vi "GetPropertiesArray.vi"(8 "error in (no error)":errorcluster, 11 "JSON Text":string="{\n    \"productNum\": 30929, \n    \"productName\": \"SLSC Module Prototype\",\n\n    \"vendorNum\": 4243, \n    \"vendorName\": \"National Instruments\",\n    \"vendorPrefix\": \"NI\",\n\n    \"capsVersion\": \"17.0.0f0\",\n    \"capsSpecVersion\": 2,\n    \"capsSpecOldestCompatibleVersion\": 1,\n\n    \"scales\": [\n       {\n           \"name\": \"PolynomialThermocouple\",\n           \"description-en\": \"Type J Thermocouple. https://www.omega.com/temperature/Z/pdf/z198-201.pdf\",\n           \"forwardCoeffs\": [\n              \n              \n              0.0,\n              1.978425e-2,\n              -2.001204e-7,\n              1.036969e-11,\n              -2.549687e-16,\n              3.585153e-21,\n              -5.344285e-26,\n              5.099890e-31\n           ],\n           \"reverseCoeffs\": [\n              \n              \n              0.0,\n              5.0381187815e1,\n              3.0475836930e-2,\n              -8.5681065720e-5,\n              1.3228195295e-7,\n              -1.7052958337e-10,\n              2.0948090697e-13,\n              -1.2538395336e-16,\n              1.5631725697e-20\n           ]\n       },\n       {\n           \"name\": \"PolynomialBoundaryConditions\",\n           \"description-en\": \"Simple 1st order polynomial scale for testing boundary conditions\",\n           \"forwardCoeffs\": [\n              3.0,\n              4.0\n           ],\n           \"reverseCoeffs\": [\n              -0.75,\n              0.25\n           ]\n       },\n       {\n           \"name\": \"TableRound\",\n           \"coercion\": \"RoundToNearest\",\n           \"table\": [\n               {\"scaled\": -6.0, \"unscaled\": -3.0},\n               {\"scaled\": 0.0, \"unscaled\": 0.0},\n               {\"scaled\": 6.0, \"unscaled\": 3.0}\n           ]\n       },\n       {\n           \"name\": \"TableInterpolate\",\n           \"coercion\": \"Interpolate\",\n           \"table\": [\n               {\"scaled\": -6.0, \"unscaled\": -3.0},\n               {\"scaled\": 0.0, \"unscaled\": 0.0},\n               {\"scaled\": 6.0, \"unscaled\": 3.0}\n           ]\n       },\n       {\n           \"name\": \"LinearDivideBy8\",\n           \"m\": 0.125,\n           \"b\": 0.0\n       },\n       {\n           \"name\": \"Times2Plus2\",\n           \"m\": 2.0,\n           \"b\": 2.0\n       },\n       {\n           \"name\": \"InvertBoolean\",\n           \"m\": -1.0,\n           \"b\": 1.0\n       },\n       {\n           \"name\": \"TableStrict\",\n           \"coercion\": \"Strict\",\n           \"table\": [\n               {\"scaled\": -88888.568101, \"unscaled\": 0.0},\n               {\"scaled\": -4.0, \"unscaled\": 1.0},\n               {\"scaled\": -1.0, \"unscaled\": 2.0},\n               {\"scaled\": 0.0, \"unscaled\": 3.0},\n               {\"scaled\": 6.59999999999, \"unscaled\": 4.0},\n               {\"scaled\": 6.6, \"unscaled\": 5.0},\n               {\"scaled\": 6.60000000001, \"unscaled\": 6.0},\n               {\"scaled\": 9999999999.59999, \"unscaled\": 7.0},\n               {\"scaled\": 9999999999.6, \"unscaled\": 8.0},\n               {\"scaled\": 9999999999.60001, \"unscaled\": 9.0}\n           ]\n       },\n       {\n          \"name\": \"TableStrict4Elements\",\n          \"coercion\": \"Strict\",\n           \"table\": [\n               {\"scaled\": -3.0, \"unscaled\": -6.0},\n               {\"scaled\": -2.0, \"unscaled\": -4.0},\n               {\"scaled\": 0.0, \"unscaled\": 0.0},\n               {\"scaled\": 1.0, \"unscaled\": 2.0}\n          ]\n       },\n       {\n          \"name\": \"TableStrict12Elements\",\n          \"coercion\": \"Strict\",\n          \"table\": [\n               {\"scaled\": -3.0, \"unscaled\": -6.0},\n               {\"scaled\": -2.0, \"unscaled\": -4.0},\n               {\"scaled\": 0.0, \"unscaled\": 0.0},\n               {\"scaled\": 1.0, \"unscaled\": 2.0},\n               {\"scaled\": 2.0, \"unscaled\": 4.0},\n               {\"scaled\": 3.0, \"unscaled\": 6.0},\n               {\"scaled\": 4.0, \"unscaled\": 8.0},\n               {\"scaled\": 5.0, \"unscaled\": 10.0},\n               {\"scaled\": 6.0, \"unscaled\": 12.0},\n               {\"scaled\": 7.0, \"unscaled\": 14.0},\n               {\"scaled\": 8.0, \"unscaled\": 16.0},\n               {\"scaled\": 9.0, \"unscaled\": 18.0}\n          ]\n       },\n       {\n          \n          \"name\": \"TableStrictTrueFalse\",\n          \"coercion\": \"Strict\",\n           \"table\": [\n               {\"scaled\": -4.0, \"unscaled\": -1.0},\n               {\"scaled\": -1.0, \"unscaled\": -3.0},\n               {\"scaled\": 0.0, \"unscaled\": 3.0},\n               {\"scaled\": 1.0, \"unscaled\": 0.0},\n               {\"scaled\": 2.0, \"unscaled\": -4.0},\n               {\"scaled\": 3.0, \"unscaled\": 12.0}\n          ]\n       },\n       {\n          \n          \"name\": \"TableStrictTrue\",\n          \"coercion\": \"Strict\",\n          \"table\": [\n               {\"scaled\": -4.0, \"unscaled\": -4.0},\n               {\"scaled\": -1.0, \"unscaled\": -1.0},\n               {\"scaled\": 1.0, \"unscaled\": 0.0},\n               {\"scaled\": 2.0, \"unscaled\": 2.0},\n               {\"scaled\": 3.0, \"unscaled\": 3.0}\n          ]\n       },\n       {\n          \n          \"name\": \"TableStrictFalse\",\n          \"coercion\": \"Strict\",\n          \"table\": [\n               {\"scaled\": -4.0, \"unscaled\": -4.0},\n               {\"scaled\": -1.0, \"unscaled\": -1.0},\n               {\"scaled\": 0.0, \"unscaled\": 0.0},\n               {\"scaled\": 2.0, \"unscaled\": 2.0},\n               {\"scaled\": 3.0, \"unscaled\": 3.0}\n          ]\n       },\n       {\n           \"name\": \"LinearMillisecondToSecond\",\n           \"m\": 0.001,\n           \"b\": 0.0\n       }\n    ],\n\n   \"enums\": [\n      {\n         \"name\": \"NI.LEDState\",\n         \"description-en\": \"This enum represents the state of LED\",\n         \"values\": [\n            {\n               \"name\": \"Off\",\n               \"value\": 0,\n               \"description-en\": \"The LED is off.\"\n            },\n            {\n               \"name\": \"On\",\n               \"value\": 1,\n               \"description-en\": \"The LED is on.\"\n            }\n         ]\n      },\n      {\n         \"name\": \"NI.EventDelay\",\n         \"description-en\": \"This enum determine how long to delay before setting the event interrupt.\",\n         \"values\": [\n            {\n               \"name\": \"TimeoutImmediately\",\n               \"value\": 0,\n               \"description-en\": \"Event to timeout immediately.\"\n            },\n            {\n               \"name\": \"TimeoutAfter50Millisecond\",\n               \"value\": 50,\n               \"description-en\": \"Event to timeout after 50 milliseconds.\"\n            },\n            {\n               \"name\": \"TimeoutAfter100Millisecond\",\n               \"value\": 100,\n               \"description-en\": \"Event to timeout after 100 milliseconds.\"\n            },\n            {\n               \"name\": \"TimeoutAfter150Millisecond\",\n               \"value\": 150,\n               \"description-en\": \"Event to timeout after 150 milliseconds.\"\n            },\n            {\n               \"name\": \"TimeoutAfter200Millisecond\",\n               \"value\": 200,\n               \"description-en\": \"Event to timeout after 200 milliseconds.\"\n            },\n            {\n               \"name\": \"TimeoutAfter250Millisecond\",\n               \"value\": 250,\n               \"description-en\": \"Event to timeout after 250 milliseconds.\"\n            }\n         ]\n      }\n   ],\n\n    \"registerMap\": {\n        \"registers\": [\n            {\n                \"name\": \"EventStartRegister\",\n                \"description-en\": \"Use to generate event.\",\n                \"access\": \"WriteOnly\",\n                \"address\": 512,\n                \"size\": 8,\n\n                \"bitfields\": [\n                    {\n                        \"name\": \"EventStart3\",\n                        \"description-en\": \"Starts event counter 3\",\n                        \"offset\": 3,\n                        \"size\": 1,\n                        \"strobe\": true\n                    },\n                    {\n                        \"name\": \"EventStart2\",\n                        \"description-en\": \"Starts event counter 2\",\n                        \"offset\": 2,\n                        \"size\": 1,\n                        \"strobe\": true\n                    },\n                    {\n                        \"name\": \"EventStart1\",\n                        \"description-en\": \"Starts event counter 1\",\n                        \"offset\": 1,\n                        \"size\": 1,\n                        \"strobe\": true\n                    },\n                    {\n                        \"name\": \"EventStart0\",\n                        \"description-en\": \"Starts event counter 0\",\n                        \"offset\": 0,\n                        \"size\": 1,\n                        \"strobe\": true\n                    }\n                ]\n            },\n            {\n                \"name\": \"EventCounter0\",\n                \"description-en\": \"Count down counter for generating an event.\",\n                \"access\": \"ReadWrite\",\n                \"address\": 528,\n                \"size\": 8,\n\n                \"initialValue\": 0,\n\n                \"bitfields\": [\n                    {\n                        \"name\": \"DelayInMilliseconds\",\n                        \"offset\": 0,\n                        \"size\": 8\n                    }\n                ]\n            },\n            {\n                \"name\": \"EventCounter1\",\n                \"description-en\": \"Count down counter for generating an event.\",\n                \"access\": \"ReadWrite\",\n                \"address\": 530,\n                \"size\": 8,\n\n                \"initialValue\": 0,\n\n                \"bitfields\": [\n                    {\n                        \"name\": \"DelayInMilliseconds\",\n                        \"offset\": 0,\n                        \"size\": 8\n                    }\n                ]\n            },\n            {\n                \"name\": \"EventCounter2\",\n                \"description-en\": \"Count down counter for generating an event.\",\n                \"access\": \"ReadWrite\",\n                \"address\": 532,\n                \"size\": 8,\n\n                \"initialValue\": 0,\n\n                \"bitfields\": [\n                    {\n                        \"name\": \"DelayInMilliseconds\",\n                        \"offset\": 0,\n                        \"size\": 8\n                    }\n                ]\n            },\n            {\n                \"name\": \"EventCounter3\",\n                \"description-en\": \"Count down counter for generating an event.\",\n                \"access\": \"ReadWrite\",\n                \"address\": 534,\n                \"size\": 8,\n\n                \"initialValue\": 0,\n\n                \"bitfields\": [\n                    {\n                        \"name\": \"DelayInMilliseconds\",\n                        \"offset\": 0,\n                        \"size\": 8\n                    }\n                ]\n            },\n            {\n                \"name\": \"InterruptStatus\",\n                \"description-en\": \"Shows the interrupt status\",\n                \"access\": \"ReadOnly\",\n                \"address\": 768,\n                \"size\": 8,\n\n                \"bitfields\": [\n                    {\n                        \"name\": \"ExternalIntStatus3\",\n                        \"description-en\": \"External interrupt status 3\",\n                        \"offset\": 7,\n                        \"size\": 1\n                    },\n                    {\n                        \"name\": \"ExternalIntStatus2\",\n                        \"description-en\": \"External interrupt status 2\",\n                        \"offset\": 6,\n                        \"size\": 1\n                    },\n                    {\n                        \"name\": \"ExternalIntStatus1\",\n                        \"description-en\": \"External interrupt status 1\",\n                        \"offset\": 5,\n                        \"size\": 1\n                    },\n                    {\n                        \"name\": \"ExternalIntStatus0\",\n                        \"description-en\": \"External interrupt status 0\",\n                        \"offset\": 4,\n                        \"size\": 1\n                    },\n                    {\n                        \"name\": \"EventIntStatus3\",\n                        \"description-en\": \"Event 3 interrupt status\",\n                        \"offset\": 3,\n                        \"size\": 1\n                    },\n                    {\n                        \"name\": \"EventIntStatus2\",\n                        \"description-en\": \"Event 2 interrupt status\",\n                        \"offset\": 2,\n                        \"size\": 1\n                    },\n                    {\n                        \"name\": \"EventIntStatus1\",\n                        \"description-en\": \"Event 1 interrupt status\",\n                        \"offset\": 1,\n                        \"size\": 1\n                    },\n                    {\n                        \"name\": \"EventIntStatus0\",\n                        \"description-en\": \"Event 0 interrupt status\",\n                        \"offset\": 0,\n                        \"size\": 1\n                    }\n                ]\n            },\n            {\n                \"name\": \"InterruptMask\",\n                \"description-en\": \"Shows the enabled interrupts\",\n                \"access\": \"ReadOnly\",\n                \"address\": 769,\n                \"size\": 8,\n\n                \"bitfields\": [\n                    {\n                        \"name\": \"ExternalIntMask3\",\n                        \"description-en\": \"External interrupt mask 3\",\n                        \"offset\": 7,\n                        \"size\": 1\n                    },\n                    {\n                        \"name\": \"ExternalIntMask2\",\n                        \"description-en\": \"External interrupt mask 2\",\n                        \"offset\": 6,\n                        \"size\": 1\n                    },\n                    {\n                        \"name\": \"ExternalIntMask1\",\n                        \"description-en\": \"External interrupt mask 1\",\n                        \"offset\": 5,\n                        \"size\": 1\n                    },\n                    {\n                        \"name\": \"ExternalIntMask0\",\n                        \"description-en\": \"External interrupt mask 0\",\n                        \"offset\": 4,\n                        \"size\": 1\n                    },\n                    {\n                        \"name\": \"EventIntMask3\",\n                        \"description-en\": \"Event 3 interrupt mask\",\n                        \"offset\": 3,\n                        \"size\": 1\n                    },\n                    {\n                        \"name\": \"EventIntMask2\",\n                        \"description-en\": \"Event 2 interrupt mask\",\n                        \"offset\": 2,\n                        \"size\": 1\n                    },\n                    {\n                        \"name\": \"EventIntMask1\",\n                        \"description-en\": \"Event 1 interrupt mask\",\n                        \"offset\": 1,\n                        \"size\": 1\n                    },\n                    {\n                        \"name\": \"EventIntMask0\",\n                        \"description-en\": \"Event 0 interrupt mask\",\n                        \"offset\": 0,\n                        \"size\": 1\n                    }\n                ]\n            },\n            {\n                \"name\": \"InterruptEnable\",\n                \"description-en\": \"Enable module interrupts support\",\n                \"access\": \"WriteOnly\",\n                \"address\": 770,\n                \"size\": 8,\n\n                \"bitfields\": [\n                    {\n                        \"name\": \"ExternalIntEnable3\",\n                        \"description-en\": \"Enable external interrupt 3\",\n                        \"offset\": 7,\n                        \"size\": 1,\n                        \"strobe\": true\n                    },\n                    {\n                        \"name\": \"ExternalIntEnable2\",\n                        \"description-en\": \"Enable external interrupt 2\",\n                        \"offset\": 6,\n                        \"size\": 1,\n                        \"strobe\": true\n                    },\n                    {\n                        \"name\": \"ExternalIntEnable1\",\n                        \"description-en\": \"Enable external interrupt 1\",\n                        \"offset\": 5,\n                        \"size\": 1,\n                        \"strobe\": true\n                    },\n                    {\n                        \"name\": \"ExternalIntEnable0\",\n                        \"description-en\": \"Enable external interrupt 0\",\n                        \"offset\": 4,\n                        \"size\": 1,\n                        \"strobe\": true\n                    },\n                    {\n                        \"name\": \"EventIntEnable3\",\n                        \"description-en\": \"Enable interrupt event 3\",\n                        \"offset\": 3,\n                        \"size\": 1,\n                        \"strobe\": true\n                    },\n                    {\n                        \"name\": \"EventIntEnable2\",\n                        \"description-en\": \"Enable interrupt event 2\",\n                        \"offset\": 2,\n                        \"size\": 1,\n                        \"strobe\": true\n                    },\n                    {\n                        \"name\": \"EventIntEnable1\",\n                        \"description-en\": \"Enable interrupt event 1\",\n                        \"offset\": 1,\n                        \"size\": 1,\n                        \"strobe\": true\n                    },\n                    {\n                        \"name\": \"EventIntEnable0\",\n                        \"description-en\": \"Enable interrupt event 0\",\n                        \"offset\": 0,\n                        \"size\": 1,\n                        \"strobe\": true\n                    }\n                ]\n            },\n            {\n                \"name\": \"InterruptDisable\",\n                \"description-en\": \"Disable module interrupts\",\n                \"access\": \"WriteOnly\",\n                \"address\": 771,\n                \"size\": 8,\n\n                \"bitfields\": [\n                    {\n                        \"name\": \"ExternalIntDisable3\",\n                        \"description-en\": \"Disable external interrupt 3\",\n                        \"offset\": 7,\n                        \"size\": 1,\n                        \"strobe\": true\n                    },\n                    {\n                        \"name\": \"ExternalIntDisable2\",\n                        \"description-en\": \"Disable external interrupt 2\",\n                        \"offset\": 6,\n                        \"size\": 1,\n                        \"strobe\": true\n                    },\n                    {\n                        \"name\": \"ExternalIntDisable1\",\n                        \"description-en\": \"Disable external interrupt 1\",\n                        \"offset\": 5,\n                        \"size\": 1,\n                        \"strobe\": true\n                    },\n                    {\n                        \"name\": \"ExternalIntDisable0\",\n                        \"description-en\": \"Disable external interrupt 0\",\n                        \"offset\": 4,\n                        \"size\": 1,\n                        \"strobe\": true\n                    },\n                    {\n                        \"name\": \"EventIntDisable3\",\n                        \"description-en\": \"Disable interrupt event 3\",\n                        \"offset\": 3,\n                        \"size\": 1,\n                        \"strobe\": true\n                    },\n                    {\n                        \"name\": \"EventIntDisable2\",\n                        \"description-en\": \"Disable interrupt event 2\",\n                        \"offset\": 2,\n                        \"size\": 1,\n                        \"strobe\": true\n                    },\n                    {\n                        \"name\": \"EventIntDisable1\",\n                        \"description-en\": \"Disable interrupt event 1\",\n                        \"offset\": 1,\n                        \"size\": 1,\n                        \"strobe\": true\n                    },\n                    {\n                        \"name\": \"EventIntDisable0\",\n                        \"description-en\": \"Disable interrupt event 0\",\n                        \"offset\": 0,\n                        \"size\": 1,\n                        \"strobe\": true\n                    }\n                ]\n            },\n            {\n                \"name\": \"InterruptAck\",\n                \"description-en\": \"Acknowledge module interrupts\",\n                \"access\": \"WriteOnly\",\n                \"address\": 772,\n                \"size\": 8,\n\n                \"bitfields\": [\n                    {\n                        \"name\": \"ExternalIntAck3\",\n                        \"description-en\": \"Acknowledge external interrupt 3\",\n                        \"offset\": 7,\n                        \"size\": 1,\n                        \"strobe\": true\n                    },\n                    {\n                        \"name\": \"ExternalIntAck2\",\n                        \"description-en\": \"Acknowledge external interrupt 2\",\n                        \"offset\": 6,\n                        \"size\": 1,\n                        \"strobe\": true\n                    },\n                    {\n                        \"name\": \"ExternalIntAck1\",\n                        \"description-en\": \"Acknowledge external interrupt 1\",\n                        \"offset\": 5,\n                        \"size\": 1,\n                        \"strobe\": true\n                    },\n                    {\n                        \"name\": \"ExternalIntAck0\",\n                        \"description-en\": \"Acknowledge external interrupt 0\",\n                        \"offset\": 4,\n                        \"size\": 1,\n                        \"strobe\": true\n                    },\n                    {\n                        \"name\": \"EventIntAck3\",\n                        \"description-en\": \"Acknowledge interrupt event 3\",\n                        \"offset\": 3,\n                        \"size\": 1,\n                        \"strobe\": true\n                    },\n                    {\n                        \"name\": \"EventIntAck2\",\n                        \"description-en\": \"Acknowledge interrupt event 2\",\n                        \"offset\": 2,\n                        \"size\": 1,\n                        \"strobe\": true\n                    },\n                    {\n                        \"name\": \"EventIntAck1\",\n                        \"description-en\": \"Acknowledge interrupt event 1\",\n                        \"offset\": 1,\n                        \"size\": 1,\n                        \"strobe\": true\n                    },\n                    {\n                        \"name\": \"EventIntAck0\",\n                        \"description-en\": \"Acknowledge interrupt event 0\",\n                        \"offset\": 0,\n                        \"size\": 1,\n                        \"strobe\": true\n                    }\n                ]\n            },\n            {\n                \"name\": \"Revision\",\n                \"description-en\": \"CPLD Date Code\",\n                \"access\": \"ReadOnly\",\n                \"address\": 2,\n                \"size\": 32,\n\n                \"bitfields\": [\n                    {\n                        \"name\": \"DateCode\",\n                        \"description-en\": \"CPLD bitfile date code\",\n                        \"offset\": 0,\n                        \"size\": 32\n                    }\n                ]\n            },\n            {\n                \"name\": \"FrontPanelLeds\",\n                \"description-en\": \"Controls front panel LEDs\",\n                \"access\": \"WriteOnly\",\n                \"address\": 1,\n                \"size\": 64,\n\n                \"initialValue\": 0,\n\n                \"bitfields\": [\n                    {\n                        \"name\": \"LedGreen2Enable\",\n                        \"description-en\": \"Turn on LED Green 2\",\n                        \"offset\": 6,\n                        \"size\": 1\n                    },\n                    {\n                        \"name\": \"LedGreen1Enable\",\n                        \"description-en\": \"Turn on LED Green 1\",\n                        \"offset\": 5,\n                        \"size\": 1\n                    },\n                    {\n                        \"name\": \"LedGreen0Enable\",\n                        \"description-en\": \"Turn on LED Green 0\",\n                        \"offset\": 4,\n                        \"size\": 1\n                    },\n                    {\n                        \"name\": \"LedRed2Enable\",\n                        \"description-en\": \"Turn on LED Red 2\",\n                        \"offset\": 2,\n                        \"size\": 1\n                    },\n                    {\n                        \"name\": \"LedRed1Enable\",\n                        \"description-en\": \"Turn on LED Red 1\",\n                        \"offset\": 1,\n                        \"size\": 1\n                    },\n                    {\n                        \"name\": \"LedRed0Enable\",\n                        \"description-en\": \"Turn on LED Red 0\",\n                        \"offset\": 0,\n                        \"size\": 1\n                    }\n                ]\n            },\n            {\n                \"name\": \"DebugScratch64\",\n                \"description-en\": \"64-bit Scratch register for debugging\",\n                \"access\": \"ReadWrite\",\n                \"address\": 256,\n                \"size\": 64,\n\n                \n                \"initialValue\": \"17940079176890708721\", \n\n                \"bitfields\": [\n                    {\n                        \"name\": \"Scratch64\",\n                        \"offset\": 0,\n                        \"size\": 64\n                    },\n                    {\n                        \"name\": \"ScratchI64\",\n                        \"offset\": 0,\n                        \"size\": 64,\n                        \"signed\": true\n                    },\n                    {\n                        \"name\": \"Scratch32\",\n                        \"offset\": 0,\n                        \"size\": 32\n                    },\n                    {\n                        \"name\": \"ScratchI32\",\n                        \"offset\": 0,\n                        \"size\": 32,\n                        \"signed\": true\n                    },\n                    {\n                        \"name\": \"Scratch16\",\n                        \"offset\": 0,\n                        \"size\": 16\n                    },\n                    {\n                        \"name\": \"ScratchI16\",\n                        \"offset\": 0,\n                        \"size\": 16,\n                        \"signed\": true\n                    },\n                    {\n                        \"name\": \"Scratch8\",\n                        \"offset\": 0,\n                        \"size\": 8\n                    },\n                    {\n                        \"name\": \"ScratchI8\",\n                        \"offset\": 0,\n                        \"size\": 8,\n                        \"signed\": true\n                    },\n                    {\n                        \"name\": \"ScratchBool\",\n                        \"offset\": 0,\n                        \"size\": 1\n                    }\n                ]\n            },\n            {\n                \"name\": \"DebugDipSwitch\",\n                \"description-en\": \"Reads the values of module SW1 DIP switches\",\n                \"access\": \"ReadOnly\",\n                \"address\": 257,\n                \"size\": 64,\n\n                \"bitfields\": [\n                    {\n                        \"name\": \"DipSwitch1\",\n                        \"description-en\": \"Reports the values of SW1 DIP switch 1\",\n                        \"offset\": 7,\n                        \"size\": 1\n                    },\n                    {\n                        \"name\": \"DipSwitch2\",\n                        \"description-en\": \"Reports the values of SW1 DIP switch 2\",\n                        \"offset\": 6,\n                        \"size\": 1\n                    },\n                    {\n                        \"name\": \"DipSwitch3\",\n                        \"description-en\": \"Reports the values of SW1 DIP switch 3\",\n                        \"offset\": 5,\n                        \"size\": 1\n                    },\n                    {\n                        \"name\": \"DipSwitch4\",\n                        \"description-en\": \"Reports the values of SW1 DIP switch 4\",\n                        \"offset\": 4,\n                        \"size\": 1\n                    },\n                    {\n                        \"name\": \"DipSwitch5\",\n                        \"description-en\": \"Reports the values of SW1 DIP switch 5\",\n                        \"offset\": 3,\n                        \"size\": 1\n                    },\n                    {\n                        \"name\": \"DipSwitch6\",\n                        \"description-en\": \"Reports the values of SW1 DIP switch 6\",\n                        \"offset\": 2,\n                        \"size\": 1\n                    },\n                    {\n                        \"name\": \"DipSwitch7\",\n                        \"description-en\": \"Reports the values of SW1 DIP switch 7\",\n                        \"offset\": 1,\n                        \"size\": 1\n                    },\n                    {\n                        \"name\": \"DipSwitch8\",\n                        \"description-en\": \"Reports the values of SW1 DIP switch 8\",\n                        \"offset\": 0,\n                        \"size\": 1\n                    }\n                ]\n            },\n            {\n                \"name\": \"DebugLeds\",\n                \"description-en\": \"Controls the blue LEDs adjacent to the CPLD\",\n                \"access\": \"ReadWrite\",\n                \"address\": 258,\n                \"size\": 64,\n\n                \"initialValue\" : 4, \n\n                \"bitfields\": [\n                    {\n                        \"name\": \"DebugLed0\",\n                        \"description-en\": \"Controls blue LED 0\",\n                        \"offset\": 0,\n                        \"size\": 1,\n                        \"strobe\": true \n                    },\n                    {\n                        \"name\": \"DebugLed1\",\n                        \"description-en\": \"Controls blue LED 1\",\n                        \"offset\": 1,\n                        \"size\": 1\n                    },\n                    {\n                        \"name\": \"DebugLed2\",\n                        \"description-en\": \"Controls blue LED 2\",\n                        \"offset\": 2,\n                        \"size\": 1\n                    },\n                    {\n                        \"name\": \"DebugLed3\",\n                        \"description-en\": \"Controls blue LED 3\",\n                        \"offset\": 3,\n                        \"size\": 1\n                    }\n                ]\n            },\n            {\n                \"name\": \"DebugScratch32\",\n                \"description-en\": \"32-bit Scratch register for debugging\",\n                \"access\": \"ReadWrite\",\n                \"address\": 280,\n                \"size\": 32,\n\n                \n                \"initialValue\": 4109628145, \n\n                \"bitfields\": [\n                    {\n                        \"name\": \"Scratch32\",\n                        \"offset\": 0,\n                        \"size\": 32\n                    },\n                    {\n                        \"name\": \"ScratchI32\",\n                        \"offset\": 0,\n                        \"size\": 32,\n                        \"signed\": true\n                    },\n                    {\n                        \"name\": \"Scratch16\",\n                        \"offset\": 0,\n                        \"size\": 16\n                    },\n                    {\n                        \"name\": \"ScratchI16\",\n                        \"offset\": 0,\n                        \"size\": 16,\n                        \"signed\": true\n                    },\n                    {\n                        \"name\": \"Scratch8\",\n                        \"offset\": 0,\n                        \"size\": 8\n                    },\n                    {\n                        \"name\": \"ScratchI8\",\n                        \"offset\": 0,\n                        \"size\": 8,\n                        \"signed\": true\n                    },\n                    {\n                        \"name\": \"ScratchBool\",\n                        \"offset\": 0,\n                        \"size\": 1\n                    }\n                ]\n            },\n            {\n                \"name\": \"DebugScratch16\",\n                \"description-en\": \"16-bit Scratch register for debugging\",\n                \"access\": \"ReadWrite\",\n                \"address\": 284,\n                \"size\": 16,\n\n                \n                \"initialValue\": 62193, \n\n                \"bitfields\": [\n                    {\n                        \"name\": \"Scratch16\",\n                        \"offset\": 0,\n                        \"size\": 16\n                    },\n                    {\n                        \"name\": \"ScratchI16\",\n                        \"offset\": 0,\n                        \"size\": 16,\n                        \"signed\": true\n                    },\n                    {\n                        \"name\": \"Scratch8\",\n                        \"offset\": 0,\n                        \"size\": 8\n                    },\n                    {\n                        \"name\": \"ScratchI8\",\n                        \"offset\": 0,\n                        \"size\": 8,\n                        \"signed\": true\n                    },\n                    {\n                        \"name\": \"ScratchBool\",\n                        \"offset\": 0,\n                        \"size\": 1\n                    }\n                ]\n            },\n            {\n                \"name\": \"DebugScratch8\",\n                \"description-en\": \"8-bit Scratch register for debugging\",\n                \"access\": \"ReadWrite\",\n                \"address\": 286,\n                \"size\": 8,\n\n                \n                \"initialValue\": 241, \n\n                \"bitfields\": [\n                    {\n                        \"name\": \"ScratchBool\",\n                        \"offset\": 0,\n                        \"size\": 1\n                    },\n                    {\n                        \"name\": \"Scratch8\",\n                        \"offset\": 0,\n                        \"size\": 8\n                    },\n                    {\n                        \"name\": \"ScratchI8\",\n                        \"offset\": 0,\n                        \"size\": 8,\n                        \"signed\": true\n                    }\n                ]\n            },\n            {\n                \"name\": \"ComplianceTestRegister\",\n                \"description-en\": \"MDK-required scratchpad register\",\n                \"access\": \"ReadWrite\",\n                \"address\": 32512,\n                \"size\": 8\n            },\n            {\n                \"name\": \"ComplianceTestPatternRegister\",\n                \"description-en\": \"MDK-required register which should always return 0xAA55F733CC08D24B\",\n                \"access\": \"ReadOnly\",\n                \"address\": 32520,\n                \"size\": 64\n            }\n         ],\n         \"interrupts\" : [\n            {\n               \"name\": \"EventInt0\",\n               \"description-en\": \"Event Interrupt 0\",\n               \"enableBitfield\": \"InterruptEnable/EventIntEnable0\",\n               \"disableBitfield\": \"InterruptDisable/EventIntDisable0\",\n               \"ackBitfield\": \"InterruptAck/EventIntAck0\",\n               \"statusBitfield\": \"InterruptStatus/EventIntStatus0\"\n            },\n            {\n               \"name\": \"EventInt1\",\n               \"description-en\": \"Event Interrupt 1\",\n               \"enableBitfield\": \"InterruptEnable/EventIntEnable1\",\n               \"disableBitfield\": \"InterruptDisable/EventIntDisable1\",\n               \"ackBitfield\": \"InterruptAck/EventIntAck1\",\n               \"statusBitfield\": \"InterruptStatus/EventIntStatus1\"\n            },\n            {\n               \"name\": \"EventInt2\",\n               \"description-en\": \"Event Interrupt 2\",\n               \"enableBitfield\": \"InterruptEnable/EventIntEnable2\",\n               \"disableBitfield\": \"InterruptDisable/EventIntDisable2\",\n               \"ackBitfield\": \"InterruptAck/EventIntAck2\",\n               \"statusBitfield\": \"InterruptStatus/EventIntStatus2\"\n            },\n            {\n               \"name\": \"EventInt3\",\n               \"description-en\": \"Event Interrupt 3\",\n               \"enableBitfield\": \"InterruptEnable/EventIntEnable3\",\n               \"disableBitfield\": \"InterruptDisable/EventIntDisable3\",\n               \"ackBitfield\": \"InterruptAck/EventIntAck3\",\n               \"statusBitfield\": \"InterruptStatus/EventIntStatus3\"\n            },\n            {\n               \"name\": \"ExternalInt0\",\n               \"description-en\": \"External Interrupt 0\",\n               \"enableBitfield\": \"InterruptEnable/ExternalIntEnable0\",\n               \"disableBitfield\": \"InterruptDisable/ExternalIntDisable0\",\n               \"ackBitfield\": \"InterruptAck/ExternalIntAck0\",\n               \"statusBitfield\": \"InterruptStatus/ExternalIntStatus0\"\n            },\n            {\n               \"name\": \"ExternalInt1\",\n               \"description-en\": \"External Interrupt 1\",\n               \"enableBitfield\": \"InterruptEnable/ExternalIntEnable1\",\n               \"disableBitfield\": \"InterruptDisable/ExternalIntDisable1\",\n               \"ackBitfield\": \"InterruptAck/ExternalIntAck1\",\n               \"statusBitfield\": \"InterruptStatus/ExternalIntStatus1\"\n            },\n            {\n               \"name\": \"ExternalInt2\",\n               \"description-en\": \"External Interrupt 2\",\n               \"enableBitfield\": \"InterruptEnable/ExternalIntEnable2\",\n               \"disableBitfield\": \"InterruptDisable/ExternalIntDisable2\",\n               \"ackBitfield\": \"InterruptAck/ExternalIntAck2\",\n               \"statusBitfield\": \"InterruptStatus/ExternalIntStatus2\"\n            },\n            {\n               \"name\": \"ExternalInt3\",\n               \"description-en\": \"External Interrupt 3\",\n               \"enableBitfield\": \"InterruptEnable/ExternalIntEnable3\",\n               \"disableBitfield\": \"InterruptDisable/ExternalIntDisable3\",\n               \"ackBitfield\": \"InterruptAck/ExternalIntAck3\",\n               \"statusBitfield\": \"InterruptStatus/ExternalIntStatus3\"\n            }\n         ]\n    },\n\n    \"commands\": [\n        {\n            \"name\": \"NI.EnableLed0Immediate\",\n            \"description-en\": \"Enable LED 0 and complete immediately\",\n            \"documentation-en\": \"Enable LED 0 and complete immediately (doc)\",\n            \"startBitfield\": \"DebugLeds/DebugLed0\"\n        },\n        {\n            \"name\": \"NI.EnableLed0Delay\",\n            \"description-en\": \"Enable LED 0 and delay 5 second\",\n            \"documentation-en\": \"Enable LED 0 and delay 5 second (doc)\",\n            \"startBitfield\": \"DebugLeds/DebugLed0\",\n            \"waitTimeInMs\": 5000\n        },\n        {\n            \"name\": \"NI.EnableLed0Poll\",\n            \"description-en\": \"Enable LED 0 and wait until DIP switch 1 enabled\",\n            \"documentation-en\": \"Enable LED 0 and wait until DIP switch 1 enabled (doc)\",\n            \"startBitfield\": \"DebugLeds/DebugLed0\",\n            \"doneBitfield\": \"DebugDipSwitch/DipSwitch1\",\n            \"doneTimeoutInMs\": 5000\n        },\n        {\n            \"name\": \"NI.Event0TimerExpirationInterrupt\",\n            \"description-en\": \"Start event 0 timer and wait until the expiration interrupt\",\n            \"documentation-en\": \"Start event 0 timer and wait until the expiration interrupt\",\n            \"startBitfield\": \"EventStartRegister/EventStart0\",\n            \"doneInterrupt\": \"EventInt0\",\n            \"doneTimeoutInMs\": 5000\n        },\n        {\n            \"name\": \"NI.Event1TimerExpirationInterrupt\",\n            \"description-en\": \"Start event 1 timer and wait until the expiration interrupt\",\n            \"documentation-en\": \"Start event 1 timer and wait until the expiration interrupt\",\n            \"startBitfield\": \"EventStartRegister/EventStart1\",\n            \"doneInterrupt\": \"EventInt1\",\n            \"doneTimeoutInMs\": 5000\n        },\n        {\n            \"name\": \"NI.Event2TimerExpirationInterrupt\",\n            \"description-en\": \"Start event 2 timer and wait until the expiration interrupt\",\n            \"documentation-en\": \"Start event 2 timer and wait until the expiration interrupt\",\n            \"startBitfield\": \"EventStartRegister/EventStart2\",\n            \"doneInterrupt\": \"EventInt2\",\n            \"doneTimeoutInMs\": 5000\n        },\n        {\n            \"name\": \"NI.Event3TimerExpirationInterrupt\",\n            \"description-en\": \"Start event 3 timer and wait until the expiration interrupt\",\n            \"documentation-en\": \"Start event 3 timer and wait until the expiration interrupt\",\n            \"startBitfield\": \"EventStartRegister/EventStart3\",\n            \"doneInterrupt\": \"EventInt3\",\n            \"doneTimeoutInMs\": 5000\n        }\n    ],\n\n    \"physicalChannels\": [\n        {\n            \"name\": \"LED0\",\n            \"properties\": [\n                {\n                   \"name\": \"NI.ChannelName\",\n                   \"dataType\": \"String\",\n                   \"value\": \"LED0\"\n                },\n                {\n                    \"name\": \"NI.RedBool\",\n                    \"dataType\": \"Bool\",\n                    \"access\": \"WriteOnly\",\n                    \"bitfield\": \"FrontPanelLeds/LedRed0Enable\"\n                },\n                {\n                    \"name\": \"NI.GreenBool\",\n                    \"dataType\": \"Bool\",\n                    \"access\": \"WriteOnly\",\n                    \"bitfield\": \"FrontPanelLeds/LedGreen0Enable\"\n                },\n                {\n                    \"name\": \"NI.RedEnum\",\n                    \"dataType\": \"NI.LEDState\",\n                    \"access\": \"WriteOnly\",\n                    \"bitfield\": \"FrontPanelLeds/LedRed0Enable\"\n                },\n                {\n                    \"name\": \"NI.GreenEnum\",\n                    \"dataType\": \"NI.LEDState\",\n                    \"access\": \"WriteOnly\",\n                    \"bitfield\": \"FrontPanelLeds/LedGreen0Enable\"\n                }\n            ]\n        },\n        {\n            \"name\": \"LED1\",\n            \"properties\": [\n                {\n                   \"name\": \"NI.ChannelName\",\n                   \"dataType\": \"String\",\n                   \"value\": \"LED1\"\n                },\n                {\n                    \"name\": \"NI.RedBool\",\n                    \"dataType\": \"Bool\",\n                    \"access\": \"WriteOnly\",\n                    \"bitfield\": \"FrontPanelLeds/LedRed1Enable\"\n                },\n                {\n                    \"name\": \"NI.GreenBool\",\n                    \"dataType\": \"Bool\",\n                    \"access\": \"WriteOnly\",\n                    \"bitfield\": \"FrontPanelLeds/LedGreen1Enable\"\n                },\n                {\n                    \"name\": \"NI.RedEnum\",\n                    \"dataType\": \"NI.LEDState\",\n                    \"access\": \"WriteOnly\",\n                    \"bitfield\": \"FrontPanelLeds/LedRed1Enable\"\n                },\n                {\n                    \"name\": \"NI.GreenEnum\",\n                    \"dataType\": \"NI.LEDState\",\n                    \"access\": \"WriteOnly\",\n                    \"bitfield\": \"FrontPanelLeds/LedGreen1Enable\"\n                }\n            ]\n        },\n        {\n            \"name\": \"LED2\",\n            \"properties\": [\n                {\n                   \"name\": \"NI.ChannelName\",\n                   \"dataType\": \"String\",\n                   \"value\": \"LED2\"\n                },\n                {\n                    \"name\": \"NI.RedBool\",\n                    \"dataType\": \"Bool\",\n                    \"access\": \"WriteOnly\",\n                    \"bitfield\": \"FrontPanelLeds/LedRed2Enable\"\n                },\n                {\n                    \"name\": \"NI.GreenBool\",\n                    \"dataType\": \"Bool\",\n                    \"access\": \"WriteOnly\",\n                    \"bitfield\": \"FrontPanelLeds/LedGreen2Enable\"\n                },\n                {\n                    \"name\": \"NI.RedEnum\",\n                    \"dataType\": \"NI.LEDState\",\n                    \"access\": \"WriteOnly\",\n                    \"bitfield\": \"FrontPanelLeds/LedRed2Enable\"\n                },\n                {\n                    \"name\": \"NI.GreenEnum\",\n                    \"dataType\": \"NI.LEDState\",\n                    \"access\": \"WriteOnly\",\n                    \"bitfield\": \"FrontPanelLeds/LedGreen2Enable\"\n                }\n            ]\n        },\n        {\n            \"name\": \"EventCounter0\",\n            \"properties\": [\n                {\n                   \"name\": \"NI.ChannelName\",\n                   \"dataType\": \"String\",\n                   \"value\": \"EventCounter0\"\n                },\n                {\n                    \"name\": \"NI.EventCounter.DelayInMs\",\n                    \"dataType\": \"UInt32\",\n                    \"access\": \"ReadWrite\",\n                    \"bitfield\": \"EventCounter0/DelayInMilliseconds\",\n                    \"max\": 255\n                },\n                {\n                    \"name\": \"NI.EventCounter.DelayInSec\",\n                     \"dataType\": \"Double\",\n                     \"access\": \"ReadWrite\",\n                     \"bitfield\": \"EventCounter0/DelayInMilliseconds\",\n                     \"scale\": \"LinearMillisecondToSecond\",\n                     \"min\": 0.0,\n                     \"max\": 0.255\n                },\n                {\n                    \"name\": \"NI.EventCounter.DelayEnum\",\n                     \"dataType\": \"NI.EventDelay\",\n                     \"access\": \"ReadWrite\",\n                     \"bitfield\": \"EventCounter0/DelayInMilliseconds\"\n                },\n                {\n                    \"name\": \"NI.EventCounter.Done\",\n                    \"dataType\": \"Bool\",\n                    \"access\": \"ReadOnly\",\n                    \"bitfield\": \"InterruptStatus/EventIntStatus0\"\n                },\n                {\n                    \"name\": \"NI.EventCounter.Armed\",\n                    \"dataType\": \"Bool\",\n                    \"access\": \"ReadOnly\",\n                    \"bitfield\": \"InterruptMask/EventIntMask0\"\n                },\n                {\n                    \"name\": \"NI.EventCounter.Ack\",\n                    \"dataType\": \"Bool\",\n                    \"access\": \"WriteOnly\",\n                    \"bitfield\": \"InterruptAck/EventIntAck0\"\n                },\n                {\n                    \"name\": \"NI.EventCounter.Start\",\n                    \"dataType\": \"Bool\",\n                    \"access\": \"WriteOnly\",\n                    \"bitfield\": \"EventStartRegister/EventStart0\"\n                }\n            ],\n            \"commands\" : [\n                 {\n                     \"name\": \"NI.EventCounter.Run\",\n                     \"description-en\": \"Start event timer and wait until the expiration interrupt\",\n                     \"documentation-en\": \"Start event timer and wait until the expiration interrupt\",\n                     \"startBitfield\": \"EventStartRegister/EventStart0\",\n                     \"doneInterrupt\": \"EventInt0\",\n                     \"doneTimeoutInMs\": 5000\n                 },\n                 {\n                     \"name\": \"NI.EventCounter.RunAsync\",\n                     \"description-en\": \"Start event timer without waiting the expiration interrupt\",\n                     \"documentation-en\": \"Start event timer without waiting the expiration interrupt\",\n                     \"startBitfield\": \"EventStartRegister/EventStart0\"\n                 },\n                 {\n                     \"name\": \"NI.EventCounter.RunAndPoll\",\n                     \"description-en\": \"Start event timer and poll the event IntStatus bit for completion\",\n                     \"documentation-en\": \"Start event timer and poll the event IntStatus bit for completion\",\n                     \"startBitfield\": \"EventStartRegister/EventStart0\",\n                     \"doneBitfield\": \"InterruptStatus/EventIntStatus0\",\n                     \"doneTimeoutInMs\": 5000\n                 }\n            ]\n        },\n        {\n            \"name\": \"EventCounter1\",\n            \"properties\": [\n                {\n                   \"name\": \"NI.ChannelName\",\n                   \"dataType\": \"String\",\n                   \"value\": \"EventCounter1\"\n                },\n                {\n                    \"name\": \"NI.EventCounter.DelayInMs\",\n                    \"dataType\": \"UInt32\",\n                    \"access\": \"ReadWrite\",\n                    \"bitfield\": \"EventCounter1/DelayInMilliseconds\",\n                    \"max\": 255\n                },\n                {\n                    \"name\": \"NI.EventCounter.DelayInSec\",\n                     \"dataType\": \"Double\",\n                     \"access\": \"ReadWrite\",\n                     \"bitfield\": \"EventCounter1/DelayInMilliseconds\",\n                     \"scale\": \"LinearMillisecondToSecond\",\n                     \"min\": 0.0,\n                     \"max\": 0.255\n                },\n                {\n                    \"name\": \"NI.EventCounter.DelayEnum\",\n                     \"dataType\": \"NI.EventDelay\",\n                     \"access\": \"ReadWrite\",\n                     \"bitfield\": \"EventCounter1/DelayInMilliseconds\"\n                },\n                {\n                    \"name\": \"NI.EventCounter.Done\",\n                    \"dataType\": \"Bool\",\n                    \"access\": \"ReadOnly\",\n                    \"bitfield\": \"InterruptStatus/EventIntStatus1\"\n                },\n                {\n                    \"name\": \"NI.EventCounter.Armed\",\n                    \"dataType\": \"Bool\",\n                    \"access\": \"ReadOnly\",\n                    \"bitfield\": \"InterruptMask/EventIntMask1\"\n                },\n                {\n                    \"name\": \"NI.EventCounter.Ack\",\n                    \"dataType\": \"Bool\",\n                    \"access\": \"WriteOnly\",\n                    \"bitfield\": \"InterruptAck/EventIntAck1\"\n                },\n                {\n                    \"name\": \"NI.EventCounter.Start\",\n                    \"dataType\": \"Bool\",\n                    \"access\": \"WriteOnly\",\n                    \"bitfield\": \"EventStartRegister/EventStart1\"\n                }\n            ],\n            \"commands\" : [\n                 {\n                     \"name\": \"NI.EventCounter.Run\",\n                     \"description-en\": \"Start event timer and wait until the expiration interrupt\",\n                     \"documentation-en\": \"Start event timer and wait until the expiration interrupt\",\n                     \"startBitfield\": \"EventStartRegister/EventStart1\",\n                     \"doneInterrupt\": \"EventInt1\",\n                     \"doneTimeoutInMs\": 5000\n                 },\n                 {\n                     \"name\": \"NI.EventCounter.RunAsync\",\n                     \"description-en\": \"Start event timer without waiting the expiration interrupt\",\n                     \"documentation-en\": \"Start event timer without waiting the expiration interrupt\",\n                     \"startBitfield\": \"EventStartRegister/EventStart1\"\n                 },\n                 {\n                     \"name\": \"NI.EventCounter.RunAndPoll\",\n                     \"description-en\": \"Start event timer and poll the event IntStatus bit for completion\",\n                     \"documentation-en\": \"Start event timer and poll the event IntStatus bit for completion\",\n                     \"startBitfield\": \"EventStartRegister/EventStart1\",\n                     \"doneBitfield\": \"InterruptStatus/EventIntStatus1\",\n                     \"doneTimeoutInMs\": 5000\n                 }\n            ]\n        },\n        {\n            \"name\": \"EventCounter2\",\n            \"properties\": [\n                {\n                   \"name\": \"NI.ChannelName\",\n                   \"dataType\": \"String\",\n                   \"value\": \"EventCounter2\"\n                },\n                {\n                    \"name\": \"NI.EventCounter.DelayInMs\",\n                    \"dataType\": \"UInt32\",\n                    \"access\": \"ReadWrite\",\n                    \"bitfield\": \"EventCounter2/DelayInMilliseconds\",\n                    \"max\": 255\n                },\n                {\n                    \"name\": \"NI.EventCounter.DelayInSec\",\n                     \"dataType\": \"Double\",\n                     \"access\": \"ReadWrite\",\n                     \"bitfield\": \"EventCounter2/DelayInMilliseconds\",\n                     \"scale\": \"LinearMillisecondToSecond\",\n                     \"min\": 0.0,\n                     \"max\": 0.255\n                },\n                {\n                    \"name\": \"NI.EventCounter.DelayEnum\",\n                     \"dataType\": \"NI.EventDelay\",\n                     \"access\": \"ReadWrite\",\n                     \"bitfield\": \"EventCounter2/DelayInMilliseconds\"\n                },\n                {\n                    \"name\": \"NI.EventCounter.Done\",\n                    \"dataType\": \"Bool\",\n                    \"access\": \"ReadOnly\",\n                    \"bitfield\": \"InterruptStatus/EventIntStatus2\"\n                },\n                {\n                    \"name\": \"NI.EventCounter.Armed\",\n                    \"dataType\": \"Bool\",\n                    \"access\": \"ReadOnly\",\n                    \"bitfield\": \"InterruptMask/EventIntMask2\"\n                },\n                {\n                    \"name\": \"NI.EventCounter.Ack\",\n                    \"dataType\": \"Bool\",\n                    \"access\": \"WriteOnly\",\n                    \"bitfield\": \"InterruptAck/EventIntAck2\"\n                },\n                {\n                    \"name\": \"NI.EventCounter.Start\",\n                    \"dataType\": \"Bool\",\n                    \"access\": \"WriteOnly\",\n                    \"bitfield\": \"EventStartRegister/EventStart2\"\n                }\n            ],\n            \"commands\" : [\n                 {\n                     \"name\": \"NI.EventCounter.Run\",\n                     \"description-en\": \"Start event timer and wait until the expiration interrupt\",\n                     \"documentation-en\": \"Start event timer and wait until the expiration interrupt\",\n                     \"startBitfield\": \"EventStartRegister/EventStart2\",\n                     \"doneInterrupt\": \"EventInt2\",\n                     \"doneTimeoutInMs\": 5000\n                 },\n                 {\n                     \"name\": \"NI.EventCounter.RunAsync\",\n                     \"description-en\": \"Start event timer without waiting the expiration interrupt\",\n                     \"documentation-en\": \"Start event timer without waiting the expiration interrupt\",\n                     \"startBitfield\": \"EventStartRegister/EventStart2\"\n                 },\n                 {\n                     \"name\": \"NI.EventCounter.RunAndPoll\",\n                     \"description-en\": \"Start event timer and poll the event IntStatus bit for completion\",\n                     \"documentation-en\": \"Start event timer and poll the event IntStatus bit for completion\",\n                     \"startBitfield\": \"EventStartRegister/EventStart2\",\n                     \"doneBitfield\": \"InterruptStatus/EventIntStatus2\",\n                     \"doneTimeoutInMs\": 5000\n                 }\n            ]\n        },\n        {\n            \"name\": \"EventCounter3\",\n            \"properties\": [\n                {\n                   \"name\": \"NI.ChannelName\",\n                   \"dataType\": \"String\",\n                   \"value\": \"EventCounter3\"\n                },\n                {\n                    \"name\": \"NI.EventCounter.DelayInMs\",\n                    \"dataType\": \"UInt32\",\n                    \"access\": \"ReadWrite\",\n                    \"bitfield\": \"EventCounter3/DelayInMilliseconds\",\n                    \"max\": 255\n                },\n                {\n                    \"name\": \"NI.EventCounter.DelayInSec\",\n                     \"dataType\": \"Double\",\n                     \"access\": \"ReadWrite\",\n                     \"bitfield\": \"EventCounter3/DelayInMilliseconds\",\n                     \"scale\": \"LinearMillisecondToSecond\",\n                     \"min\": 0.0,\n                     \"max\": 0.255\n                },\n                {\n                    \"name\": \"NI.EventCounter.DelayEnum\",\n                     \"dataType\": \"NI.EventDelay\",\n                     \"access\": \"ReadWrite\",\n                     \"bitfield\": \"EventCounter3/DelayInMilliseconds\"\n                },\n                {\n                    \"name\": \"NI.EventCounter.Done\",\n                    \"dataType\": \"Bool\",\n                    \"access\": \"ReadOnly\",\n                    \"bitfield\": \"InterruptStatus/EventIntStatus3\"\n                },\n                {\n                    \"name\": \"NI.EventCounter.Armed\",\n                    \"dataType\": \"Bool\",\n                    \"access\": \"ReadOnly\",\n                    \"bitfield\": \"InterruptMask/EventIntMask3\"\n                },\n                {\n                    \"name\": \"NI.EventCounter.Ack\",\n                    \"dataType\": \"Bool\",\n                    \"access\": \"WriteOnly\",\n                    \"bitfield\": \"InterruptAck/EventIntAck3\"\n                },\n                {\n                    \"name\": \"NI.EventCounter.Start\",\n                    \"dataType\": \"Bool\",\n                    \"access\": \"WriteOnly\",\n                    \"bitfield\": \"EventStartRegister/EventStart3\"\n                }\n            ],\n            \"commands\" : [\n                 {\n                     \"name\": \"NI.EventCounter.Run\",\n                     \"description-en\": \"Start event timer and wait until the expiration interrupt\",\n                     \"documentation-en\": \"Start event timer and wait until the expiration interrupt\",\n                     \"startBitfield\": \"EventStartRegister/EventStart3\",\n                     \"doneInterrupt\": \"EventInt3\",\n                     \"doneTimeoutInMs\": 5000\n                 },\n                 {\n                     \"name\": \"NI.EventCounter.RunAsync\",\n                     \"description-en\": \"Start event timer without waiting the expiration interrupt\",\n                     \"documentation-en\": \"Start event timer without waiting the expiration interrupt\",\n                     \"startBitfield\": \"EventStartRegister/EventStart3\"\n                 },\n                 {\n                     \"name\": \"NI.EventCounter.RunAndPoll\",\n                     \"description-en\": \"Start event timer and poll the event IntStatus bit for completion\",\n                     \"documentation-en\": \"Start event timer and poll the event IntStatus bit for completion\",\n                     \"startBitfield\": \"EventStartRegister/EventStart3\",\n                     \"doneBitfield\": \"InterruptStatus/EventIntStatus3\",\n                     \"doneTimeoutInMs\": 5000\n                 }\n            ]\n        },\n        {\n            \"name\": \"ExternalInterrupt0\",\n            \"properties\": [\n                {\n                   \"name\": \"NI.ChannelName\",\n                   \"dataType\": \"String\",\n                   \"value\": \"ExternalInterrupt0\"\n                },\n                {\n                    \"name\": \"NI.ExternalInterrupt.Done\",\n                    \"dataType\": \"Bool\",\n                    \"access\": \"ReadOnly\",\n                    \"bitfield\": \"InterruptStatus/ExternalIntStatus0\"\n                },\n                {\n                    \"name\": \"NI.ExternalInterrupt.Armed\",\n                    \"dataType\": \"Bool\",\n                    \"access\": \"ReadOnly\",\n                    \"bitfield\": \"InterruptMask/ExternalIntMask0\"\n                },\n                {\n                    \"name\": \"NI.ExternalInterrupt.Enable\",\n                    \"dataType\": \"Bool\",\n                    \"access\": \"WriteOnly\",\n                    \"bitfield\": \"InterruptEnable/ExternalIntEnable0\"\n                },\n                {\n                    \"name\": \"NI.ExternalInterrupt.Disable\",\n                    \"dataType\": \"Bool\",\n                    \"access\": \"WriteOnly\",\n                    \"bitfield\": \"InterruptDisable/ExternalIntDisable0\"\n                },\n                {\n                    \"name\": \"NI.ExternalInterrupt.Ack\",\n                    \"dataType\": \"Bool\",\n                    \"access\": \"WriteOnly\",\n                    \"bitfield\": \"InterruptAck/ExternalIntAck0\"\n                }\n            ],\n            \"commands\" : [\n                 {\n                     \"name\": \"NI.ExternalInterrupt.Wait\",\n                     \"description-en\": \"Wait for the external interrupt\",\n                     \"documentation-en\": \"Wait for the external interrupt\",\n                     \"startBitfield\": \"InterruptAck/ExternalIntAck0\", \n                     \"doneInterrupt\": \"ExternalInt0\",\n                     \"doneTimeoutInMs\": 60000\n                 },\n                 {\n                     \"name\": \"NI.ExternalInterrupt.Poll\",\n                     \"description-en\": \"Poll for the external interrupt line to be asserted\",\n                     \"documentation-en\": \"Poll for the external interrupt line to be asserted\",\n                     \"startBitfield\": \"InterruptAck/ExternalIntAck0\", \n                     \"doneBitfield\": \"InterruptStatus/ExternalIntStatus0\",\n                     \"doneTimeoutInMs\": 60000\n                 }\n            ]\n        },\n        {\n            \"name\": \"ExternalInterrupt1\",\n            \"properties\": [\n                {\n                   \"name\": \"NI.ChannelName\",\n                   \"dataType\": \"String\",\n                   \"value\": \"ExternalInterrupt1\"\n                },\n                {\n                    \"name\": \"NI.ExternalInterrupt.Done\",\n                    \"dataType\": \"Bool\",\n                    \"access\": \"ReadOnly\",\n                    \"bitfield\": \"InterruptStatus/ExternalIntStatus1\"\n                },\n                {\n                    \"name\": \"NI.ExternalInterrupt.Armed\",\n                    \"dataType\": \"Bool\",\n                    \"access\": \"ReadOnly\",\n                    \"bitfield\": \"InterruptMask/ExternalIntMask1\"\n                },\n                {\n                    \"name\": \"NI.ExternalInterrupt.Enable\",\n                    \"dataType\": \"Bool\",\n                    \"access\": \"WriteOnly\",\n                    \"bitfield\": \"InterruptEnable/ExternalIntEnable1\"\n                },\n                {\n                    \"name\": \"NI.ExternalInterrupt.Disable\",\n                    \"dataType\": \"Bool\",\n                    \"access\": \"WriteOnly\",\n                    \"bitfield\": \"InterruptDisable/ExternalIntDisable1\"\n                },\n                {\n                    \"name\": \"NI.ExternalInterrupt.Ack\",\n                    \"dataType\": \"Bool\",\n                    \"access\": \"WriteOnly\",\n                    \"bitfield\": \"InterruptAck/ExternalIntAck1\"\n                }\n            ],\n            \"commands\" : [\n                 {\n                     \"name\": \"NI.ExternalInterrupt.Wait\",\n                     \"description-en\": \"Wait for the external interrupt\",\n                     \"documentation-en\": \"Wait for the external interrupt\",\n                     \"startBitfield\": \"InterruptAck/ExternalIntAck1\", \n                     \"doneInterrupt\": \"ExternalInt1\",\n                     \"doneTimeoutInMs\": 60000\n                 },\n                 {\n                     \"name\": \"NI.ExternalInterrupt.Poll\",\n                     \"description-en\": \"Poll for the external interrupt line to be asserted\",\n                     \"documentation-en\": \"Poll for the external interrupt line to be asserted\",\n                     \"startBitfield\": \"InterruptAck/ExternalIntAck1\", \n                     \"doneBitfield\": \"InterruptStatus/ExternalIntStatus1\",\n                     \"doneTimeoutInMs\": 60000\n                 }\n            ]\n        },\n        {\n            \"name\": \"ExternalInterrupt2\",\n            \"properties\": [\n                {\n                   \"name\": \"NI.ChannelName\",\n                   \"dataType\": \"String\",\n                   \"value\": \"ExternalInterrupt2\"\n                },\n                {\n                    \"name\": \"NI.ExternalInterrupt.Done\",\n                    \"dataType\": \"Bool\",\n                    \"access\": \"ReadOnly\",\n                    \"bitfield\": \"InterruptStatus/ExternalIntStatus2\"\n                },\n                {\n                    \"name\": \"NI.ExternalInterrupt.Armed\",\n                    \"dataType\": \"Bool\",\n                    \"access\": \"ReadOnly\",\n                    \"bitfield\": \"InterruptMask/ExternalIntMask2\"\n                },\n                {\n                    \"name\": \"NI.ExternalInterrupt.Enable\",\n                    \"dataType\": \"Bool\",\n                    \"access\": \"WriteOnly\",\n                    \"bitfield\": \"InterruptEnable/ExternalIntEnable2\"\n                },\n                {\n                    \"name\": \"NI.ExternalInterrupt.Disable\",\n                    \"dataType\": \"Bool\",\n                    \"access\": \"WriteOnly\",\n                    \"bitfield\": \"InterruptDisable/ExternalIntDisable2\"\n                },\n                {\n                    \"name\": \"NI.ExternalInterrupt.Ack\",\n                    \"dataType\": \"Bool\",\n                    \"access\": \"WriteOnly\",\n                    \"bitfield\": \"InterruptAck/ExternalIntAck2\"\n                }\n            ],\n            \"commands\" : [\n                 {\n                     \"name\": \"NI.ExternalInterrupt.Wait\",\n                     \"description-en\": \"Wait for the external interrupt\",\n                     \"documentation-en\": \"Wait for the external interrupt\",\n                     \"startBitfield\": \"InterruptAck/ExternalIntAck2\", \n                     \"doneInterrupt\": \"ExternalInt2\",\n                     \"doneTimeoutInMs\": 60000\n                 },\n                 {\n                     \"name\": \"NI.ExternalInterrupt.Poll\",\n                     \"description-en\": \"Poll for the external interrupt line to be asserted\",\n                     \"documentation-en\": \"Poll for the external interrupt line to be asserted\",\n                     \"startBitfield\": \"InterruptAck/ExternalIntAck2\", \n                     \"doneBitfield\": \"InterruptStatus/ExternalIntStatus2\",\n                     \"doneTimeoutInMs\": 60000\n                 }\n            ]\n        },\n        {\n            \"name\": \"ExternalInterrupt3\",\n            \"properties\": [\n                {\n                   \"name\": \"NI.ChannelName\",\n                   \"dataType\": \"String\",\n                   \"value\": \"ExternalInterrupt3\"\n                },\n                {\n                    \"name\": \"NI.ExternalInterrupt.Done\",\n                    \"dataType\": \"Bool\",\n                    \"access\": \"ReadOnly\",\n                    \"bitfield\": \"InterruptStatus/ExternalIntStatus3\"\n                },\n                {\n                    \"name\": \"NI.ExternalInterrupt.Armed\",\n                    \"dataType\": \"Bool\",\n                    \"access\": \"ReadOnly\",\n                    \"bitfield\": \"InterruptMask/ExternalIntMask3\"\n                },\n                {\n                    \"name\": \"NI.ExternalInterrupt.Enable\",\n                    \"dataType\": \"Bool\",\n                    \"access\": \"WriteOnly\",\n                    \"bitfield\": \"InterruptEnable/ExternalIntEnable3\"\n                },\n                {\n                    \"name\": \"NI.ExternalInterrupt.Disable\",\n                    \"dataType\": \"Bool\",\n                    \"access\": \"WriteOnly\",\n                    \"bitfield\": \"InterruptDisable/ExternalIntDisable3\"\n                },\n                {\n                    \"name\": \"NI.ExternalInterrupt.Ack\",\n                    \"dataType\": \"Bool\",\n                    \"access\": \"WriteOnly\",\n                    \"bitfield\": \"InterruptAck/ExternalIntAck3\"\n                }\n            ],\n            \"commands\" : [\n                 {\n                     \"name\": \"NI.ExternalInterrupt.Wait\",\n                     \"description-en\": \"Wait for the external interrupt\",\n                     \"documentation-en\": \"Wait for the external interrupt\",\n                     \"startBitfield\": \"InterruptAck/ExternalIntAck3\", \n                     \"doneInterrupt\": \"ExternalInt3\",\n                     \"doneTimeoutInMs\": 60000\n                 },\n                 {\n                     \"name\": \"NI.ExternalInterrupt.Poll\",\n                     \"description-en\": \"Poll for the external interrupt line to be asserted\",\n                     \"documentation-en\": \"Poll for the external interrupt line to be asserted\",\n                     \"startBitfield\": \"InterruptAck/ExternalIntAck3\", \n                     \"doneBitfield\": \"InterruptStatus/ExternalIntStatus3\",\n                     \"doneTimeoutInMs\": 60000\n                 }\n            ]\n        },\n        {\n            \"name\": \"Scratchpad/Size_64\",\n            \"description-en\": \"Channel for testing a single slash in channel names\",\n            \"properties\": [\n                {\n                   \"name\": \"NI.ChannelName\",\n                   \"dataType\": \"String\",\n                   \"value\": \"Scratchpad/64\"\n                },\n                {\n                    \"name\": \"NI.Scratchpad.AsUInt64\",\n                    \"description-en\": \"use 64-bit Scratchpad as UInt64\",\n                    \"documentation-en\": \"Read write 64-bit scratchpad with UInt64 type\",\n                    \"dataType\": \"UInt64\",\n                    \"access\": \"ReadWrite\",\n                    \"bitfield\": \"DebugScratch64/Scratch64\"\n                }\n            ]\n        },\n        {\n            \"name\": \"Scratchpad/Copy2/Size_64\",\n            \"description-en\": \"Channel for testing multiple slashes in channel names\",\n            \"properties\": [\n                {\n                   \"name\": \"NI.ChannelName\",\n                   \"dataType\": \"String\",\n                   \"value\": \"Scratchpad/Copy2/64\"\n                },\n                {\n                    \"name\": \"NI.Scratchpad.AsUInt64\",\n                    \"description-en\": \"use 64-bit Scratchpad as UInt64\",\n                    \"documentation-en\": \"Read write 64-bit scratchpad with UInt64 type\",\n                    \"dataType\": \"UInt64\",\n                    \"access\": \"ReadWrite\",\n                    \"bitfield\": \"DebugScratch64/Scratch64\"\n                }\n            ]\n        },\n        {\n            \"name\": \"Scratchpad64\",\n            \"properties\": [\n                {\n                   \"name\": \"NI.ChannelName\",\n                   \"dataType\": \"String\",\n                   \"value\": \"Scratchpad64\"\n                },\n                {\n                    \"name\": \"NI.Scratchpad.RegisterSize\",\n                    \"description-en\": \"Indicates the width of the register backing this physical channel\",\n                    \"dataType\": \"Int32\",\n                    \"value\": 64\n                },\n                {\n                    \"name\": \"NI.Scratchpad.AsBool\",\n                    \"description-en\": \"use 64-bit Scratchpad as Bool\",\n                    \"documentation-en\": \"Read write 64-bit scratchpad with Bool value\",\n                    \"dataType\": \"Bool\",\n                    \"access\": \"ReadWrite\",\n                    \"bitfield\": \"DebugScratch64/ScratchBool\"\n                },\n                {\n                    \"name\": \"NI.Scratchpad.AsBool.U64\",\n                    \"description-en\": \"registerSize=64, bitfieldSize=64, dataType=Bool\",\n                    \"documentation-en\": \"Read write 64-bit scratchpad with U64 range as Bool\",\n                    \"dataType\": \"Bool\",\n                    \"access\": \"ReadWrite\",\n                    \"bitfield\": \"DebugScratch64/Scratch64\"\n                },\n                {\n                    \"name\": \"NI.Scratchpad.AsBool.I64\",\n                    \"description-en\": \"registerSize=64, bitfieldSize=64, dataType=Bool\",\n                    \"documentation-en\": \"Read write 64-bit scratchpad with I64 range as Bool\",\n                    \"dataType\": \"Bool\",\n                    \"access\": \"ReadWrite\",\n                    \"bitfield\": \"DebugScratch64/ScratchI64\"\n                },\n                {\n                    \"name\": \"NI.Scratchpad.AsBool.U32\",\n                    \"description-en\": \"registerSize=64, bitfieldSize=32, dataType=Bool\",\n                    \"documentation-en\": \"Read write 64-bit scratchpad with U32 range as Bool\",\n                    \"dataType\": \"Bool\",\n                    \"access\": \"ReadWrite\",\n                    \"bitfield\": \"DebugScratch64/Scratch32\"\n                },\n                {\n                    \"name\": \"NI.Scratchpad.AsBool.I32\",\n                    \"description-en\": \"registerSize=64, bitfieldSize=32, dataType=Bool\",\n                    \"documentation-en\": \"Read write 64-bit scratchpad with I32 range as Bool\",\n                    \"dataType\": \"Bool\",\n                    \"access\": \"ReadWrite\",\n                    \"bitfield\": \"DebugScratch64/ScratchI32\"\n                },\n                {\n                    \"name\": \"NI.Scratchpad.AsBool.U16\",\n                    \"description-en\": \"registerSize=64, bitfieldSize=16, dataType=Bool\",\n                    \"documentation-en\": \"Read write 64-bit scratchpad with U16 range as Bool\",\n                    \"dataType\": \"Bool\",\n                    \"access\": \"ReadWrite\",\n                    \"bitfield\": \"DebugScratch64/Scratch16\"\n                },\n                {\n                    \"name\": \"NI.Scratchpad.AsBool.I16\",\n                    \"description-en\": \"registerSize=64, bitfieldSize=16, dataType=Bool\",\n                    \"documentation-en\": \"Read write 64-bit scratchpad with I16 range as Bool\",\n                    \"dataType\": \"Bool\",\n                    \"access\": \"ReadWrite\",\n                    \"bitfield\": \"DebugScratch64/ScratchI16\"\n                },\n                {\n                    \"name\": \"NI.Scratchpad.AsBool.U8\",\n                    \"description-en\": \"registerSize=64, bitfieldSize=8, dataType=Bool\",\n                    \"documentation-en\": \"Read write 64-bit scratchpad with U8 range as Bool\",\n                    \"dataType\": \"Bool\",\n                    \"access\": \"ReadWrite\",\n                    \"bitfield\": \"DebugScratch64/Scratch8\"\n                },\n                {\n                    \"name\": \"NI.Scratchpad.AsBool.I8\",\n                    \"description-en\": \"registerSize=64, bitfieldSize=8, dataType=Bool\",\n                    \"documentation-en\": \"Read write 64-bit scratchpad with I8 range as Bool\",\n                    \"dataType\": \"Bool\",\n                    \"access\": \"ReadWrite\",\n                    \"bitfield\": \"DebugScratch64/ScratchI8\"\n                },\n        \n                {\n                    \"name\": \"NI.Scratchpad.AsBool.InvertBoolean\",\n                    \"dataType\": \"Bool\",\n                    \"access\": \"ReadWrite\",\n                    \"bitfield\": \"DebugScratch64/ScratchBool\",\n                    \"scale\": \"InvertBoolean\"\n                },\n                {\n                    \"name\": \"NI.Scratchpad.AsBool.TableStrictTrueFalse\",\n                    \"dataType\": \"Bool\",\n                    \"access\": \"ReadWrite\",\n                    \"bitfield\": \"DebugScratch64/ScratchI64\",\n                    \"scale\": \"TableStrictTrueFalse\"\n                },\n                {\n                    \"name\": \"NI.Scratchpad.AsBool.TableStrictFalse\",\n                    \"dataType\": \"Bool\",\n                    \"access\": \"ReadWrite\",\n                    \"bitfield\": \"DebugScratch64/ScratchI64\",\n                    \"scale\": \"TableStrictFalse\"\n                },\n                {\n                    \"name\": \"NI.Scratchpad.AsBool.TableStrictTrue\",\n                    \"dataType\": \"Bool\",\n                    \"access\": \"ReadWrite\",\n                    \"bitfield\": \"DebugScratch64/ScratchI64\",\n                    \"scale\": \"TableStrictTrue\"\n                },\n                {\n                    \"name\": \"NI.Scratchpad.AsBool.Bool\",\n                    \"description-en\": \"registerSize=64, bitfieldSize=1, dataType=Bool\",\n                    \"documentation-en\": \"Read write 64-bit scratchpad with 1 bit range as Bool\",\n                    \"dataType\": \"Bool\",\n                    \"access\": \"ReadWrite\",\n                    \"bitfield\": \"DebugScratch64/ScratchBool\"\n                },\n                {\n                    \"name\": \"NI.Scratchpad.AsDouble\",\n                    \"description-en\": \"use 64-bit Scratchpad as Double\",\n                    \"documentation-en\": \"Read write 64-bit scratchpad with Double value\",\n                    \"dataType\": \"Double\",\n                    \"access\": \"ReadWrite\",\n                    \"bitfield\": \"DebugScratch64/ScratchI64\"\n                },\n                {\n                    \"name\": \"NI.Scratchpad.AsDouble.U64\",\n                    \"description-en\": \"registerSize=64, bitfieldSize=64, dataType=Double\",\n                    \"documentation-en\": \"Read write 64-bit scratchpad with U64 range as Double\",\n                    \"dataType\": \"Double\",\n                    \"access\": \"ReadWrite\",\n                    \"bitfield\": \"DebugScratch64/Scratch64\"\n                },\n                {\n                    \"name\": \"NI.Scratchpad.AsDouble.I64\",\n                    \"description-en\": \"registerSize=64, bitfieldSize=64, dataType=Double\",\n                    \"documentation-en\": \"Read write 64-bit scratchpad with I64 range as Double\",\n                    \"dataType\": \"Double\",\n                    \"access\": \"ReadWrite\",\n                    \"bitfield\": \"DebugScratch64/ScratchI64\"\n                },\n                {\n                    \"name\": \"NI.Scratchpad.AsDouble.U32\",\n                    \"description-en\": \"registerSize=64, bitfieldSize=32, dataType=Double\",\n                    \"documentation-en\": \"Read write 64-bit scratchpad with U32 range as Double\",\n                    \"dataType\": \"Double\",\n                    \"access\": \"ReadWrite\",\n                    \"bitfield\": \"DebugScratch64/Scratch32\"\n                },\n                {\n                    \"name\": \"NI.Scratchpad.AsDouble.I32\",\n                    \"description-en\": \"registerSize=64, bitfieldSize=32, dataType=Double\",\n                    \"documentation-en\": \"Read write 64-bit scratchpad with I32 range as Double\",\n                    \"dataType\": \"Double\",\n                    \"access\": \"ReadWrite\",\n                    \"bitfield\": \"DebugScratch64/ScratchI32\"\n                },\n                {\n                    \"name\": \"NI.Scratchpad.AsDouble.U16\",\n                    \"description-en\": \"registerSize=64, bitfieldSize=16, dataType=Double\",\n                    \"documentation-en\": \"Read write 64-bit scratchpad with U16 range as Double\",\n                    \"dataType\": \"Double\",\n                    \"access\": \"ReadWrite\",\n                    \"bitfield\": \"DebugScratch64/Scratch16\"\n                },\n                {\n                    \"name\": \"NI.Scratchpad.AsDouble.I16\",\n                    \"description-en\": \"registerSize=64, bitfieldSize=16, dataType=Double\",\n                    \"documentation-en\": \"Read write 64-bit scratchpad with I16 range as Double\",\n                    \"dataType\": \"Double\",\n                    \"access\": \"ReadWrite\",\n                    \"bitfield\": \"DebugScratch64/ScratchI16\"\n                },\n                {\n                    \"name\": \"NI.Scratchpad.AsDouble.U8\",\n                    \"description-en\": \"registerSize=64, bitfieldSize=8, dataType=Double\",\n                    \"documentation-en\": \"Read write 64-bit scratchpad with U8 range as Double\",\n                    \"dataType\": \"Double\",\n                    \"access\": \"ReadWrite\",\n                    \"bitfield\": \"DebugScratch64/Scratch8\"\n                },\n                {\n                    \"name\": \"NI.Scratchpad.AsDouble.I8\",\n                    \"description-en\": \"registerSize=64, bitfieldSize=8, dataType=Double\",\n                    \"documentation-en\": \"Read write 64-bit scratchpad with I8 range as Double\",\n                    \"dataType\": \"Double\",\n                    \"access\": \"ReadWrite\",\n                    \"bitfield\": \"DebugScratch64/ScratchI8\"\n                },\n        \n                {\n                    \"name\": \"NI.Scratchpad.AsDouble.TableStrict\",\n                    \"dataType\": \"Double\",\n                    \"access\": \"ReadWrite\",\n                    \"bitfield\": \"DebugScratch64/ScratchI64\",\n                    \"scale\": \"TableStrict\"\n                },\n                {\n                    \"name\": \"NI.Scratchpad.AsDouble.TableStrict12Elements\",\n                    \"dataType\": \"Double\",\n                    \"access\": \"ReadWrite\",\n                    \"bitfield\": \"DebugScratch64/ScratchI64\",\n                    \"scale\": \"TableStrict12Elements\"\n                },\n                {\n                    \"name\": \"NI.Scratchpad.AsDouble.TableRound\",\n                    \"dataType\": \"Double\",\n                    \"access\": \"ReadWrite\",\n                    \"bitfield\": \"DebugScratch64/ScratchI64\",\n                    \"scale\": \"TableRound\"\n                },\n                {\n                    \"name\": \"NI.Scratchpad.AsDouble.TableInterpolate\",\n                    \"dataType\": \"Double\",\n                    \"access\": \"ReadWrite\",\n                    \"bitfield\": \"DebugScratch64/ScratchI64\",\n                    \"scale\": \"TableInterpolate\"\n                },\n                {\n                    \"name\": \"NI.Scratchpad.AsDouble.LinearDivideBy8\",\n                    \"dataType\": \"Double\",\n                    \"access\": \"ReadWrite\",\n                    \"bitfield\": \"DebugScratch64/ScratchI64\",\n                    \"scale\": \"LinearDivideBy8\"\n                },\n                {\n                    \"name\": \"NI.Scratchpad.AsDouble.Times2Plus2\",\n                    \"dataType\": \"Double\",\n                    \"access\": \"ReadWrite\",\n                    \"bitfield\": \"DebugScratch64/ScratchI64\",\n                    \"scale\": \"Times2Plus2\"\n                },\n                {\n                    \"name\": \"NI.Scratchpad.AsDouble.PolynomialThermocouple\",\n                    \"dataType\": \"Double\",\n                    \"access\": \"ReadWrite\",\n                    \"bitfield\": \"DebugScratch64/ScratchI64\",\n                    \"scale\": \"PolynomialThermocouple\",\n                    \"min\": 0,\n                    \"max\": 760\n                },\n                {\n                    \"name\": \"NI.Scratchpad.AsDouble.PolynomialBoundaryConditions\",\n                    \"dataType\": \"Double\",\n                    \"access\": \"ReadWrite\",\n                    \"bitfield\": \"DebugScratch64/ScratchI64\",\n                    \"scale\": \"PolynomialBoundaryConditions\"\n                },\n                {\n                    \"name\": \"NI.Scratchpad.AsDouble.Bool\",\n                    \"description-en\": \"registerSize=64, bitfieldSize=1, dataType=Double\",\n                    \"documentation-en\": \"Read write 64-bit scratchpad with 1 bit range as Double\",\n                    \"dataType\": \"Double\",\n                    \"access\": \"ReadWrite\",\n                    \"bitfield\": \"DebugScratch64/ScratchBool\"\n                },\n                {\n                    \"name\": \"NI.Scratchpad.AsInt32\",\n                    \"description-en\": \"use 64-bit Scratchpad as Int32\",\n                    \"documentation-en\": \"Read write 64-bit scratchpad with Int32 value\",\n                    \"dataType\": \"Int32\",\n                    \"access\": \"ReadWrite\",\n                    \"bitfield\": \"DebugScratch64/ScratchI32\"\n                },\n                {\n                    \"name\": \"NI.Scratchpad.AsInt32.U64\",\n                    \"description-en\": \"registerSize=64, bitfieldSize=64, dataType=Int32\",\n                    \"documentation-en\": \"Read write 64-bit scratchpad with U64 range as Int32\",\n                    \"dataType\": \"Int32\",\n                    \"access\": \"ReadWrite\",\n                    \"bitfield\": \"DebugScratch64/Scratch64\"\n                },\n                {\n                    \"name\": \"NI.Scratchpad.AsInt32.I64\",\n                    \"description-en\": \"registerSize=64, bitfieldSize=64, dataType=Int32\",\n                    \"documentation-en\": \"Read write 64-bit scratchpad with I64 range as Int32\",\n                    \"dataType\": \"Int32\",\n                    \"access\": \"ReadWrite\",\n                    \"bitfield\": \"DebugScratch64/ScratchI64\"\n                },\n                {\n                    \"name\": \"NI.Scratchpad.AsInt32.U32\",\n                    \"description-en\": \"registerSize=64, bitfieldSize=32, dataType=Int32\",\n                    \"documentation-en\": \"Read write 64-bit scratchpad with U32 range as Int32\",\n                    \"dataType\": \"Int32\",\n                    \"access\": \"ReadWrite\",\n                    \"bitfield\": \"DebugScratch64/Scratch32\"\n                },\n                {\n                    \"name\": \"NI.Scratchpad.AsInt32.I32\",\n                    \"description-en\": \"registerSize=64, bitfieldSize=32, dataType=Int32\",\n                    \"documentation-en\": \"Read write 64-bit scratchpad with I32 range as Int32\",\n                    \"dataType\": \"Int32\",\n                    \"access\": \"ReadWrite\",\n                    \"bitfield\": \"DebugScratch64/ScratchI32\"\n                },\n                {\n                    \"name\": \"NI.Scratchpad.AsInt32.U16\",\n                    \"description-en\": \"registerSize=64, bitfieldSize=16, dataType=Int32\",\n                    \"documentation-en\": \"Read write 64-bit scratchpad with U16 range as Int32\",\n                    \"dataType\": \"Int32\",\n                    \"access\": \"ReadWrite\",\n                    \"bitfield\": \"DebugScratch64/Scratch16\"\n                },\n                {\n                    \"name\": \"NI.Scratchpad.AsInt32.I16\",\n                    \"description-en\": \"registerSize=64, bitfieldSize=16, dataType=Int32\",\n                    \"documentation-en\": \"Read write 64-bit scratchpad with I16 range as Int32\",\n                    \"dataType\": \"Int32\",\n                    \"access\": \"ReadWrite\",\n                    \"bitfield\": \"DebugScratch64/ScratchI16\"\n                },\n                {\n                    \"name\": \"NI.Scratchpad.AsInt32.U8\",\n                    \"description-en\": \"registerSize=64, bitfieldSize=8, dataType=Int32\",\n                    \"documentation-en\": \"Read write 64-bit scratchpad with U8 range as Int32\",\n                    \"dataType\": \"Int32\",\n                    \"access\": \"ReadWrite\",\n                    \"bitfield\": \"DebugScratch64/Scratch8\"\n                },\n                {\n                    \"name\": \"NI.Scratchpad.AsInt32.I8\",\n                    \"description-en\": \"registerSize=64, bitfieldSize=8, dataType=Int32\",\n                    \"documentation-en\": \"Read write 64-bit scratchpad with I8 range as Int32\",\n                    \"dataType\": \"Int32\",\n                    \"access\": \"ReadWrite\",\n                    \"bitfield\": \"DebugScratch64/ScratchI8\"\n                },\n        \n                {\n                    \"name\": \"NI.Scratchpad.AsInt32.TableStrict12Elements\",\n                    \"dataType\": \"Int32\",\n                    \"access\": \"ReadWrite\",\n                    \"bitfield\": \"DebugScratch64/ScratchI32\",\n                    \"scale\": \"TableStrict12Elements\"\n                },\n                {\n                    \"name\": \"NI.Scratchpad.AsInt32.TableRound\",\n                    \"dataType\": \"Int32\",\n                    \"access\": \"ReadWrite\",\n                    \"bitfield\": \"DebugScratch64/ScratchI32\",\n                    \"scale\": \"TableRound\"\n                },\n                {\n                    \"name\": \"NI.Scratchpad.AsInt32.TableInterpolate\",\n                    \"dataType\": \"Int32\",\n                    \"access\": \"ReadWrite\",\n                    \"bitfield\": \"DebugScratch64/ScratchI32\",\n                    \"scale\": \"TableInterpolate\"\n                },\n                {\n                    \"name\": \"NI.Scratchpad.AsInt32.LinearDivideBy8\",\n                    \"dataType\": \"Int32\",\n                    \"access\": \"ReadWrite\",\n                    \"bitfield\": \"DebugScratch64/ScratchI32\",\n                    \"scale\": \"LinearDivideBy8\"\n                },\n                {\n                    \"name\": \"NI.Scratchpad.AsInt32.Times2Plus2\",\n                    \"dataType\": \"Int32\",\n                    \"access\": \"ReadWrite\",\n                    \"bitfield\": \"DebugScratch64/ScratchI32\",\n                    \"scale\": \"Times2Plus2\"\n                },\n                {\n                    \"name\": \"NI.Scratchpad.AsInt32.PolynomialThermocouple\",\n                    \"dataType\": \"Int32\",\n                    \"access\": \"ReadWrite\",\n                    \"bitfield\": \"DebugScratch64/ScratchI32\",\n                    \"scale\": \"PolynomialThermocouple\",\n                    \"min\": 0,\n                    \"max\": 760\n                },\n                {\n                    \"name\": \"NI.Scratchpad.AsInt32.PolynomialBoundaryConditions\",\n                    \"dataType\": \"Int32\",\n                    \"access\": \"ReadWrite\",\n                    \"bitfield\": \"DebugScratch64/ScratchI32\",\n                    \"scale\": \"PolynomialBoundaryConditions\"\n                },\n                {\n                    \"name\": \"NI.Scratchpad.AsInt32.Bool\",\n                    \"description-en\": \"registerSize=64, bitfieldSize=1, dataType=Int32\",\n                    \"documentation-en\": \"Read write 64-bit scratchpad with 1 bit range as Int32\",\n                    \"dataType\": \"Int32\",\n                    \"access\": \"ReadWrite\",\n                    \"bitfield\": \"DebugScratch64/ScratchBool\"\n                },\n                {\n                    \"name\": \"NI.Scratchpad.AsInt64\",\n                    \"description-en\": \"use 64-bit Scratchpad as Int64\",\n                    \"documentation-en\": \"Read write 64-bit scratchpad with Int64 value\",\n                    \"dataType\": \"Int64\",\n                    \"access\": \"ReadWrite\",\n                    \"bitfield\": \"DebugScratch64/ScratchI64\"\n                },\n                {\n                    \"name\": \"NI.Scratchpad.AsInt64.U64\",\n                    \"description-en\": \"registerSize=64, bitfieldSize=64, dataType=Int64\",\n                    \"documentation-en\": \"Read write 64-bit scratchpad with U64 range as Int64\",\n                    \"dataType\": \"Int64\",\n                    \"access\": \"ReadWrite\",\n                    \"bitfield\": \"DebugScratch64/Scratch64\"\n                },\n                {\n                    \"name\": \"NI.Scratchpad.AsInt64.I64\",\n                    \"description-en\": \"registerSize=64, bitfieldSize=64, dataType=Int64\",\n                    \"documentation-en\": \"Read write 64-bit scratchpad with I64 range as Int64\",\n                    \"dataType\": \"Int64\",\n                    \"access\": \"ReadWrite\",\n                    \"bitfield\": \"DebugScratch64/ScratchI64\"\n                },\n                {\n                    \"name\": \"NI.Scratchpad.AsInt64.U32\",\n                    \"description-en\": \"registerSize=64, bitfieldSize=32, dataType=Int64\",\n                    \"documentation-en\": \"Read write 64-bit scratchpad with U32 range as Int64\",\n                    \"dataType\": \"Int64\",\n                    \"access\": \"ReadWrite\",\n                    \"bitfield\": \"DebugScratch64/Scratch32\"\n                },\n                {\n                    \"name\": \"NI.Scratchpad.AsInt64.I32\",\n                    \"description-en\": \"registerSize=64, bitfieldSize=32, dataType=Int64\",\n                    \"documentation-en\": \"Read write 64-bit scratchpad with I32 range as Int64\",\n                    \"dataType\": \"Int64\",\n                    \"access\": \"ReadWrite\",\n                    \"bitfield\": \"DebugScratch64/ScratchI32\"\n                },\n                {\n                    \"name\": \"NI.Scratchpad.AsInt64.U16\",\n                    \"description-en\": \"registerSize=64, bitfieldSize=16, dataType=Int64\",\n                    \"documentation-en\": \"Read write 64-bit scratchpad with U16 range as Int64\",\n                    \"dataType\": \"Int64\",\n                    \"access\": \"ReadWrite\",\n                    \"bitfield\": \"DebugScratch64/Scratch16\"\n                },\n                {\n                    \"name\": \"NI.Scratchpad.AsInt64.I16\",\n                    \"description-en\": \"registerSize=64, bitfieldSize=16, dataType=Int64\",\n                    \"documentation-en\": \"Read write 64-bit scratchpad with I16 range as Int64\",\n                    \"dataType\": \"Int64\",\n                    \"access\": \"ReadWrite\",\n                    \"bitfield\": \"DebugScratch64/ScratchI16\"\n                },\n                {\n                    \"name\": \"NI.Scratchpad.AsInt64.U8\",\n                    \"description-en\": \"registerSize=64, bitfieldSize=8, dataType=Int64\",\n                    \"documentation-en\": \"Read write 64-bit scratchpad with U8 range as Int64\",\n                    \"dataType\": \"Int64\",\n                    \"access\": \"ReadWrite\",\n                    \"bitfield\": \"DebugScratch64/Scratch8\"\n                },\n                {\n                    \"name\": \"NI.Scratchpad.AsInt64.I8\",\n                    \"description-en\": \"registerSize=64, bitfieldSize=8, dataType=Int64\",\n                    \"documentation-en\": \"Read write 64-bit scratchpad with I8 range as Int64\",\n                    \"dataType\": \"Int64\",\n                    \"access\": \"ReadWrite\",\n                    \"bitfield\": \"DebugScratch64/ScratchI8\"\n                },\n        \n                {\n                    \"name\": \"NI.Scratchpad.AsInt64.TableStrict12Elements\",\n                    \"dataType\": \"Int64\",\n                    \"access\": \"ReadWrite\",\n                    \"bitfield\": \"DebugScratch64/ScratchI64\",\n                    \"scale\": \"TableStrict12Elements\"\n                },\n                {\n                    \"name\": \"NI.Scratchpad.AsInt64.TableRound\",\n                    \"dataType\": \"Int64\",\n                    \"access\": \"ReadWrite\",\n                    \"bitfield\": \"DebugScratch64/ScratchI64\",\n                    \"scale\": \"TableRound\"\n                },\n                {\n                    \"name\": \"NI.Scratchpad.AsInt64.TableInterpolate\",\n                    \"dataType\": \"Int64\",\n                    \"access\": \"ReadWrite\",\n                    \"bitfield\": \"DebugScratch64/ScratchI64\",\n                    \"scale\": \"TableInterpolate\"\n                },\n                {\n                    \"name\": \"NI.Scratchpad.AsInt64.LinearDivideBy8\",\n                    \"dataType\": \"Int64\",\n                    \"access\": \"ReadWrite\",\n                    \"bitfield\": \"DebugScratch64/ScratchI64\",\n                    \"scale\": \"LinearDivideBy8\"\n                },\n                {\n                    \"name\": \"NI.Scratchpad.AsInt64.Times2Plus2\",\n                    \"dataType\": \"Int64\",\n                    \"access\": \"ReadWrite\",\n                    \"bitfield\": \"DebugScratch64/ScratchI64\",\n                    \"scale\": \"Times2Plus2\"\n                },\n                {\n                    \"name\": \"NI.Scratchpad.AsInt64.PolynomialThermocouple\",\n                    \"dataType\": \"Int64\",\n                    \"access\": \"ReadWrite\",\n                    \"bitfield\": \"DebugScratch64/ScratchI64\",\n                    \"scale\": \"PolynomialThermocouple\",\n                    \"min\": 0,\n                    \"max\": 760\n                },\n                {\n                    \"name\": \"NI.Scratchpad.AsInt64.PolynomialBoundaryConditions\",\n                    \"dataType\": \"Int64\",\n                    \"access\": \"ReadWrite\",\n                    \"bitfield\": \"DebugScratch64/ScratchI64\",\n                    \"scale\": \"PolynomialBoundaryConditions\"\n                },\n                {\n                    \"name\": \"NI.Scratchpad.AsInt64.Bool\",\n                    \"description-en\": \"registerSize=64, bitfieldSize=1, dataType=Int64\",\n                    \"documentation-en\": \"Read write 64-bit scratchpad with 1 bit range as Int64\",\n                    \"dataType\": \"Int64\",\n                    \"access\": \"ReadWrite\",\n                    \"bitfield\": \"DebugScratch64/ScratchBool\"\n                },\n                {\n                    \"name\": \"NI.Scratchpad.AsUInt32\",\n                    \"description-en\": \"use 64-bit Scratchpad as UInt32\",\n                    \"documentation-en\": \"Read write 64-bit scratchpad with UInt32 value\",\n                    \"dataType\": \"UInt32\",\n                    \"access\": \"ReadWrite\",\n                    \"bitfield\": \"DebugScratch64/Scratch32\"\n                },\n                {\n                    \"name\": \"NI.Scratchpad.AsUInt32.U64\",\n                    \"description-en\": \"registerSize=64, bitfieldSize=64, dataType=UInt32\",\n                    \"documentation-en\": \"Read write 64-bit scratchpad with U64 range as UInt32\",\n                    \"dataType\": \"UInt32\",\n                    \"access\": \"ReadWrite\",\n                    \"bitfield\": \"DebugScratch64/Scratch64\"\n                },\n                {\n                    \"name\": \"NI.Scratchpad.AsUInt32.I64\",\n                    \"description-en\": \"registerSize=64, bitfieldSize=64, dataType=UInt32\",\n                    \"documentation-en\": \"Read write 64-bit scratchpad with I64 range as UInt32\",\n                    \"dataType\": \"UInt32\",\n                    \"access\": \"ReadWrite\",\n                    \"bitfield\": \"DebugScratch64/ScratchI64\"\n                },\n                {\n                    \"name\": \"NI.Scratchpad.AsUInt32.U32\",\n                    \"description-en\": \"registerSize=64, bitfieldSize=32, dataType=UInt32\",\n                    \"documentation-en\": \"Read write 64-bit scratchpad with U32 range as UInt32\",\n                    \"dataType\": \"UInt32\",\n                    \"access\": \"ReadWrite\",\n                    \"bitfield\": \"DebugScratch64/Scratch32\"\n                },\n                {\n                    \"name\": \"NI.Scratchpad.AsUInt32.I32\",\n                    \"description-en\": \"registerSize=64, bitfieldSize=32, dataType=UInt32\",\n                    \"documentation-en\": \"Read write 64-bit scratchpad with I32 range as UInt32\",\n                    \"dataType\": \"UInt32\",\n                    \"access\": \"ReadWrite\",\n                    \"bitfield\": \"DebugScratch64/ScratchI32\"\n                },\n                {\n                    \"name\": \"NI.Scratchpad.AsUInt32.U16\",\n                    \"description-en\": \"registerSize=64, bitfieldSize=16, dataType=UInt32\",\n                    \"documentation-en\": \"Read write 64-bit scratchpad with U16 range as UInt32\",\n                    \"dataType\": \"UInt32\",\n                    \"access\": \"ReadWrite\",\n                    \"bitfield\": \"DebugScratch64/Scratch16\"\n                },\n                {\n                    \"name\": \"NI.Scratchpad.AsUInt32.I16\",\n                    \"description-en\": \"registerSize=64, bitfieldSize=16, dataType=UInt32\",\n                    \"documentation-en\": \"Read write 64-bit scratchpad with I16 range as UInt32\",\n                    \"dataType\": \"UInt32\",\n                    \"access\": \"ReadWrite\",\n                    \"bitfield\": \"DebugScratch64/ScratchI16\"\n                },\n                {\n                    \"name\": \"NI.Scratchpad.AsUInt32.U8\",\n                    \"description-en\": \"registerSize=64, bitfieldSize=8, dataType=UInt32\",\n                    \"documentation-en\": \"Read write 64-bit scratchpad with U8 range as UInt32\",\n                    \"dataType\": \"UInt32\",\n                    \"access\": \"ReadWrite\",\n                    \"bitfield\": \"DebugScratch64/Scratch8\"\n                },\n                {\n                    \"name\": \"NI.Scratchpad.AsUInt32.I8\",\n                    \"description-en\": \"registerSize=64, bitfieldSize=8, dataType=UInt32\",\n                    \"documentation-en\": \"Read write 64-bit scratchpad with I8 range as UInt32\",\n                    \"dataType\": \"UInt32\",\n                    \"access\": \"ReadWrite\",\n                    \"bitfield\": \"DebugScratch64/ScratchI8\"\n                },\n        \n                {\n                    \"name\": \"NI.Scratchpad.AsUInt32.TableStrict12Elements\",\n                    \"dataType\": \"UInt32\",\n                    \"access\": \"ReadWrite\",\n                    \"bitfield\": \"DebugScratch64/Scratch32\",\n                    \"scale\": \"TableStrict12Elements\"\n                },\n                {\n                    \"name\": \"NI.Scratchpad.AsUInt32.TableRound\",\n                    \"dataType\": \"UInt32\",\n                    \"access\": \"ReadWrite\",\n                    \"bitfield\": \"DebugScratch64/Scratch32\",\n                    \"scale\": \"TableRound\"\n                },\n                {\n                    \"name\": \"NI.Scratchpad.AsUInt32.TableInterpolate\",\n                    \"dataType\": \"UInt32\",\n                    \"access\": \"ReadWrite\",\n                    \"bitfield\": \"DebugScratch64/Scratch32\",\n                    \"scale\": \"TableInterpolate\"\n                },\n                {\n                    \"name\": \"NI.Scratchpad.AsUInt32.LinearDivideBy8\",\n                    \"dataType\": \"UInt32\",\n                    \"access\": \"ReadWrite\",\n                    \"bitfield\": \"DebugScratch64/Scratch32\",\n                    \"scale\": \"LinearDivideBy8\"\n                },\n                {\n                    \"name\": \"NI.Scratchpad.AsUInt32.Times2Plus2\",\n                    \"dataType\": \"UInt32\",\n                    \"access\": \"ReadWrite\",\n                    \"bitfield\": \"DebugScratch64/Scratch32\",\n                    \"scale\": \"Times2Plus2\"\n                },\n                {\n                    \"name\": \"NI.Scratchpad.AsUInt32.PolynomialThermocouple\",\n                    \"dataType\": \"UInt32\",\n                    \"access\": \"ReadWrite\",\n                    \"bitfield\": \"DebugScratch64/Scratch32\",\n                    \"scale\": \"PolynomialThermocouple\",\n                    \"min\": 0,\n                    \"max\": 760\n                },\n                {\n                    \"name\": \"NI.Scratchpad.AsUInt32.PolynomialBoundaryConditions\",\n                    \"dataType\": \"UInt32\",\n                    \"access\": \"ReadWrite\",\n                    \"bitfield\": \"DebugScratch64/Scratch32\",\n                    \"scale\": \"PolynomialBoundaryConditions\"\n                },\n                {\n                    \"name\": \"NI.Scratchpad.AsUInt32.Bool\",\n                    \"description-en\": \"registerSize=64, bitfieldSize=1, dataType=UInt32\",\n                    \"documentation-en\": \"Read write 64-bit scratchpad with 1 bit range as UInt32\",\n                    \"dataType\": \"UInt32\",\n                    \"access\": \"ReadWrite\",\n                    \"bitfield\": \"DebugScratch64/ScratchBool\"\n                },\n                {\n                    \"name\": \"NI.Scratchpad.AsUInt64\",\n                    \"description-en\": \"use 64-bit Scratchpad as UInt64\",\n                    \"documentation-en\": \"Read write 64-bit scratchpad with UInt64 value\",\n                    \"dataType\": \"UInt64\",\n                    \"access\": \"ReadWrite\",\n                    \"bitfield\": \"DebugScratch64/Scratch64\"\n                },\n                {\n                    \"name\": \"NI.Scratchpad.AsUInt64.U64\",\n                    \"description-en\": \"registerSize=64, bitfieldSize=64, dataType=UInt64\",\n                    \"documentation-en\": \"Read write 64-bit scratchpad with U64 range as UInt64\",\n                    \"dataType\": \"UInt64\",\n                    \"access\": \"ReadWrite\",\n                    \"bitfield\": \"DebugScratch64/Scratch64\"\n                },\n                {\n                    \"name\": \"NI.Scratchpad.AsUInt64.I64\",\n                    \"description-en\": \"registerSize=64, bitfieldSize=64, dataType=UInt64\",\n                    \"documentation-en\": \"Read write 64-bit scratchpad with I64 range as UInt64\",\n                    \"dataType\": \"UInt64\",\n                    \"access\": \"ReadWrite\",\n                    \"bitfield\": \"DebugScratch64/ScratchI64\"\n                },\n                {\n                    \"name\": \"NI.Scratchpad.AsUInt64.U32\",\n                    \"description-en\": \"registerSize=64, bitfieldSize=32, dataType=UInt64\",\n                    \"documentation-en\": \"Read write 64-bit scratchpad with U32 range as UInt64\",\n                    \"dataType\": \"UInt64\",\n                    \"access\": \"ReadWrite\",\n                    \"bitfield\": \"DebugScratch64/Scratch32\"\n                },\n                {\n                    \"name\": \"NI.Scratchpad.AsUInt64.I32\",\n                    \"description-en\": \"registerSize=64, bitfieldSize=32, dataType=UInt64\",\n                    \"documentation-en\": \"Read write 64-bit scratchpad with I32 range as UInt64\",\n                    \"dataType\": \"UInt64\",\n                    \"access\": \"ReadWrite\",\n                    \"bitfield\": \"DebugScratch64/ScratchI32\"\n                },\n                {\n                    \"name\": \"NI.Scratchpad.AsUInt64.U16\",\n                    \"description-en\": \"registerSize=64, bitfieldSize=16, dataType=UInt64\",\n                    \"documentation-en\": \"Read write 64-bit scratchpad with U16 range as UInt64\",\n                    \"dataType\": \"UInt64\",\n                    \"access\": \"ReadWrite\",\n                    \"bitfield\": \"DebugScratch64/Scratch16\"\n                },\n                {\n                    \"name\": \"NI.Scratchpad.AsUInt64.I16\",\n                    \"description-en\": \"registerSize=64, bitfieldSize=16, dataType=UInt64\",\n                    \"documentation-en\": \"Read write 64-bit scratchpad with I16 range as UInt64\",\n                    \"dataType\": \"UInt64\",\n                    \"access\": \"ReadWrite\",\n                    \"bitfield\": \"DebugScratch64/ScratchI16\"\n                },\n                {\n                    \"name\": \"NI.Scratchpad.AsUInt64.U8\",\n                    \"description-en\": \"registerSize=64, bitfieldSize=8, dataType=UInt64\",\n                    \"documentation-en\": \"Read write 64-bit scratchpad with U8 range as UInt64\",\n                    \"dataType\": \"UInt64\",\n                    \"access\": \"ReadWrite\",\n                    \"bitfield\": \"DebugScratch64/Scratch8\"\n                },\n                {\n                    \"name\": \"NI.Scratchpad.AsUInt64.I8\",\n                    \"description-en\": \"registerSize=64, bitfieldSize=8, dataType=UInt64\",\n                    \"documentation-en\": \"Read write 64-bit scratchpad with I8 range as UInt64\",\n                    \"dataType\": \"UInt64\",\n                    \"access\": \"ReadWrite\",\n                    \"bitfield\": \"DebugScratch64/ScratchI8\"\n                },\n        \n                {\n                    \"name\": \"NI.Scratchpad.AsUInt64.TableStrict12Elements\",\n                    \"dataType\": \"UInt64\",\n                    \"access\": \"ReadWrite\",\n                    \"bitfield\": \"DebugScratch64/Scratch64\",\n                    \"scale\": \"TableStrict12Elements\"\n                },\n                {\n                    \"name\": \"NI.Scratchpad.AsUInt64.TableRound\",\n                    \"dataType\": \"UInt64\",\n                    \"access\": \"ReadWrite\",\n                    \"bitfield\": \"DebugScratch64/Scratch64\",\n                    \"scale\": \"TableRound\"\n                },\n                {\n                    \"name\": \"NI.Scratchpad.AsUInt64.TableInterpolate\",\n                    \"dataType\": \"UInt64\",\n                    \"access\": \"ReadWrite\",\n                    \"bitfield\": \"DebugScratch64/Scratch64\",\n                    \"scale\": \"TableInterpolate\"\n                },\n                {\n                    \"name\": \"NI.Scratchpad.AsUInt64.LinearDivideBy8\",\n                    \"dataType\": \"UInt64\",\n                    \"access\": \"ReadWrite\",\n                    \"bitfield\": \"DebugScratch64/Scratch64\",\n                    \"scale\": \"LinearDivideBy8\"\n                },\n                {\n                    \"name\": \"NI.Scratchpad.AsUInt64.Times2Plus2\",\n                    \"dataType\": \"UInt64\",\n                    \"access\": \"ReadWrite\",\n                    \"bitfield\": \"DebugScratch64/Scratch64\",\n                    \"scale\": \"Times2Plus2\"\n                },\n                {\n                    \"name\": \"NI.Scratchpad.AsUInt64.PolynomialThermocouple\",\n                    \"dataType\": \"UInt64\",\n                    \"access\": \"ReadWrite\",\n                    \"bitfield\": \"DebugScratch64/Scratch64\",\n                    \"scale\": \"PolynomialThermocouple\",\n                    \"min\": 0,\n                    \"max\": 760\n                },\n                {\n                    \"name\": \"NI.Scratchpad.AsUInt64.PolynomialBoundaryConditions\",\n                    \"dataType\": \"UInt64\",\n                    \"access\": \"ReadWrite\",\n                    \"bitfield\": \"DebugScratch64/Scratch64\",\n                    \"scale\": \"PolynomialBoundaryConditions\"\n                },\n                {\n                    \"name\": \"NI.Scratchpad.AsUInt64.Bool\",\n                    \"description-en\": \"registerSize=64, bitfieldSize=1, dataType=UInt64\",\n                    \"documentation-en\": \"Read write 64-bit scratchpad with 1 bit range as UInt64\",\n                    \"dataType\": \"UInt64\",\n                    \"access\": \"ReadWrite\",\n                    \"bitfield\": \"DebugScratch64/ScratchBool\"\n                }\n            ]\n        },\n        {\n            \"name\": \"Scratchpad32\",\n            \"properties\": [\n                {\n                   \"name\": \"NI.ChannelName\",\n                   \"dataType\": \"String\",\n                   \"value\": \"Scratchpad32\"\n                },\n                {\n                    \"name\": \"NI.Scratchpad.RegisterSize\",\n                    \"description-en\": \"Indicates the width of the register backing this physical channel\",\n                    \"dataType\": \"Int32\",\n                    \"value\": 32\n                },\n                {\n                    \"name\": \"NI.Scratchpad.AsBool\",\n                    \"description-en\": \"use 32-bit Scratchpad as Bool\",\n                    \"documentation-en\": \"Read write 32-bit scratchpad with Bool value\",\n                    \"dataType\": \"Bool\",\n                    \"access\": \"ReadWrite\",\n                    \"bitfield\": \"DebugScratch32/ScratchBool\"\n                },\n                {\n                    \"name\": \"NI.Scratchpad.AsBool.U32\",\n                    \"description-en\": \"registerSize=32, bitfieldSize=32, dataType=Bool\",\n                    \"documentation-en\": \"Read write 32-bit scratchpad with U32 range as Bool\",\n                    \"dataType\": \"Bool\",\n                    \"access\": \"ReadWrite\",\n                    \"bitfield\": \"DebugScratch32/Scratch32\"\n                },\n                {\n                    \"name\": \"NI.Scratchpad.AsBool.I32\",\n                    \"description-en\": \"registerSize=32, bitfieldSize=32, dataType=Bool\",\n                    \"documentation-en\": \"Read write 32-bit scratchpad with I32 range as Bool\",\n                    \"dataType\": \"Bool\",\n                    \"access\": \"ReadWrite\",\n                    \"bitfield\": \"DebugScratch32/ScratchI32\"\n                },\n                {\n                    \"name\": \"NI.Scratchpad.AsBool.U16\",\n                    \"description-en\": \"registerSize=32, bitfieldSize=16, dataType=Bool\",\n                    \"documentation-en\": \"Read write 32-bit scratchpad with U16 range as Bool\",\n                    \"dataType\": \"Bool\",\n                    \"access\": \"ReadWrite\",\n                    \"bitfield\": \"DebugScratch32/Scratch16\"\n                },\n                {\n                    \"name\": \"NI.Scratchpad.AsBool.I16\",\n                    \"description-en\": \"registerSize=32, bitfieldSize=16, dataType=Bool\",\n                    \"documentation-en\": \"Read write 32-bit scratchpad with I16 range as Bool\",\n                    \"dataType\": \"Bool\",\n                    \"access\": \"ReadWrite\",\n                    \"bitfield\": \"DebugScratch32/ScratchI16\"\n                },\n                {\n                    \"name\": \"NI.Scratchpad.AsBool.U8\",\n                    \"description-en\": \"registerSize=32, bitfieldSize=8, dataType=Bool\",\n                    \"documentation-en\": \"Read write 32-bit scratchpad with U8 range as Bool\",\n                    \"dataType\": \"Bool\",\n                    \"access\": \"ReadWrite\",\n                    \"bitfield\": \"DebugScratch32/Scratch8\"\n                },\n                {\n                    \"name\": \"NI.Scratchpad.AsBool.I8\",\n                    \"description-en\": \"registerSize=32, bitfieldSize=8, dataType=Bool\",\n                    \"documentation-en\": \"Read write 32-bit scratchpad with I8 range as Bool\",\n                    \"dataType\": \"Bool\",\n                    \"access\": \"ReadWrite\",\n                    \"bitfield\": \"DebugScratch32/ScratchI8\"\n                },\n        \n                {\n                    \"name\": \"NI.Scratchpad.AsBool.InvertBoolean\",\n                    \"dataType\": \"Bool\",\n                    \"access\": \"ReadWrite\",\n                    \"bitfield\": \"DebugScratch32/ScratchBool\",\n                    \"scale\": \"InvertBoolean\"\n                },\n                {\n                    \"name\": \"NI.Scratchpad.AsBool.TableStrictTrueFalse\",\n                    \"dataType\": \"Bool\",\n                    \"access\": \"ReadWrite\",\n                    \"bitfield\": \"DebugScratch32/ScratchI32\",\n                    \"scale\": \"TableStrictTrueFalse\"\n                },\n                {\n                    \"name\": \"NI.Scratchpad.AsBool.TableStrictFalse\",\n                    \"dataType\": \"Bool\",\n                    \"access\": \"ReadWrite\",\n                    \"bitfield\": \"DebugScratch32/ScratchI32\",\n                    \"scale\": \"TableStrictFalse\"\n                },\n                {\n                    \"name\": \"NI.Scratchpad.AsBool.TableStrictTrue\",\n                    \"dataType\": \"Bool\",\n                    \"access\": \"ReadWrite\",\n                    \"bitfield\": \"DebugScratch32/ScratchI32\",\n                    \"scale\": \"TableStrictTrue\"\n                },\n                {\n                    \"name\": \"NI.Scratchpad.AsBool.Bool\",\n                    \"description-en\": \"registerSize=32, bitfieldSize=1, dataType=Bool\",\n                    \"documentation-en\": \"Read write 32-bit scratchpad with 1 bit range as Bool\",\n                    \"dataType\": \"Bool\",\n                    \"access\": \"ReadWrite\",\n                    \"bitfield\": \"DebugScratch32/ScratchBool\"\n                },\n                {\n                    \"name\": \"NI.Scratchpad.AsDouble\",\n                    \"description-en\": \"use 32-bit Scratchpad as Double\",\n                    \"documentation-en\": \"Read write 32-bit scratchpad with Double value\",\n                    \"dataType\": \"Double\",\n                    \"access\": \"ReadWrite\",\n                    \"bitfield\": \"DebugScratch32/ScratchI32\"\n                },\n                {\n                    \"name\": \"NI.Scratchpad.AsDouble.U32\",\n                    \"description-en\": \"registerSize=32, bitfieldSize=32, dataType=Double\",\n                    \"documentation-en\": \"Read write 32-bit scratchpad with U32 range as Double\",\n                    \"dataType\": \"Double\",\n                    \"access\": \"ReadWrite\",\n                    \"bitfield\": \"DebugScratch32/Scratch32\"\n                },\n                {\n                    \"name\": \"NI.Scratchpad.AsDouble.I32\",\n                    \"description-en\": \"registerSize=32, bitfieldSize=32, dataType=Double\",\n                    \"documentation-en\": \"Read write 32-bit scratchpad with I32 range as Double\",\n                    \"dataType\": \"Double\",\n                    \"access\": \"ReadWrite\",\n                    \"bitfield\": \"DebugScratch32/ScratchI32\"\n                },\n                {\n                    \"name\": \"NI.Scratchpad.AsDouble.U16\",\n                    \"description-en\": \"registerSize=32, bitfieldSize=16, dataType=Double\",\n                    \"documentation-en\": \"Read write 32-bit scratchpad with U16 range as Double\",\n                    \"dataType\": \"Double\",\n                    \"access\": \"ReadWrite\",\n                    \"bitfield\": \"DebugScratch32/Scratch16\"\n                },\n                {\n                    \"name\": \"NI.Scratchpad.AsDouble.I16\",\n                    \"description-en\": \"registerSize=32, bitfieldSize=16, dataType=Double\",\n                    \"documentation-en\": \"Read write 32-bit scratchpad with I16 range as Double\",\n                    \"dataType\": \"Double\",\n                    \"access\": \"ReadWrite\",\n                    \"bitfield\": \"DebugScratch32/ScratchI16\"\n                },\n                {\n                    \"name\": \"NI.Scratchpad.AsDouble.U8\",\n                    \"description-en\": \"registerSize=32, bitfieldSize=8, dataType=Double\",\n                    \"documentation-en\": \"Read write 32-bit scratchpad with U8 range as Double\",\n                    \"dataType\": \"Double\",\n                    \"access\": \"ReadWrite\",\n                    \"bitfield\": \"DebugScratch32/Scratch8\"\n                },\n                {\n                    \"name\": \"NI.Scratchpad.AsDouble.I8\",\n                    \"description-en\": \"registerSize=32, bitfieldSize=8, dataType=Double\",\n                    \"documentation-en\": \"Read write 32-bit scratchpad with I8 range as Double\",\n                    \"dataType\": \"Double\",\n                    \"access\": \"ReadWrite\",\n                    \"bitfield\": \"DebugScratch32/ScratchI8\"\n                },\n        \n                {\n                    \"name\": \"NI.Scratchpad.AsDouble.TableStrict\",\n                    \"dataType\": \"Double\",\n                    \"access\": \"ReadWrite\",\n                    \"bitfield\": \"DebugScratch32/ScratchI32\",\n                    \"scale\": \"TableStrict\"\n                },\n                {\n                    \"name\": \"NI.Scratchpad.AsDouble.TableStrict12Elements\",\n                    \"dataType\": \"Double\",\n                    \"access\": \"ReadWrite\",\n                    \"bitfield\": \"DebugScratch32/ScratchI32\",\n                    \"scale\": \"TableStrict12Elements\"\n                },\n                {\n                    \"name\": \"NI.Scratchpad.AsDouble.TableRound\",\n                    \"dataType\": \"Double\",\n                    \"access\": \"ReadWrite\",\n                    \"bitfield\": \"DebugScratch32/ScratchI32\",\n                    \"scale\": \"TableRound\"\n                },\n                {\n                    \"name\": \"NI.Scratchpad.AsDouble.TableInterpolate\",\n                    \"dataType\": \"Double\",\n                    \"access\": \"ReadWrite\",\n                    \"bitfield\": \"DebugScratch32/ScratchI32\",\n                    \"scale\": \"TableInterpolate\"\n                },\n                {\n                    \"name\": \"NI.Scratchpad.AsDouble.LinearDivideBy8\",\n                    \"dataType\": \"Double\",\n                    \"access\": \"ReadWrite\",\n                    \"bitfield\": \"DebugScratch32/ScratchI32\",\n                    \"scale\": \"LinearDivideBy8\"\n                },\n                {\n                    \"name\": \"NI.Scratchpad.AsDouble.Times2Plus2\",\n                    \"dataType\": \"Double\",\n                    \"access\": \"ReadWrite\",\n                    \"bitfield\": \"DebugScratch32/ScratchI32\",\n                    \"scale\": \"Times2Plus2\"\n                },\n                {\n                    \"name\": \"NI.Scratchpad.AsDouble.PolynomialThermocouple\",\n                    \"dataType\": \"Double\",\n                    \"access\": \"ReadWrite\",\n                    \"bitfield\": \"DebugScratch32/ScratchI32\",\n                    \"scale\": \"PolynomialThermocouple\",\n                    \"min\": 0,\n                    \"max\": 760\n                },\n                {\n                    \"name\": \"NI.Scratchpad.AsDouble.PolynomialBoundaryConditions\",\n                    \"dataType\": \"Double\",\n                    \"access\": \"ReadWrite\",\n                    \"bitfield\": \"DebugScratch32/ScratchI32\",\n                    \"scale\": \"PolynomialBoundaryConditions\"\n                },\n                {\n                    \"name\": \"NI.Scratchpad.AsDouble.Bool\",\n                    \"description-en\": \"registerSize=32, bitfieldSize=1, dataType=Double\",\n                    \"documentation-en\": \"Read write 32-bit scratchpad with 1 bit range as Double\",\n                    \"dataType\": \"Double\",\n                    \"access\": \"ReadWrite\",\n                    \"bitfield\": \"DebugScratch32/ScratchBool\"\n                },\n                {\n                    \"name\": \"NI.Scratchpad.AsInt32\",\n                    \"description-en\": \"use 32-bit Scratchpad as Int32\",\n                    \"documentation-en\": \"Read write 32-bit scratchpad with Int32 value\",\n                    \"dataType\": \"Int32\",\n                    \"access\": \"ReadWrite\",\n                    \"bitfield\": \"DebugScratch32/ScratchI32\"\n                },\n                {\n                    \"name\": \"NI.Scratchpad.AsInt32.U32\",\n                    \"description-en\": \"registerSize=32, bitfieldSize=32, dataType=Int32\",\n                    \"documentation-en\": \"Read write 32-bit scratchpad with U32 range as Int32\",\n                    \"dataType\": \"Int32\",\n                    \"access\": \"ReadWrite\",\n                    \"bitfield\": \"DebugScratch32/Scratch32\"\n                },\n                {\n                    \"name\": \"NI.Scratchpad.AsInt32.I32\",\n                    \"description-en\": \"registerSize=32, bitfieldSize=32, dataType=Int32\",\n                    \"documentation-en\": \"Read write 32-bit scratchpad with I32 range as Int32\",\n                    \"dataType\": \"Int32\",\n                    \"access\": \"ReadWrite\",\n                    \"bitfield\": \"DebugScratch32/ScratchI32\"\n                },\n                {\n                    \"name\": \"NI.Scratchpad.AsInt32.U16\",\n                    \"description-en\": \"registerSize=32, bitfieldSize=16, dataType=Int32\",\n                    \"documentation-en\": \"Read write 32-bit scratchpad with U16 range as Int32\",\n                    \"dataType\": \"Int32\",\n                    \"access\": \"ReadWrite\",\n                    \"bitfield\": \"DebugScratch32/Scratch16\"\n                },\n                {\n                    \"name\": \"NI.Scratchpad.AsInt32.I16\",\n                    \"description-en\": \"registerSize=32, bitfieldSize=16, dataType=Int32\",\n                    \"documentation-en\": \"Read write 32-bit scratchpad with I16 range as Int32\",\n                    \"dataType\": \"Int32\",\n                    \"access\": \"ReadWrite\",\n                    \"bitfield\": \"DebugScratch32/ScratchI16\"\n                },\n                {\n                    \"name\": \"NI.Scratchpad.AsInt32.U8\",\n                    \"description-en\": \"registerSize=32, bitfieldSize=8, dataType=Int32\",\n                    \"documentation-en\": \"Read write 32-bit scratchpad with U8 range as Int32\",\n                    \"dataType\": \"Int32\",\n                    \"access\": \"ReadWrite\",\n                    \"bitfield\": \"DebugScratch32/Scratch8\"\n                },\n                {\n                    \"name\": \"NI.Scratchpad.AsInt32.I8\",\n                    \"description-en\": \"registerSize=32, bitfieldSize=8, dataType=Int32\",\n                    \"documentation-en\": \"Read write 32-bit scratchpad with I8 range as Int32\",\n                    \"dataType\": \"Int32\",\n                    \"access\": \"ReadWrite\",\n                    \"bitfield\": \"DebugScratch32/ScratchI8\"\n                },\n        \n                {\n                    \"name\": \"NI.Scratchpad.AsInt32.TableStrict12Elements\",\n                    \"dataType\": \"Int32\",\n                    \"access\": \"ReadWrite\",\n                    \"bitfield\": \"DebugScratch32/ScratchI32\",\n                    \"scale\": \"TableStrict12Elements\"\n                },\n                {\n                    \"name\": \"NI.Scratchpad.AsInt32.TableRound\",\n                    \"dataType\": \"Int32\",\n                    \"access\": \"ReadWrite\",\n                    \"bitfield\": \"DebugScratch32/ScratchI32\",\n                    \"scale\": \"TableRound\"\n                },\n                {\n                    \"name\": \"NI.Scratchpad.AsInt32.TableInterpolate\",\n                    \"dataType\": \"Int32\",\n                    \"access\": \"ReadWrite\",\n                    \"bitfield\": \"DebugScratch32/ScratchI32\",\n                    \"scale\": \"TableInterpolate\"\n                },\n                {\n                    \"name\": \"NI.Scratchpad.AsInt32.LinearDivideBy8\",\n                    \"dataType\": \"Int32\",\n                    \"access\": \"ReadWrite\",\n                    \"bitfield\": \"DebugScratch32/ScratchI32\",\n                    \"scale\": \"LinearDivideBy8\"\n                },\n                {\n                    \"name\": \"NI.Scratchpad.AsInt32.Times2Plus2\",\n                    \"dataType\": \"Int32\",\n                    \"access\": \"ReadWrite\",\n                    \"bitfield\": \"DebugScratch32/ScratchI32\",\n                    \"scale\": \"Times2Plus2\"\n                },\n                {\n                    \"name\": \"NI.Scratchpad.AsInt32.PolynomialThermocouple\",\n                    \"dataType\": \"Int32\",\n                    \"access\": \"ReadWrite\",\n                    \"bitfield\": \"DebugScratch32/ScratchI32\",\n                    \"scale\": \"PolynomialThermocouple\",\n                    \"min\": 0,\n                    \"max\": 760\n                },\n                {\n                    \"name\": \"NI.Scratchpad.AsInt32.PolynomialBoundaryConditions\",\n                    \"dataType\": \"Int32\",\n                    \"access\": \"ReadWrite\",\n                    \"bitfield\": \"DebugScratch32/ScratchI32\",\n                    \"scale\": \"PolynomialBoundaryConditions\"\n                },\n                {\n                    \"name\": \"NI.Scratchpad.AsInt32.Bool\",\n                    \"description-en\": \"registerSize=32, bitfieldSize=1, dataType=Int32\",\n                    \"documentation-en\": \"Read write 32-bit scratchpad with 1 bit range as Int32\",\n                    \"dataType\": \"Int32\",\n                    \"access\": \"ReadWrite\",\n                    \"bitfield\": \"DebugScratch32/ScratchBool\"\n                },\n                {\n                    \"name\": \"NI.Scratchpad.AsInt64\",\n                    \"description-en\": \"use 32-bit Scratchpad as Int64\",\n                    \"documentation-en\": \"Read write 32-bit scratchpad with Int64 value\",\n                    \"dataType\": \"Int64\",\n                    \"access\": \"ReadWrite\",\n                    \"bitfield\": \"DebugScratch32/ScratchI32\"\n                },\n                {\n                    \"name\": \"NI.Scratchpad.AsInt64.U32\",\n                    \"description-en\": \"registerSize=32, bitfieldSize=32, dataType=Int64\",\n                    \"documentation-en\": \"Read write 32-bit scratchpad with U32 range as Int64\",\n                    \"dataType\": \"Int64\",\n                    \"access\": \"ReadWrite\",\n                    \"bitfield\": \"DebugScratch32/Scratch32\"\n                },\n                {\n                    \"name\": \"NI.Scratchpad.AsInt64.I32\",\n                    \"description-en\": \"registerSize=32, bitfieldSize=32, dataType=Int64\",\n                    \"documentation-en\": \"Read write 32-bit scratchpad with I32 range as Int64\",\n                    \"dataType\": \"Int64\",\n                    \"access\": \"ReadWrite\",\n                    \"bitfield\": \"DebugScratch32/ScratchI32\"\n                },\n                {\n                    \"name\": \"NI.Scratchpad.AsInt64.U16\",\n                    \"description-en\": \"registerSize=32, bitfieldSize=16, dataType=Int64\",\n                    \"documentation-en\": \"Read write 32-bit scratchpad with U16 range as Int64\",\n                    \"dataType\": \"Int64\",\n                    \"access\": \"ReadWrite\",\n                    \"bitfield\": \"DebugScratch32/Scratch16\"\n                },\n                {\n                    \"name\": \"NI.Scratchpad.AsInt64.I16\",\n                    \"description-en\": \"registerSize=32, bitfieldSize=16, dataType=Int64\",\n                    \"documentation-en\": \"Read write 32-bit scratchpad with I16 range as Int64\",\n                    \"dataType\": \"Int64\",\n                    \"access\": \"ReadWrite\",\n                    \"bitfield\": \"DebugScratch32/ScratchI16\"\n                },\n                {\n                    \"name\": \"NI.Scratchpad.AsInt64.U8\",\n                    \"description-en\": \"registerSize=32, bitfieldSize=8, dataType=Int64\",\n                    \"documentation-en\": \"Read write 32-bit scratchpad with U8 range as Int64\",\n                    \"dataType\": \"Int64\",\n                    \"access\": \"ReadWrite\",\n                    \"bitfield\": \"DebugScratch32/Scratch8\"\n                },\n                {\n                    \"name\": \"NI.Scratchpad.AsInt64.I8\",\n                    \"description-en\": \"registerSize=32, bitfieldSize=8, dataType=Int64\",\n                    \"documentation-en\": \"Read write 32-bit scratchpad with I8 range as Int64\",\n                    \"dataType\": \"Int64\",\n                    \"access\": \"ReadWrite\",\n                    \"bitfield\": \"DebugScratch32/ScratchI8\"\n                },\n        \n                {\n                    \"name\": \"NI.Scratchpad.AsInt64.TableStrict12Elements\",\n                    \"dataType\": \"Int64\",\n                    \"access\": \"ReadWrite\",\n                    \"bitfield\": \"DebugScratch32/ScratchI32\",\n                    \"scale\": \"TableStrict12Elements\"\n                },\n                {\n                    \"name\": \"NI.Scratchpad.AsInt64.TableRound\",\n                    \"dataType\": \"Int64\",\n                    \"access\": \"ReadWrite\",\n                    \"bitfield\": \"DebugScratch32/ScratchI32\",\n                    \"scale\": \"TableRound\"\n                },\n                {\n                    \"name\": \"NI.Scratchpad.AsInt64.TableInterpolate\",\n                    \"dataType\": \"Int64\",\n                    \"access\": \"ReadWrite\",\n                    \"bitfield\": \"DebugScratch32/ScratchI32\",\n                    \"scale\": \"TableInterpolate\"\n                },\n                {\n                    \"name\": \"NI.Scratchpad.AsInt64.LinearDivideBy8\",\n                    \"dataType\": \"Int64\",\n                    \"access\": \"ReadWrite\",\n                    \"bitfield\": \"DebugScratch32/ScratchI32\",\n                    \"scale\": \"LinearDivideBy8\"\n                },\n                {\n                    \"name\": \"NI.Scratchpad.AsInt64.Times2Plus2\",\n                    \"dataType\": \"Int64\",\n                    \"access\": \"ReadWrite\",\n                    \"bitfield\": \"DebugScratch32/ScratchI32\",\n                    \"scale\": \"Times2Plus2\"\n                },\n                {\n                    \"name\": \"NI.Scratchpad.AsInt64.PolynomialThermocouple\",\n                    \"dataType\": \"Int64\",\n                    \"access\": \"ReadWrite\",\n                    \"bitfield\": \"DebugScratch32/ScratchI32\",\n                    \"scale\": \"PolynomialThermocouple\",\n                    \"min\": 0,\n                    \"max\": 760\n                },\n                {\n                    \"name\": \"NI.Scratchpad.AsInt64.PolynomialBoundaryConditions\",\n                    \"dataType\": \"Int64\",\n                    \"access\": \"ReadWrite\",\n                    \"bitfield\": \"DebugScratch32/ScratchI32\",\n                    \"scale\": \"PolynomialBoundaryConditions\"\n                },\n                {\n                    \"name\": \"NI.Scratchpad.AsInt64.Bool\",\n                    \"description-en\": \"registerSize=32, bitfieldSize=1, dataType=Int64\",\n                    \"documentation-en\": \"Read write 32-bit scratchpad with 1 bit range as Int64\",\n                    \"dataType\": \"Int64\",\n                    \"access\": \"ReadWrite\",\n                    \"bitfield\": \"DebugScratch32/ScratchBool\"\n                },\n                {\n                    \"name\": \"NI.Scratchpad.AsUInt32\",\n                    \"description-en\": \"use 32-bit Scratchpad as UInt32\",\n                    \"documentation-en\": \"Read write 32-bit scratchpad with UInt32 value\",\n                    \"dataType\": \"UInt32\",\n                    \"access\": \"ReadWrite\",\n                    \"bitfield\": \"DebugScratch32/Scratch32\"\n                },\n                {\n                    \"name\": \"NI.Scratchpad.AsUInt32.U32\",\n                    \"description-en\": \"registerSize=32, bitfieldSize=32, dataType=UInt32\",\n                    \"documentation-en\": \"Read write 32-bit scratchpad with U32 range as UInt32\",\n                    \"dataType\": \"UInt32\",\n                    \"access\": \"ReadWrite\",\n                    \"bitfield\": \"DebugScratch32/Scratch32\"\n                },\n                {\n                    \"name\": \"NI.Scratchpad.AsUInt32.I32\",\n                    \"description-en\": \"registerSize=32, bitfieldSize=32, dataType=UInt32\",\n                    \"documentation-en\": \"Read write 32-bit scratchpad with I32 range as UInt32\",\n                    \"dataType\": \"UInt32\",\n                    \"access\": \"ReadWrite\",\n                    \"bitfield\": \"DebugScratch32/ScratchI32\"\n                },\n                {\n                    \"name\": \"NI.Scratchpad.AsUInt32.U16\",\n                    \"description-en\": \"registerSize=32, bitfieldSize=16, dataType=UInt32\",\n                    \"documentation-en\": \"Read write 32-bit scratchpad with U16 range as UInt32\",\n                    \"dataType\": \"UInt32\",\n                    \"access\": \"ReadWrite\",\n                    \"bitfield\": \"DebugScratch32/Scratch16\"\n                },\n                {\n                    \"name\": \"NI.Scratchpad.AsUInt32.I16\",\n                    \"description-en\": \"registerSize=32, bitfieldSize=16, dataType=UInt32\",\n                    \"documentation-en\": \"Read write 32-bit scratchpad with I16 range as UInt32\",\n                    \"dataType\": \"UInt32\",\n                    \"access\": \"ReadWrite\",\n                    \"bitfield\": \"DebugScratch32/ScratchI16\"\n                },\n                {\n                    \"name\": \"NI.Scratchpad.AsUInt32.U8\",\n                    \"description-en\": \"registerSize=32, bitfieldSize=8, dataType=UInt32\",\n                    \"documentation-en\": \"Read write 32-bit scratchpad with U8 range as UInt32\",\n                    \"dataType\": \"UInt32\",\n                    \"access\": \"ReadWrite\",\n                    \"bitfield\": \"DebugScratch32/Scratch8\"\n                },\n                {\n                    \"name\": \"NI.Scratchpad.AsUInt32.I8\",\n                    \"description-en\": \"registerSize=32, bitfieldSize=8, dataType=UInt32\",\n                    \"documentation-en\": \"Read write 32-bit scratchpad with I8 range as UInt32\",\n                    \"dataType\": \"UInt32\",\n                    \"access\": \"ReadWrite\",\n                    \"bitfield\": \"DebugScratch32/ScratchI8\"\n                },\n        \n                {\n                    \"name\": \"NI.Scratchpad.AsUInt32.TableStrict12Elements\",\n                    \"dataType\": \"UInt32\",\n                    \"access\": \"ReadWrite\",\n                    \"bitfield\": \"DebugScratch32/Scratch32\",\n                    \"scale\": \"TableStrict12Elements\"\n                },\n                {\n                    \"name\": \"NI.Scratchpad.AsUInt32.TableRound\",\n                    \"dataType\": \"UInt32\",\n                    \"access\": \"ReadWrite\",\n                    \"bitfield\": \"DebugScratch32/Scratch32\",\n                    \"scale\": \"TableRound\"\n                },\n                {\n                    \"name\": \"NI.Scratchpad.AsUInt32.TableInterpolate\",\n                    \"dataType\": \"UInt32\",\n                    \"access\": \"ReadWrite\",\n                    \"bitfield\": \"DebugScratch32/Scratch32\",\n                    \"scale\": \"TableInterpolate\"\n                },\n                {\n                    \"name\": \"NI.Scratchpad.AsUInt32.LinearDivideBy8\",\n                    \"dataType\": \"UInt32\",\n                    \"access\": \"ReadWrite\",\n                    \"bitfield\": \"DebugScratch32/Scratch32\",\n                    \"scale\": \"LinearDivideBy8\"\n                },\n                {\n                    \"name\": \"NI.Scratchpad.AsUInt32.Times2Plus2\",\n                    \"dataType\": \"UInt32\",\n                    \"access\": \"ReadWrite\",\n                    \"bitfield\": \"DebugScratch32/Scratch32\",\n                    \"scale\": \"Times2Plus2\"\n                },\n                {\n                    \"name\": \"NI.Scratchpad.AsUInt32.PolynomialThermocouple\",\n                    \"dataType\": \"UInt32\",\n                    \"access\": \"ReadWrite\",\n                    \"bitfield\": \"DebugScratch32/Scratch32\",\n                    \"scale\": \"PolynomialThermocouple\",\n                    \"min\": 0,\n                    \"max\": 760\n                },\n                {\n                    \"name\": \"NI.Scratchpad.AsUInt32.PolynomialBoundaryConditions\",\n                    \"dataType\": \"UInt32\",\n                    \"access\": \"ReadWrite\",\n                    \"bitfield\": \"DebugScratch32/Scratch32\",\n                    \"scale\": \"PolynomialBoundaryConditions\"\n                },\n                {\n                    \"name\": \"NI.Scratchpad.AsUInt32.Bool\",\n                    \"description-en\": \"registerSize=32, bitfieldSize=1, dataType=UInt32\",\n                    \"documentation-en\": \"Read write 32-bit scratchpad with 1 bit range as UInt32\",\n                    \"dataType\": \"UInt32\",\n                    \"access\": \"ReadWrite\",\n                    \"bitfield\": \"DebugScratch32/ScratchBool\"\n                },\n                {\n                    \"name\": \"NI.Scratchpad.AsUInt64\",\n                    \"description-en\": \"use 32-bit Scratchpad as UInt64\",\n                    \"documentation-en\": \"Read write 32-bit scratchpad with UInt64 value\",\n                    \"dataType\": \"UInt64\",\n                    \"access\": \"ReadWrite\",\n                    \"bitfield\": \"DebugScratch32/Scratch32\"\n                },\n                {\n                    \"name\": \"NI.Scratchpad.AsUInt64.U32\",\n                    \"description-en\": \"registerSize=32, bitfieldSize=32, dataType=UInt64\",\n                    \"documentation-en\": \"Read write 32-bit scratchpad with U32 range as UInt64\",\n                    \"dataType\": \"UInt64\",\n                    \"access\": \"ReadWrite\",\n                    \"bitfield\": \"DebugScratch32/Scratch32\"\n                },\n                {\n                    \"name\": \"NI.Scratchpad.AsUInt64.I32\",\n                    \"description-en\": \"registerSize=32, bitfieldSize=32, dataType=UInt64\",\n                    \"documentation-en\": \"Read write 32-bit scratchpad with I32 range as UInt64\",\n                    \"dataType\": \"UInt64\",\n                    \"access\": \"ReadWrite\",\n                    \"bitfield\": \"DebugScratch32/ScratchI32\"\n                },\n                {\n                    \"name\": \"NI.Scratchpad.AsUInt64.U16\",\n                    \"description-en\": \"registerSize=32, bitfieldSize=16, dataType=UInt64\",\n                    \"documentation-en\": \"Read write 32-bit scratchpad with U16 range as UInt64\",\n                    \"dataType\": \"UInt64\",\n                    \"access\": \"ReadWrite\",\n                    \"bitfield\": \"DebugScratch32/Scratch16\"\n                },\n                {\n                    \"name\": \"NI.Scratchpad.AsUInt64.I16\",\n                    \"description-en\": \"registerSize=32, bitfieldSize=16, dataType=UInt64\",\n                    \"documentation-en\": \"Read write 32-bit scratchpad with I16 range as UInt64\",\n                    \"dataType\": \"UInt64\",\n                    \"access\": \"ReadWrite\",\n                    \"bitfield\": \"DebugScratch32/ScratchI16\"\n                },\n                {\n                    \"name\": \"NI.Scratchpad.AsUInt64.U8\",\n                    \"description-en\": \"registerSize=32, bitfieldSize=8, dataType=UInt64\",\n                    \"documentation-en\": \"Read write 32-bit scratchpad with U8 range as UInt64\",\n                    \"dataType\": \"UInt64\",\n                    \"access\": \"ReadWrite\",\n                    \"bitfield\": \"DebugScratch32/Scratch8\"\n                },\n                {\n                    \"name\": \"NI.Scratchpad.AsUInt64.I8\",\n                    \"description-en\": \"registerSize=32, bitfieldSize=8, dataType=UInt64\",\n                    \"documentation-en\": \"Read write 32-bit scratchpad with I8 range as UInt64\",\n                    \"dataType\": \"UInt64\",\n                    \"access\": \"ReadWrite\",\n                    \"bitfield\": \"DebugScratch32/ScratchI8\"\n                },\n        \n                {\n                    \"name\": \"NI.Scratchpad.AsUInt64.TableStrict12Elements\",\n                    \"dataType\": \"UInt64\",\n                    \"access\": \"ReadWrite\",\n                    \"bitfield\": \"DebugScratch32/Scratch32\",\n                    \"scale\": \"TableStrict12Elements\"\n                },\n                {\n                    \"name\": \"NI.Scratchpad.AsUInt64.TableRound\",\n                    \"dataType\": \"UInt64\",\n                    \"access\": \"ReadWrite\",\n                    \"bitfield\": \"DebugScratch32/Scratch32\",\n                    \"scale\": \"TableRound\"\n                },\n                {\n                    \"name\": \"NI.Scratchpad.AsUInt64.TableInterpolate\",\n                    \"dataType\": \"UInt64\",\n                    \"access\": \"ReadWrite\",\n                    \"bitfield\": \"DebugScratch32/Scratch32\",\n                    \"scale\": \"TableInterpolate\"\n                },\n                {\n                    \"name\": \"NI.Scratchpad.AsUInt64.LinearDivideBy8\",\n                    \"dataType\": \"UInt64\",\n                    \"access\": \"ReadWrite\",\n                    \"bitfield\": \"DebugScratch32/Scratch32\",\n                    \"scale\": \"LinearDivideBy8\"\n                },\n                {\n                    \"name\": \"NI.Scratchpad.AsUInt64.Times2Plus2\",\n                    \"dataType\": \"UInt64\",\n                    \"access\": \"ReadWrite\",\n                    \"bitfield\": \"DebugScratch32/Scratch32\",\n                    \"scale\": \"Times2Plus2\"\n                },\n                {\n                    \"name\": \"NI.Scratchpad.AsUInt64.PolynomialThermocouple\",\n                    \"dataType\": \"UInt64\",\n                    \"access\": \"ReadWrite\",\n                    \"bitfield\": \"DebugScratch32/Scratch32\",\n                    \"scale\": \"PolynomialThermocouple\",\n                    \"min\": 0,\n                    \"max\": 760\n                },\n                {\n                    \"name\": \"NI.Scratchpad.AsUInt64.PolynomialBoundaryConditions\",\n                    \"dataType\": \"UInt64\",\n                    \"access\": \"ReadWrite\",\n                    \"bitfield\": \"DebugScratch32/Scratch32\",\n                    \"scale\": \"PolynomialBoundaryConditions\"\n                },\n                {\n                    \"name\": \"NI.Scratchpad.AsUInt64.Bool\",\n                    \"description-en\": \"registerSize=32, bitfieldSize=1, dataType=UInt64\",\n                    \"documentation-en\": \"Read write 32-bit scratchpad with 1 bit range as UInt64\",\n                    \"dataType\": \"UInt64\",\n                    \"access\": \"ReadWrite\",\n                    \"bitfield\": \"DebugScratch32/ScratchBool\"\n                }\n            ]\n        },\n        {\n            \"name\": \"Scratchpad16\",\n            \"properties\": [\n                {\n                   \"name\": \"NI.ChannelName\",\n                   \"dataType\": \"String\",\n                   \"value\": \"Scratchpad16\"\n                },\n                {\n                    \"name\": \"NI.Scratchpad.RegisterSize\",\n                    \"description-en\": \"Indicates the width of the register backing this physical channel\",\n                    \"dataType\": \"Int32\",\n                    \"value\": 16\n                },\n                {\n                    \"name\": \"NI.Scratchpad.AsBool\",\n                    \"description-en\": \"use 16-bit Scratchpad as Bool\",\n                    \"documentation-en\": \"Read write 16-bit scratchpad with Bool value\",\n                    \"dataType\": \"Bool\",\n                    \"access\": \"ReadWrite\",\n                    \"bitfield\": \"DebugScratch16/ScratchBool\"\n                },\n                {\n                    \"name\": \"NI.Scratchpad.AsBool.U16\",\n                    \"description-en\": \"registerSize=16, bitfieldSize=16, dataType=Bool\",\n                    \"documentation-en\": \"Read write 16-bit scratchpad with U16 range as Bool\",\n                    \"dataType\": \"Bool\",\n                    \"access\": \"ReadWrite\",\n                    \"bitfield\": \"DebugScratch16/Scratch16\"\n                },\n                {\n                    \"name\": \"NI.Scratchpad.AsBool.I16\",\n                    \"description-en\": \"registerSize=16, bitfieldSize=16, dataType=Bool\",\n                    \"documentation-en\": \"Read write 16-bit scratchpad with I16 range as Bool\",\n                    \"dataType\": \"Bool\",\n                    \"access\": \"ReadWrite\",\n                    \"bitfield\": \"DebugScratch16/ScratchI16\"\n                },\n                {\n                    \"name\": \"NI.Scratchpad.AsBool.U8\",\n                    \"description-en\": \"registerSize=16, bitfieldSize=8, dataType=Bool\",\n                    \"documentation-en\": \"Read write 16-bit scratchpad with U8 range as Bool\",\n                    \"dataType\": \"Bool\",\n                    \"access\": \"ReadWrite\",\n                    \"bitfield\": \"DebugScratch16/Scratch8\"\n                },\n                {\n                    \"name\": \"NI.Scratchpad.AsBool.I8\",\n                    \"description-en\": \"registerSize=16, bitfieldSize=8, dataType=Bool\",\n                    \"documentation-en\": \"Read write 16-bit scratchpad with I8 range as Bool\",\n                    \"dataType\": \"Bool\",\n                    \"access\": \"ReadWrite\",\n                    \"bitfield\": \"DebugScratch16/ScratchI8\"\n                },\n        \n                {\n                    \"name\": \"NI.Scratchpad.AsBool.InvertBoolean\",\n                    \"dataType\": \"Bool\",\n                    \"access\": \"ReadWrite\",\n                    \"bitfield\": \"DebugScratch16/ScratchBool\",\n                    \"scale\": \"InvertBoolean\"\n                },\n                {\n                    \"name\": \"NI.Scratchpad.AsBool.TableStrictTrueFalse\",\n                    \"dataType\": \"Bool\",\n                    \"access\": \"ReadWrite\",\n                    \"bitfield\": \"DebugScratch16/ScratchI16\",\n                    \"scale\": \"TableStrictTrueFalse\"\n                },\n                {\n                    \"name\": \"NI.Scratchpad.AsBool.TableStrictFalse\",\n                    \"dataType\": \"Bool\",\n                    \"access\": \"ReadWrite\",\n                    \"bitfield\": \"DebugScratch16/ScratchI16\",\n                    \"scale\": \"TableStrictFalse\"\n                },\n                {\n                    \"name\": \"NI.Scratchpad.AsBool.TableStrictTrue\",\n                    \"dataType\": \"Bool\",\n                    \"access\": \"ReadWrite\",\n                    \"bitfield\": \"DebugScratch16/ScratchI16\",\n                    \"scale\": \"TableStrictTrue\"\n                },\n                {\n                    \"name\": \"NI.Scratchpad.AsBool.Bool\",\n                    \"description-en\": \"registerSize=16, bitfieldSize=1, dataType=Bool\",\n                    \"documentation-en\": \"Read write 16-bit scratchpad with 1 bit range as Bool\",\n                    \"dataType\": \"Bool\",\n                    \"access\": \"ReadWrite\",\n                    \"bitfield\": \"DebugScratch16/ScratchBool\"\n                },\n                {\n                    \"name\": \"NI.Scratchpad.AsDouble\",\n                    \"description-en\": \"use 16-bit Scratchpad as Double\",\n                    \"documentation-en\": \"Read write 16-bit scratchpad with Double value\",\n                    \"dataType\": \"Double\",\n                    \"access\": \"ReadWrite\",\n                    \"bitfield\": \"DebugScratch16/ScratchI16\"\n                },\n                {\n                    \"name\": \"NI.Scratchpad.AsDouble.U16\",\n                    \"description-en\": \"registerSize=16, bitfieldSize=16, dataType=Double\",\n                    \"documentation-en\": \"Read write 16-bit scratchpad with U16 range as Double\",\n                    \"dataType\": \"Double\",\n                    \"access\": \"ReadWrite\",\n                    \"bitfield\": \"DebugScratch16/Scratch16\"\n                },\n                {\n                    \"name\": \"NI.Scratchpad.AsDouble.I16\",\n                    \"description-en\": \"registerSize=16, bitfieldSize=16, dataType=Double\",\n                    \"documentation-en\": \"Read write 16-bit scratchpad with I16 range as Double\",\n                    \"dataType\": \"Double\",\n                    \"access\": \"ReadWrite\",\n                    \"bitfield\": \"DebugScratch16/ScratchI16\"\n                },\n                {\n                    \"name\": \"NI.Scratchpad.AsDouble.U8\",\n                    \"description-en\": \"registerSize=16, bitfieldSize=8, dataType=Double\",\n                    \"documentation-en\": \"Read write 16-bit scratchpad with U8 range as Double\",\n                    \"dataType\": \"Double\",\n                    \"access\": \"ReadWrite\",\n                    \"bitfield\": \"DebugScratch16/Scratch8\"\n                },\n                {\n                    \"name\": \"NI.Scratchpad.AsDouble.I8\",\n                    \"description-en\": \"registerSize=16, bitfieldSize=8, dataType=Double\",\n                    \"documentation-en\": \"Read write 16-bit scratchpad with I8 range as Double\",\n                    \"dataType\": \"Double\",\n                    \"access\": \"ReadWrite\",\n                    \"bitfield\": \"DebugScratch16/ScratchI8\"\n                },\n        \n                {\n                    \"name\": \"NI.Scratchpad.AsDouble.TableStrict\",\n                    \"dataType\": \"Double\",\n                    \"access\": \"ReadWrite\",\n                    \"bitfield\": \"DebugScratch16/ScratchI16\",\n                    \"scale\": \"TableStrict\"\n                },\n                {\n                    \"name\": \"NI.Scratchpad.AsDouble.TableStrict12Elements\",\n                    \"dataType\": \"Double\",\n                    \"access\": \"ReadWrite\",\n                    \"bitfield\": \"DebugScratch16/ScratchI16\",\n                    \"scale\": \"TableStrict12Elements\"\n                },\n                {\n                    \"name\": \"NI.Scratchpad.AsDouble.TableRound\",\n                    \"dataType\": \"Double\",\n                    \"access\": \"ReadWrite\",\n                    \"bitfield\": \"DebugScratch16/ScratchI16\",\n                    \"scale\": \"TableRound\"\n                },\n                {\n                    \"name\": \"NI.Scratchpad.AsDouble.TableInterpolate\",\n                    \"dataType\": \"Double\",\n                    \"access\": \"ReadWrite\",\n                    \"bitfield\": \"DebugScratch16/ScratchI16\",\n                    \"scale\": \"TableInterpolate\"\n                },\n                {\n                    \"name\": \"NI.Scratchpad.AsDouble.LinearDivideBy8\",\n                    \"dataType\": \"Double\",\n                    \"access\": \"ReadWrite\",\n                    \"bitfield\": \"DebugScratch16/ScratchI16\",\n                    \"scale\": \"LinearDivideBy8\"\n                },\n                {\n                    \"name\": \"NI.Scratchpad.AsDouble.Times2Plus2\",\n                    \"dataType\": \"Double\",\n                    \"access\": \"ReadWrite\",\n                    \"bitfield\": \"DebugScratch16/ScratchI16\",\n                    \"scale\": \"Times2Plus2\"\n                },\n                {\n                    \"name\": \"NI.Scratchpad.AsDouble.PolynomialThermocouple\",\n                    \"dataType\": \"Double\",\n                    \"access\": \"ReadWrite\",\n                    \"bitfield\": \"DebugScratch16/ScratchI16\",\n                    \"scale\": \"PolynomialThermocouple\",\n                    \"min\": 0,\n                    \"max\": 760\n                },\n                {\n                    \"name\": \"NI.Scratchpad.AsDouble.PolynomialBoundaryConditions\",\n                    \"dataType\": \"Double\",\n                    \"access\": \"ReadWrite\",\n                    \"bitfield\": \"DebugScratch16/ScratchI16\",\n                    \"scale\": \"PolynomialBoundaryConditions\"\n                },\n                {\n                    \"name\": \"NI.Scratchpad.AsDouble.Bool\",\n                    \"description-en\": \"registerSize=16, bitfieldSize=1, dataType=Double\",\n                    \"documentation-en\": \"Read write 16-bit scratchpad with 1 bit range as Double\",\n                    \"dataType\": \"Double\",\n                    \"access\": \"ReadWrite\",\n                    \"bitfield\": \"DebugScratch16/ScratchBool\"\n                },\n                {\n                    \"name\": \"NI.Scratchpad.AsInt32\",\n                    \"description-en\": \"use 16-bit Scratchpad as Int32\",\n                    \"documentation-en\": \"Read write 16-bit scratchpad with Int32 value\",\n                    \"dataType\": \"Int32\",\n                    \"access\": \"ReadWrite\",\n                    \"bitfield\": \"DebugScratch16/ScratchI16\"\n                },\n                {\n                    \"name\": \"NI.Scratchpad.AsInt32.U16\",\n                    \"description-en\": \"registerSize=16, bitfieldSize=16, dataType=Int32\",\n                    \"documentation-en\": \"Read write 16-bit scratchpad with U16 range as Int32\",\n                    \"dataType\": \"Int32\",\n                    \"access\": \"ReadWrite\",\n                    \"bitfield\": \"DebugScratch16/Scratch16\"\n                },\n                {\n                    \"name\": \"NI.Scratchpad.AsInt32.I16\",\n                    \"description-en\": \"registerSize=16, bitfieldSize=16, dataType=Int32\",\n                    \"documentation-en\": \"Read write 16-bit scratchpad with I16 range as Int32\",\n                    \"dataType\": \"Int32\",\n                    \"access\": \"ReadWrite\",\n                    \"bitfield\": \"DebugScratch16/ScratchI16\"\n                },\n                {\n                    \"name\": \"NI.Scratchpad.AsInt32.U8\",\n                    \"description-en\": \"registerSize=16, bitfieldSize=8, dataType=Int32\",\n                    \"documentation-en\": \"Read write 16-bit scratchpad with U8 range as Int32\",\n                    \"dataType\": \"Int32\",\n                    \"access\": \"ReadWrite\",\n                    \"bitfield\": \"DebugScratch16/Scratch8\"\n                },\n                {\n                    \"name\": \"NI.Scratchpad.AsInt32.I8\",\n                    \"description-en\": \"registerSize=16, bitfieldSize=8, dataType=Int32\",\n                    \"documentation-en\": \"Read write 16-bit scratchpad with I8 range as Int32\",\n                    \"dataType\": \"Int32\",\n                    \"access\": \"ReadWrite\",\n                    \"bitfield\": \"DebugScratch16/ScratchI8\"\n                },\n        \n                {\n                    \"name\": \"NI.Scratchpad.AsInt32.TableStrict12Elements\",\n                    \"dataType\": \"Int32\",\n                    \"access\": \"ReadWrite\",\n                    \"bitfield\": \"DebugScratch16/ScratchI16\",\n                    \"scale\": \"TableStrict12Elements\"\n                },\n                {\n                    \"name\": \"NI.Scratchpad.AsInt32.TableRound\",\n                    \"dataType\": \"Int32\",\n                    \"access\": \"ReadWrite\",\n                    \"bitfield\": \"DebugScratch16/ScratchI16\",\n                    \"scale\": \"TableRound\"\n                },\n                {\n                    \"name\": \"NI.Scratchpad.AsInt32.TableInterpolate\",\n                    \"dataType\": \"Int32\",\n                    \"access\": \"ReadWrite\",\n                    \"bitfield\": \"DebugScratch16/ScratchI16\",\n                    \"scale\": \"TableInterpolate\"\n                },\n                {\n                    \"name\": \"NI.Scratchpad.AsInt32.LinearDivideBy8\",\n                    \"dataType\": \"Int32\",\n                    \"access\": \"ReadWrite\",\n                    \"bitfield\": \"DebugScratch16/ScratchI16\",\n                    \"scale\": \"LinearDivideBy8\"\n                },\n                {\n                    \"name\": \"NI.Scratchpad.AsInt32.Times2Plus2\",\n                    \"dataType\": \"Int32\",\n                    \"access\": \"ReadWrite\",\n                    \"bitfield\": \"DebugScratch16/ScratchI16\",\n                    \"scale\": \"Times2Plus2\"\n                },\n                {\n                    \"name\": \"NI.Scratchpad.AsInt32.PolynomialThermocouple\",\n                    \"dataType\": \"Int32\",\n                    \"access\": \"ReadWrite\",\n                    \"bitfield\": \"DebugScratch16/ScratchI16\",\n                    \"scale\": \"PolynomialThermocouple\",\n                    \"min\": 0,\n                    \"max\": 760\n                },\n                {\n                    \"name\": \"NI.Scratchpad.AsInt32.PolynomialBoundaryConditions\",\n                    \"dataType\": \"Int32\",\n                    \"access\": \"ReadWrite\",\n                    \"bitfield\": \"DebugScratch16/ScratchI16\",\n                    \"scale\": \"PolynomialBoundaryConditions\"\n                },\n                {\n                    \"name\": \"NI.Scratchpad.AsInt32.Bool\",\n                    \"description-en\": \"registerSize=16, bitfieldSize=1, dataType=Int32\",\n                    \"documentation-en\": \"Read write 16-bit scratchpad with 1 bit range as Int32\",\n                    \"dataType\": \"Int32\",\n                    \"access\": \"ReadWrite\",\n                    \"bitfield\": \"DebugScratch16/ScratchBool\"\n                },\n                {\n                    \"name\": \"NI.Scratchpad.AsInt64\",\n                    \"description-en\": \"use 16-bit Scratchpad as Int64\",\n                    \"documentation-en\": \"Read write 16-bit scratchpad with Int64 value\",\n                    \"dataType\": \"Int64\",\n                    \"access\": \"ReadWrite\",\n                    \"bitfield\": \"DebugScratch16/ScratchI16\"\n                },\n                {\n                    \"name\": \"NI.Scratchpad.AsInt64.U16\",\n                    \"description-en\": \"registerSize=16, bitfieldSize=16, dataType=Int64\",\n                    \"documentation-en\": \"Read write 16-bit scratchpad with U16 range as Int64\",\n                    \"dataType\": \"Int64\",\n                    \"access\": \"ReadWrite\",\n                    \"bitfield\": \"DebugScratch16/Scratch16\"\n                },\n                {\n                    \"name\": \"NI.Scratchpad.AsInt64.I16\",\n                    \"description-en\": \"registerSize=16, bitfieldSize=16, dataType=Int64\",\n                    \"documentation-en\": \"Read write 16-bit scratchpad with I16 range as Int64\",\n                    \"dataType\": \"Int64\",\n                    \"access\": \"ReadWrite\",\n                    \"bitfield\": \"DebugScratch16/ScratchI16\"\n                },\n                {\n                    \"name\": \"NI.Scratchpad.AsInt64.U8\",\n                    \"description-en\": \"registerSize=16, bitfieldSize=8, dataType=Int64\",\n                    \"documentation-en\": \"Read write 16-bit scratchpad with U8 range as Int64\",\n                    \"dataType\": \"Int64\",\n                    \"access\": \"ReadWrite\",\n                    \"bitfield\": \"DebugScratch16/Scratch8\"\n                },\n                {\n                    \"name\": \"NI.Scratchpad.AsInt64.I8\",\n                    \"description-en\": \"registerSize=16, bitfieldSize=8, dataType=Int64\",\n                    \"documentation-en\": \"Read write 16-bit scratchpad with I8 range as Int64\",\n                    \"dataType\": \"Int64\",\n                    \"access\": \"ReadWrite\",\n                    \"bitfield\": \"DebugScratch16/ScratchI8\"\n                },\n        \n                {\n                    \"name\": \"NI.Scratchpad.AsInt64.TableStrict12Elements\",\n                    \"dataType\": \"Int64\",\n                    \"access\": \"ReadWrite\",\n                    \"bitfield\": \"DebugScratch16/ScratchI16\",\n                    \"scale\": \"TableStrict12Elements\"\n                },\n                {\n                    \"name\": \"NI.Scratchpad.AsInt64.TableRound\",\n                    \"dataType\": \"Int64\",\n                    \"access\": \"ReadWrite\",\n                    \"bitfield\": \"DebugScratch16/ScratchI16\",\n                    \"scale\": \"TableRound\"\n                },\n                {\n                    \"name\": \"NI.Scratchpad.AsInt64.TableInterpolate\",\n                    \"dataType\": \"Int64\",\n                    \"access\": \"ReadWrite\",\n                    \"bitfield\": \"DebugScratch16/ScratchI16\",\n                    \"scale\": \"TableInterpolate\"\n                },\n                {\n                    \"name\": \"NI.Scratchpad.AsInt64.LinearDivideBy8\",\n                    \"dataType\": \"Int64\",\n                    \"access\": \"ReadWrite\",\n                    \"bitfield\": \"DebugScratch16/ScratchI16\",\n                    \"scale\": \"LinearDivideBy8\"\n                },\n                {\n                    \"name\": \"NI.Scratchpad.AsInt64.Times2Plus2\",\n                    \"dataType\": \"Int64\",\n                    \"access\": \"ReadWrite\",\n                    \"bitfield\": \"DebugScratch16/ScratchI16\",\n                    \"scale\": \"Times2Plus2\"\n                },\n                {\n                    \"name\": \"NI.Scratchpad.AsInt64.PolynomialThermocouple\",\n                    \"dataType\": \"Int64\",\n                    \"access\": \"ReadWrite\",\n                    \"bitfield\": \"DebugScratch16/ScratchI16\",\n                    \"scale\": \"PolynomialThermocouple\",\n                    \"min\": 0,\n                    \"max\": 760\n                },\n                {\n                    \"name\": \"NI.Scratchpad.AsInt64.PolynomialBoundaryConditions\",\n                    \"dataType\": \"Int64\",\n                    \"access\": \"ReadWrite\",\n                    \"bitfield\": \"DebugScratch16/ScratchI16\",\n                    \"scale\": \"PolynomialBoundaryConditions\"\n                },\n                {\n                    \"name\": \"NI.Scratchpad.AsInt64.Bool\",\n                    \"description-en\": \"registerSize=16, bitfieldSize=1, dataType=Int64\",\n                    \"documentation-en\": \"Read write 16-bit scratchpad with 1 bit range as Int64\",\n                    \"dataType\": \"Int64\",\n                    \"access\": \"ReadWrite\",\n                    \"bitfield\": \"DebugScratch16/ScratchBool\"\n                },\n                {\n                    \"name\": \"NI.Scratchpad.AsUInt32\",\n                    \"description-en\": \"use 16-bit Scratchpad as UInt32\",\n                    \"documentation-en\": \"Read write 16-bit scratchpad with UInt32 value\",\n                    \"dataType\": \"UInt32\",\n                    \"access\": \"ReadWrite\",\n                    \"bitfield\": \"DebugScratch16/Scratch16\"\n                },\n                {\n                    \"name\": \"NI.Scratchpad.AsUInt32.U16\",\n                    \"description-en\": \"registerSize=16, bitfieldSize=16, dataType=UInt32\",\n                    \"documentation-en\": \"Read write 16-bit scratchpad with U16 range as UInt32\",\n                    \"dataType\": \"UInt32\",\n                    \"access\": \"ReadWrite\",\n                    \"bitfield\": \"DebugScratch16/Scratch16\"\n                },\n                {\n                    \"name\": \"NI.Scratchpad.AsUInt32.I16\",\n                    \"description-en\": \"registerSize=16, bitfieldSize=16, dataType=UInt32\",\n                    \"documentation-en\": \"Read write 16-bit scratchpad with I16 range as UInt32\",\n                    \"dataType\": \"UInt32\",\n                    \"access\": \"ReadWrite\",\n                    \"bitfield\": \"DebugScratch16/ScratchI16\"\n                },\n                {\n                    \"name\": \"NI.Scratchpad.AsUInt32.U8\",\n                    \"description-en\": \"registerSize=16, bitfieldSize=8, dataType=UInt32\",\n                    \"documentation-en\": \"Read write 16-bit scratchpad with U8 range as UInt32\",\n                    \"dataType\": \"UInt32\",\n                    \"access\": \"ReadWrite\",\n                    \"bitfield\": \"DebugScratch16/Scratch8\"\n                },\n                {\n                    \"name\": \"NI.Scratchpad.AsUInt32.I8\",\n                    \"description-en\": \"registerSize=16, bitfieldSize=8, dataType=UInt32\",\n                    \"documentation-en\": \"Read write 16-bit scratchpad with I8 range as UInt32\",\n                    \"dataType\": \"UInt32\",\n                    \"access\": \"ReadWrite\",\n                    \"bitfield\": \"DebugScratch16/ScratchI8\"\n                },\n        \n                {\n                    \"name\": \"NI.Scratchpad.AsUInt32.TableStrict12Elements\",\n                    \"dataType\": \"UInt32\",\n                    \"access\": \"ReadWrite\",\n                    \"bitfield\": \"DebugScratch16/Scratch16\",\n                    \"scale\": \"TableStrict12Elements\"\n                },\n                {\n                    \"name\": \"NI.Scratchpad.AsUInt32.TableRound\",\n                    \"dataType\": \"UInt32\",\n                    \"access\": \"ReadWrite\",\n                    \"bitfield\": \"DebugScratch16/Scratch16\",\n                    \"scale\": \"TableRound\"\n                },\n                {\n                    \"name\": \"NI.Scratchpad.AsUInt32.TableInterpolate\",\n                    \"dataType\": \"UInt32\",\n                    \"access\": \"ReadWrite\",\n                    \"bitfield\": \"DebugScratch16/Scratch16\",\n                    \"scale\": \"TableInterpolate\"\n                },\n                {\n                    \"name\": \"NI.Scratchpad.AsUInt32.LinearDivideBy8\",\n                    \"dataType\": \"UInt32\",\n                    \"access\": \"ReadWrite\",\n                    \"bitfield\": \"DebugScratch16/Scratch16\",\n                    \"scale\": \"LinearDivideBy8\"\n                },\n                {\n                    \"name\": \"NI.Scratchpad.AsUInt32.Times2Plus2\",\n                    \"dataType\": \"UInt32\",\n                    \"access\": \"ReadWrite\",\n                    \"bitfield\": \"DebugScratch16/Scratch16\",\n                    \"scale\": \"Times2Plus2\"\n                },\n                {\n                    \"name\": \"NI.Scratchpad.AsUInt32.PolynomialThermocouple\",\n                    \"dataType\": \"UInt32\",\n                    \"access\": \"ReadWrite\",\n                    \"bitfield\": \"DebugScratch16/Scratch16\",\n                    \"scale\": \"PolynomialThermocouple\",\n                    \"min\": 0,\n                    \"max\": 760\n                },\n                {\n                    \"name\": \"NI.Scratchpad.AsUInt32.PolynomialBoundaryConditions\",\n                    \"dataType\": \"UInt32\",\n                    \"access\": \"ReadWrite\",\n                    \"bitfield\": \"DebugScratch16/Scratch16\",\n                    \"scale\": \"PolynomialBoundaryConditions\"\n                },\n                {\n                    \"name\": \"NI.Scratchpad.AsUInt32.Bool\",\n                    \"description-en\": \"registerSize=16, bitfieldSize=1, dataType=UInt32\",\n                    \"documentation-en\": \"Read write 16-bit scratchpad with 1 bit range as UInt32\",\n                    \"dataType\": \"UInt32\",\n                    \"access\": \"ReadWrite\",\n                    \"bitfield\": \"DebugScratch16/ScratchBool\"\n                },\n                {\n                    \"name\": \"NI.Scratchpad.AsUInt64\",\n                    \"description-en\": \"use 16-bit Scratchpad as UInt64\",\n                    \"documentation-en\": \"Read write 16-bit scratchpad with UInt64 value\",\n                    \"dataType\": \"UInt64\",\n                    \"access\": \"ReadWrite\",\n                    \"bitfield\": \"DebugScratch16/Scratch16\"\n                },\n                {\n                    \"name\": \"NI.Scratchpad.AsUInt64.U16\",\n                    \"description-en\": \"registerSize=16, bitfieldSize=16, dataType=UInt64\",\n                    \"documentation-en\": \"Read write 16-bit scratchpad with U16 range as UInt64\",\n                    \"dataType\": \"UInt64\",\n                    \"access\": \"ReadWrite\",\n                    \"bitfield\": \"DebugScratch16/Scratch16\"\n                },\n                {\n                    \"name\": \"NI.Scratchpad.AsUInt64.I16\",\n                    \"description-en\": \"registerSize=16, bitfieldSize=16, dataType=UInt64\",\n                    \"documentation-en\": \"Read write 16-bit scratchpad with I16 range as UInt64\",\n                    \"dataType\": \"UInt64\",\n                    \"access\": \"ReadWrite\",\n                    \"bitfield\": \"DebugScratch16/ScratchI16\"\n                },\n                {\n                    \"name\": \"NI.Scratchpad.AsUInt64.U8\",\n                    \"description-en\": \"registerSize=16, bitfieldSize=8, dataType=UInt64\",\n                    \"documentation-en\": \"Read write 16-bit scratchpad with U8 range as UInt64\",\n                    \"dataType\": \"UInt64\",\n                    \"access\": \"ReadWrite\",\n                    \"bitfield\": \"DebugScratch16/Scratch8\"\n                },\n                {\n                    \"name\": \"NI.Scratchpad.AsUInt64.I8\",\n                    \"description-en\": \"registerSize=16, bitfieldSize=8, dataType=UInt64\",\n                    \"documentation-en\": \"Read write 16-bit scratchpad with I8 range as UInt64\",\n                    \"dataType\": \"UInt64\",\n                    \"access\": \"ReadWrite\",\n                    \"bitfield\": \"DebugScratch16/ScratchI8\"\n                },\n        \n                {\n                    \"name\": \"NI.Scratchpad.AsUInt64.TableStrict12Elements\",\n                    \"dataType\": \"UInt64\",\n                    \"access\": \"ReadWrite\",\n                    \"bitfield\": \"DebugScratch16/Scratch16\",\n                    \"scale\": \"TableStrict12Elements\"\n                },\n                {\n                    \"name\": \"NI.Scratchpad.AsUInt64.TableRound\",\n                    \"dataType\": \"UInt64\",\n                    \"access\": \"ReadWrite\",\n                    \"bitfield\": \"DebugScratch16/Scratch16\",\n                    \"scale\": \"TableRound\"\n                },\n                {\n                    \"name\": \"NI.Scratchpad.AsUInt64.TableInterpolate\",\n                    \"dataType\": \"UInt64\",\n                    \"access\": \"ReadWrite\",\n                    \"bitfield\": \"DebugScratch16/Scratch16\",\n                    \"scale\": \"TableInterpolate\"\n                },\n                {\n                    \"name\": \"NI.Scratchpad.AsUInt64.LinearDivideBy8\",\n                    \"dataType\": \"UInt64\",\n                    \"access\": \"ReadWrite\",\n                    \"bitfield\": \"DebugScratch16/Scratch16\",\n                    \"scale\": \"LinearDivideBy8\"\n                },\n                {\n                    \"name\": \"NI.Scratchpad.AsUInt64.Times2Plus2\",\n                    \"dataType\": \"UInt64\",\n                    \"access\": \"ReadWrite\",\n                    \"bitfield\": \"DebugScratch16/Scratch16\",\n                    \"scale\": \"Times2Plus2\"\n                },\n                {\n                    \"name\": \"NI.Scratchpad.AsUInt64.PolynomialThermocouple\",\n                    \"dataType\": \"UInt64\",\n                    \"access\": \"ReadWrite\",\n                    \"bitfield\": \"DebugScratch16/Scratch16\",\n                    \"scale\": \"PolynomialThermocouple\",\n                    \"min\": 0,\n                    \"max\": 760\n                },\n                {\n                    \"name\": \"NI.Scratchpad.AsUInt64.PolynomialBoundaryConditions\",\n                    \"dataType\": \"UInt64\",\n                    \"access\": \"ReadWrite\",\n                    \"bitfield\": \"DebugScratch16/Scratch16\",\n                    \"scale\": \"PolynomialBoundaryConditions\"\n                },\n                {\n                    \"name\": \"NI.Scratchpad.AsUInt64.Bool\",\n                    \"description-en\": \"registerSize=16, bitfieldSize=1, dataType=UInt64\",\n                    \"documentation-en\": \"Read write 16-bit scratchpad with 1 bit range as UInt64\",\n                    \"dataType\": \"UInt64\",\n                    \"access\": \"ReadWrite\",\n                    \"bitfield\": \"DebugScratch16/ScratchBool\"\n                }\n            ]\n        },\n        {\n            \"name\": \"Scratchpad8\",\n            \"properties\": [\n                {\n                   \"name\": \"NI.ChannelName\",\n                   \"dataType\": \"String\",\n                   \"value\": \"Scratchpad8\"\n                },\n                {\n                    \"name\": \"NI.Scratchpad.RegisterSize\",\n                    \"description-en\": \"Indicates the width of the register backing this physical channel\",\n                    \"dataType\": \"Int32\",\n                    \"value\": 8\n                },\n                {\n                    \"name\": \"NI.Scratchpad.AsBool\",\n                    \"description-en\": \"use 8-bit Scratchpad as Bool\",\n                    \"documentation-en\": \"Read write 8-bit scratchpad with Bool value\",\n                    \"dataType\": \"Bool\",\n                    \"access\": \"ReadWrite\",\n                    \"bitfield\": \"DebugScratch8/ScratchBool\"\n                },\n                {\n                    \"name\": \"NI.Scratchpad.AsBool.U8\",\n                    \"description-en\": \"registerSize=8, bitfieldSize=8, dataType=Bool\",\n                    \"documentation-en\": \"Read write 8-bit scratchpad with U8 range as Bool\",\n                    \"dataType\": \"Bool\",\n                    \"access\": \"ReadWrite\",\n                    \"bitfield\": \"DebugScratch8/Scratch8\"\n                },\n                {\n                    \"name\": \"NI.Scratchpad.AsBool.I8\",\n                    \"description-en\": \"registerSize=8, bitfieldSize=8, dataType=Bool\",\n                    \"documentation-en\": \"Read write 8-bit scratchpad with I8 range as Bool\",\n                    \"dataType\": \"Bool\",\n                    \"access\": \"ReadWrite\",\n                    \"bitfield\": \"DebugScratch8/ScratchI8\"\n                },\n        \n                {\n                    \"name\": \"NI.Scratchpad.AsBool.InvertBoolean\",\n                    \"dataType\": \"Bool\",\n                    \"access\": \"ReadWrite\",\n                    \"bitfield\": \"DebugScratch8/ScratchBool\",\n                    \"scale\": \"InvertBoolean\"\n                },\n                {\n                    \"name\": \"NI.Scratchpad.AsBool.TableStrictTrueFalse\",\n                    \"dataType\": \"Bool\",\n                    \"access\": \"ReadWrite\",\n                    \"bitfield\": \"DebugScratch8/ScratchI8\",\n                    \"scale\": \"TableStrictTrueFalse\"\n                },\n                {\n                    \"name\": \"NI.Scratchpad.AsBool.TableStrictFalse\",\n                    \"dataType\": \"Bool\",\n                    \"access\": \"ReadWrite\",\n                    \"bitfield\": \"DebugScratch8/ScratchI8\",\n                    \"scale\": \"TableStrictFalse\"\n                },\n                {\n                    \"name\": \"NI.Scratchpad.AsBool.TableStrictTrue\",\n                    \"dataType\": \"Bool\",\n                    \"access\": \"ReadWrite\",\n                    \"bitfield\": \"DebugScratch8/ScratchI8\",\n                    \"scale\": \"TableStrictTrue\"\n                },\n                {\n                    \"name\": \"NI.Scratchpad.AsBool.Bool\",\n                    \"description-en\": \"registerSize=8, bitfieldSize=1, dataType=Bool\",\n                    \"documentation-en\": \"Read write 8-bit scratchpad with 1 bit range as Bool\",\n                    \"dataType\": \"Bool\",\n                    \"access\": \"ReadWrite\",\n                    \"bitfield\": \"DebugScratch8/ScratchBool\"\n                },\n                {\n                    \"name\": \"NI.Scratchpad.AsDouble\",\n                    \"description-en\": \"use 8-bit Scratchpad as Double\",\n                    \"documentation-en\": \"Read write 8-bit scratchpad with Double value\",\n                    \"dataType\": \"Double\",\n                    \"access\": \"ReadWrite\",\n                    \"bitfield\": \"DebugScratch8/ScratchI8\"\n                },\n                {\n                    \"name\": \"NI.Scratchpad.AsDouble.U8\",\n                    \"description-en\": \"registerSize=8, bitfieldSize=8, dataType=Double\",\n                    \"documentation-en\": \"Read write 8-bit scratchpad with U8 range as Double\",\n                    \"dataType\": \"Double\",\n                    \"access\": \"ReadWrite\",\n                    \"bitfield\": \"DebugScratch8/Scratch8\"\n                },\n                {\n                    \"name\": \"NI.Scratchpad.AsDouble.I8\",\n                    \"description-en\": \"registerSize=8, bitfieldSize=8, dataType=Double\",\n                    \"documentation-en\": \"Read write 8-bit scratchpad with I8 range as Double\",\n                    \"dataType\": \"Double\",\n                    \"access\": \"ReadWrite\",\n                    \"bitfield\": \"DebugScratch8/ScratchI8\"\n                },\n        \n                {\n                    \"name\": \"NI.Scratchpad.AsDouble.TableStrict\",\n                    \"dataType\": \"Double\",\n                    \"access\": \"ReadWrite\",\n                    \"bitfield\": \"DebugScratch8/ScratchI8\",\n                    \"scale\": \"TableStrict\"\n                },\n                {\n                    \"name\": \"NI.Scratchpad.AsDouble.TableStrict12Elements\",\n                    \"dataType\": \"Double\",\n                    \"access\": \"ReadWrite\",\n                    \"bitfield\": \"DebugScratch8/ScratchI8\",\n                    \"scale\": \"TableStrict12Elements\"\n                },\n                {\n                    \"name\": \"NI.Scratchpad.AsDouble.TableRound\",\n                    \"dataType\": \"Double\",\n                    \"access\": \"ReadWrite\",\n                    \"bitfield\": \"DebugScratch8/ScratchI8\",\n                    \"scale\": \"TableRound\"\n                },\n                {\n                    \"name\": \"NI.Scratchpad.AsDouble.TableInterpolate\",\n                    \"dataType\": \"Double\",\n                    \"access\": \"ReadWrite\",\n                    \"bitfield\": \"DebugScratch8/ScratchI8\",\n                    \"scale\": \"TableInterpolate\"\n                },\n                {\n                    \"name\": \"NI.Scratchpad.AsDouble.LinearDivideBy8\",\n                    \"dataType\": \"Double\",\n                    \"access\": \"ReadWrite\",\n                    \"bitfield\": \"DebugScratch8/ScratchI8\",\n                    \"scale\": \"LinearDivideBy8\"\n                },\n                {\n                    \"name\": \"NI.Scratchpad.AsDouble.Times2Plus2\",\n                    \"dataType\": \"Double\",\n                    \"access\": \"ReadWrite\",\n                    \"bitfield\": \"DebugScratch8/ScratchI8\",\n                    \"scale\": \"Times2Plus2\"\n                },\n                {\n                    \"name\": \"NI.Scratchpad.AsDouble.PolynomialThermocouple\",\n                    \"dataType\": \"Double\",\n                    \"access\": \"ReadWrite\",\n                    \"bitfield\": \"DebugScratch8/ScratchI8\",\n                    \"scale\": \"PolynomialThermocouple\",\n                    \"min\": 0,\n                    \"max\": 760\n                },\n                {\n                    \"name\": \"NI.Scratchpad.AsDouble.PolynomialBoundaryConditions\",\n                    \"dataType\": \"Double\",\n                    \"access\": \"ReadWrite\",\n                    \"bitfield\": \"DebugScratch8/ScratchI8\",\n                    \"scale\": \"PolynomialBoundaryConditions\"\n                },\n                {\n                    \"name\": \"NI.Scratchpad.AsDouble.Bool\",\n                    \"description-en\": \"registerSize=8, bitfieldSize=1, dataType=Double\",\n                    \"documentation-en\": \"Read write 8-bit scratchpad with 1 bit range as Double\",\n                    \"dataType\": \"Double\",\n                    \"access\": \"ReadWrite\",\n                    \"bitfield\": \"DebugScratch8/ScratchBool\"\n                },\n                {\n                    \"name\": \"NI.Scratchpad.AsInt32\",\n                    \"description-en\": \"use 8-bit Scratchpad as Int32\",\n                    \"documentation-en\": \"Read write 8-bit scratchpad with Int32 value\",\n                    \"dataType\": \"Int32\",\n                    \"access\": \"ReadWrite\",\n                    \"bitfield\": \"DebugScratch8/ScratchI8\"\n                },\n                {\n                    \"name\": \"NI.Scratchpad.AsInt32.U8\",\n                    \"description-en\": \"registerSize=8, bitfieldSize=8, dataType=Int32\",\n                    \"documentation-en\": \"Read write 8-bit scratchpad with U8 range as Int32\",\n                    \"dataType\": \"Int32\",\n                    \"access\": \"ReadWrite\",\n                    \"bitfield\": \"DebugScratch8/Scratch8\"\n                },\n                {\n                    \"name\": \"NI.Scratchpad.AsInt32.I8\",\n                    \"description-en\": \"registerSize=8, bitfieldSize=8, dataType=Int32\",\n                    \"documentation-en\": \"Read write 8-bit scratchpad with I8 range as Int32\",\n                    \"dataType\": \"Int32\",\n                    \"access\": \"ReadWrite\",\n                    \"bitfield\": \"DebugScratch8/ScratchI8\"\n                },\n        \n                {\n                    \"name\": \"NI.Scratchpad.AsInt32.TableStrict12Elements\",\n                    \"dataType\": \"Int32\",\n                    \"access\": \"ReadWrite\",\n                    \"bitfield\": \"DebugScratch8/ScratchI8\",\n                    \"scale\": \"TableStrict12Elements\"\n                },\n                {\n                    \"name\": \"NI.Scratchpad.AsInt32.TableRound\",\n                    \"dataType\": \"Int32\",\n                    \"access\": \"ReadWrite\",\n                    \"bitfield\": \"DebugScratch8/ScratchI8\",\n                    \"scale\": \"TableRound\"\n                },\n                {\n                    \"name\": \"NI.Scratchpad.AsInt32.TableInterpolate\",\n                    \"dataType\": \"Int32\",\n                    \"access\": \"ReadWrite\",\n                    \"bitfield\": \"DebugScratch8/ScratchI8\",\n                    \"scale\": \"TableInterpolate\"\n                },\n                {\n                    \"name\": \"NI.Scratchpad.AsInt32.LinearDivideBy8\",\n                    \"dataType\": \"Int32\",\n                    \"access\": \"ReadWrite\",\n                    \"bitfield\": \"DebugScratch8/ScratchI8\",\n                    \"scale\": \"LinearDivideBy8\"\n                },\n                {\n                    \"name\": \"NI.Scratchpad.AsInt32.Times2Plus2\",\n                    \"dataType\": \"Int32\",\n                    \"access\": \"ReadWrite\",\n                    \"bitfield\": \"DebugScratch8/ScratchI8\",\n                    \"scale\": \"Times2Plus2\"\n                },\n                {\n                    \"name\": \"NI.Scratchpad.AsInt32.PolynomialThermocouple\",\n                    \"dataType\": \"Int32\",\n                    \"access\": \"ReadWrite\",\n                    \"bitfield\": \"DebugScratch8/ScratchI8\",\n                    \"scale\": \"PolynomialThermocouple\",\n                    \"min\": 0,\n                    \"max\": 760\n                },\n                {\n                    \"name\": \"NI.Scratchpad.AsInt32.PolynomialBoundaryConditions\",\n                    \"dataType\": \"Int32\",\n                    \"access\": \"ReadWrite\",\n                    \"bitfield\": \"DebugScratch8/ScratchI8\",\n                    \"scale\": \"PolynomialBoundaryConditions\"\n                },\n                {\n                    \"name\": \"NI.Scratchpad.AsInt32.Bool\",\n                    \"description-en\": \"registerSize=8, bitfieldSize=1, dataType=Int32\",\n                    \"documentation-en\": \"Read write 8-bit scratchpad with 1 bit range as Int32\",\n                    \"dataType\": \"Int32\",\n                    \"access\": \"ReadWrite\",\n                    \"bitfield\": \"DebugScratch8/ScratchBool\"\n                },\n                {\n                    \"name\": \"NI.Scratchpad.AsInt64\",\n                    \"description-en\": \"use 8-bit Scratchpad as Int64\",\n                    \"documentation-en\": \"Read write 8-bit scratchpad with Int64 value\",\n                    \"dataType\": \"Int64\",\n                    \"access\": \"ReadWrite\",\n                    \"bitfield\": \"DebugScratch8/ScratchI8\"\n                },\n                {\n                    \"name\": \"NI.Scratchpad.AsInt64.U8\",\n                    \"description-en\": \"registerSize=8, bitfieldSize=8, dataType=Int64\",\n                    \"documentation-en\": \"Read write 8-bit scratchpad with U8 range as Int64\",\n                    \"dataType\": \"Int64\",\n                    \"access\": \"ReadWrite\",\n                    \"bitfield\": \"DebugScratch8/Scratch8\"\n                },\n                {\n                    \"name\": \"NI.Scratchpad.AsInt64.I8\",\n                    \"description-en\": \"registerSize=8, bitfieldSize=8, dataType=Int64\",\n                    \"documentation-en\": \"Read write 8-bit scratchpad with I8 range as Int64\",\n                    \"dataType\": \"Int64\",\n                    \"access\": \"ReadWrite\",\n                    \"bitfield\": \"DebugScratch8/ScratchI8\"\n                },\n        \n                {\n                    \"name\": \"NI.Scratchpad.AsInt64.TableStrict12Elements\",\n                    \"dataType\": \"Int64\",\n                    \"access\": \"ReadWrite\",\n                    \"bitfield\": \"DebugScratch8/ScratchI8\",\n                    \"scale\": \"TableStrict12Elements\"\n                },\n                {\n                    \"name\": \"NI.Scratchpad.AsInt64.TableRound\",\n                    \"dataType\": \"Int64\",\n                    \"access\": \"ReadWrite\",\n                    \"bitfield\": \"DebugScratch8/ScratchI8\",\n                    \"scale\": \"TableRound\"\n                },\n                {\n                    \"name\": \"NI.Scratchpad.AsInt64.TableInterpolate\",\n                    \"dataType\": \"Int64\",\n                    \"access\": \"ReadWrite\",\n                    \"bitfield\": \"DebugScratch8/ScratchI8\",\n                    \"scale\": \"TableInterpolate\"\n                },\n                {\n                    \"name\": \"NI.Scratchpad.AsInt64.LinearDivideBy8\",\n                    \"dataType\": \"Int64\",\n                    \"access\": \"ReadWrite\",\n                    \"bitfield\": \"DebugScratch8/ScratchI8\",\n                    \"scale\": \"LinearDivideBy8\"\n                },\n                {\n                    \"name\": \"NI.Scratchpad.AsInt64.Times2Plus2\",\n                    \"dataType\": \"Int64\",\n                    \"access\": \"ReadWrite\",\n                    \"bitfield\": \"DebugScratch8/ScratchI8\",\n                    \"scale\": \"Times2Plus2\"\n                },\n                {\n                    \"name\": \"NI.Scratchpad.AsInt64.PolynomialThermocouple\",\n                    \"dataType\": \"Int64\",\n                    \"access\": \"ReadWrite\",\n                    \"bitfield\": \"DebugScratch8/ScratchI8\",\n                    \"scale\": \"PolynomialThermocouple\",\n                    \"min\": 0,\n                    \"max\": 760\n                },\n                {\n                    \"name\": \"NI.Scratchpad.AsInt64.PolynomialBoundaryConditions\",\n                    \"dataType\": \"Int64\",\n                    \"access\": \"ReadWrite\",\n                    \"bitfield\": \"DebugScratch8/ScratchI8\",\n                    \"scale\": \"PolynomialBoundaryConditions\"\n                },\n                {\n                    \"name\": \"NI.Scratchpad.AsInt64.Bool\",\n                    \"description-en\": \"registerSize=8, bitfieldSize=1, dataType=Int64\",\n                    \"documentation-en\": \"Read write 8-bit scratchpad with 1 bit range as Int64\",\n                    \"dataType\": \"Int64\",\n                    \"access\": \"ReadWrite\",\n                    \"bitfield\": \"DebugScratch8/ScratchBool\"\n                },\n                {\n                    \"name\": \"NI.Scratchpad.AsUInt32\",\n                    \"description-en\": \"use 8-bit Scratchpad as UInt32\",\n                    \"documentation-en\": \"Read write 8-bit scratchpad with UInt32 value\",\n                    \"dataType\": \"UInt32\",\n                    \"access\": \"ReadWrite\",\n                    \"bitfield\": \"DebugScratch8/Scratch8\"\n                },\n                {\n                    \"name\": \"NI.Scratchpad.AsUInt32.U8\",\n                    \"description-en\": \"registerSize=8, bitfieldSize=8, dataType=UInt32\",\n                    \"documentation-en\": \"Read write 8-bit scratchpad with U8 range as UInt32\",\n                    \"dataType\": \"UInt32\",\n                    \"access\": \"ReadWrite\",\n                    \"bitfield\": \"DebugScratch8/Scratch8\"\n                },\n                {\n                    \"name\": \"NI.Scratchpad.AsUInt32.I8\",\n                    \"description-en\": \"registerSize=8, bitfieldSize=8, dataType=UInt32\",\n                    \"documentation-en\": \"Read write 8-bit scratchpad with I8 range as UInt32\",\n                    \"dataType\": \"UInt32\",\n                    \"access\": \"ReadWrite\",\n                    \"bitfield\": \"DebugScratch8/ScratchI8\"\n                },\n        \n                {\n                    \"name\": \"NI.Scratchpad.AsUInt32.TableStrict12Elements\",\n                    \"dataType\": \"UInt32\",\n                    \"access\": \"ReadWrite\",\n                    \"bitfield\": \"DebugScratch8/Scratch8\",\n                    \"scale\": \"TableStrict12Elements\"\n                },\n                {\n                    \"name\": \"NI.Scratchpad.AsUInt32.TableRound\",\n                    \"dataType\": \"UInt32\",\n                    \"access\": \"ReadWrite\",\n                    \"bitfield\": \"DebugScratch8/Scratch8\",\n                    \"scale\": \"TableRound\"\n                },\n                {\n                    \"name\": \"NI.Scratchpad.AsUInt32.TableInterpolate\",\n                    \"dataType\": \"UInt32\",\n                    \"access\": \"ReadWrite\",\n                    \"bitfield\": \"DebugScratch8/Scratch8\",\n                    \"scale\": \"TableInterpolate\"\n                },\n                {\n                    \"name\": \"NI.Scratchpad.AsUInt32.LinearDivideBy8\",\n                    \"dataType\": \"UInt32\",\n                    \"access\": \"ReadWrite\",\n                    \"bitfield\": \"DebugScratch8/Scratch8\",\n                    \"scale\": \"LinearDivideBy8\"\n                },\n                {\n                    \"name\": \"NI.Scratchpad.AsUInt32.Times2Plus2\",\n                    \"dataType\": \"UInt32\",\n                    \"access\": \"ReadWrite\",\n                    \"bitfield\": \"DebugScratch8/Scratch8\",\n                    \"scale\": \"Times2Plus2\"\n                },\n                {\n                    \"name\": \"NI.Scratchpad.AsUInt32.PolynomialThermocouple\",\n                    \"dataType\": \"UInt32\",\n                    \"access\": \"ReadWrite\",\n                    \"bitfield\": \"DebugScratch8/Scratch8\",\n                    \"scale\": \"PolynomialThermocouple\",\n                    \"min\": 0,\n                    \"max\": 760\n                },\n                {\n                    \"name\": \"NI.Scratchpad.AsUInt32.PolynomialBoundaryConditions\",\n                    \"dataType\": \"UInt32\",\n                    \"access\": \"ReadWrite\",\n                    \"bitfield\": \"DebugScratch8/Scratch8\",\n                    \"scale\": \"PolynomialBoundaryConditions\"\n                },\n                {\n                    \"name\": \"NI.Scratchpad.AsUInt32.Bool\",\n                    \"description-en\": \"registerSize=8, bitfieldSize=1, dataType=UInt32\",\n                    \"documentation-en\": \"Read write 8-bit scratchpad with 1 bit range as UInt32\",\n                    \"dataType\": \"UInt32\",\n                    \"access\": \"ReadWrite\",\n                    \"bitfield\": \"DebugScratch8/ScratchBool\"\n                },\n                {\n                    \"name\": \"NI.Scratchpad.AsUInt64\",\n                    \"description-en\": \"use 8-bit Scratchpad as UInt64\",\n                    \"documentation-en\": \"Read write 8-bit scratchpad with UInt64 value\",\n                    \"dataType\": \"UInt64\",\n                    \"access\": \"ReadWrite\",\n                    \"bitfield\": \"DebugScratch8/Scratch8\"\n                },\n                {\n                    \"name\": \"NI.Scratchpad.AsUInt64.U8\",\n                    \"description-en\": \"registerSize=8, bitfieldSize=8, dataType=UInt64\",\n                    \"documentation-en\": \"Read write 8-bit scratchpad with U8 range as UInt64\",\n                    \"dataType\": \"UInt64\",\n                    \"access\": \"ReadWrite\",\n                    \"bitfield\": \"DebugScratch8/Scratch8\"\n                },\n                {\n                    \"name\": \"NI.Scratchpad.AsUInt64.I8\",\n                    \"description-en\": \"registerSize=8, bitfieldSize=8, dataType=UInt64\",\n                    \"documentation-en\": \"Read write 8-bit scratchpad with I8 range as UInt64\",\n                    \"dataType\": \"UInt64\",\n                    \"access\": \"ReadWrite\",\n                    \"bitfield\": \"DebugScratch8/ScratchI8\"\n                },\n        \n                {\n                    \"name\": \"NI.Scratchpad.AsUInt64.TableStrict12Elements\",\n                    \"dataType\": \"UInt64\",\n                    \"access\": \"ReadWrite\",\n                    \"bitfield\": \"DebugScratch8/Scratch8\",\n                    \"scale\": \"TableStrict12Elements\"\n                },\n                {\n                    \"name\": \"NI.Scratchpad.AsUInt64.TableRound\",\n                    \"dataType\": \"UInt64\",\n                    \"access\": \"ReadWrite\",\n                    \"bitfield\": \"DebugScratch8/Scratch8\",\n                    \"scale\": \"TableRound\"\n                },\n                {\n                    \"name\": \"NI.Scratchpad.AsUInt64.TableInterpolate\",\n                    \"dataType\": \"UInt64\",\n                    \"access\": \"ReadWrite\",\n                    \"bitfield\": \"DebugScratch8/Scratch8\",\n                    \"scale\": \"TableInterpolate\"\n                },\n                {\n                    \"name\": \"NI.Scratchpad.AsUInt64.LinearDivideBy8\",\n                    \"dataType\": \"UInt64\",\n                    \"access\": \"ReadWrite\",\n                    \"bitfield\": \"DebugScratch8/Scratch8\",\n                    \"scale\": \"LinearDivideBy8\"\n                },\n                {\n                    \"name\": \"NI.Scratchpad.AsUInt64.Times2Plus2\",\n                    \"dataType\": \"UInt64\",\n                    \"access\": \"ReadWrite\",\n                    \"bitfield\": \"DebugScratch8/Scratch8\",\n                    \"scale\": \"Times2Plus2\"\n                },\n                {\n                    \"name\": \"NI.Scratchpad.AsUInt64.PolynomialThermocouple\",\n                    \"dataType\": \"UInt64\",\n                    \"access\": \"ReadWrite\",\n                    \"bitfield\": \"DebugScratch8/Scratch8\",\n                    \"scale\": \"PolynomialThermocouple\",\n                    \"min\": 0,\n                    \"max\": 760\n                },\n                {\n                    \"name\": \"NI.Scratchpad.AsUInt64.PolynomialBoundaryConditions\",\n                    \"dataType\": \"UInt64\",\n                    \"access\": \"ReadWrite\",\n                    \"bitfield\": \"DebugScratch8/Scratch8\",\n                    \"scale\": \"PolynomialBoundaryConditions\"\n                },\n                {\n                    \"name\": \"NI.Scratchpad.AsUInt64.Bool\",\n                    \"description-en\": \"registerSize=8, bitfieldSize=1, dataType=UInt64\",\n                    \"documentation-en\": \"Read write 8-bit scratchpad with 1 bit range as UInt64\",\n                    \"dataType\": \"UInt64\",\n                    \"access\": \"ReadWrite\",\n                    \"bitfield\": \"DebugScratch8/ScratchBool\"\n                }\n            ]\n        }\n    ],\n\n    \"properties\": [{\n            \"name\": \"NI.DateCode\",\n            \"description-en\": \"Module CPLD Date Code\",\n            \"documentationen\": \"Date code of the image on the module CPLD\",\n            \"dataType\": \"UInt32\",\n            \"bitfield\": \"Revision/DateCode\",\n            \"access\": \"ReadOnly\"\n        },{\"name\":\"abcd\",\"description-en\":\"\",\"documentation-en\":\"\",\"dataType\":\"String\",\"value\":\"abv\"},{\"name\":\"aaa\",\"description-en\":\"\",\"documentation-en\":\"\",\"dataType\":\"String\",\"value\":\"aaa\"},{\n            \"name\": \"NI.Debug.Alphabet\",\n            \"description-en\": \"Constant string property\",\n            \"documentation-en\": \"Constant string that returns the english alphabet\",\n            \"dataType\": \"String\",\n            \"value\": \"abcdefghijklmnopqrstuvwxyz\"\n        },{\n            \"name\": \"NI.Debug.LED0Bool\",\n            \"description-en\": \"one of 4 blue LEDs with Bool data type\",\n            \"documentation-en\": \"towards back of module, under 2 caps, LED on far right\",\n            \"dataType\": \"Bool\",\n            \"bitfield\": \"DebugLeds/DebugLed0\",\n            \"access\": \"WriteOnly\" \n        },{\n            \"name\": \"NI.Debug.LED1Bool\",\n            \"description-en\": \"one of 4 blue LEDs with Bool data type\",\n            \"documentation-en\": \"towards back of module, under 2 caps, 2nd LED from the right\",\n            \"dataType\": \"Bool\",\n            \"bitfield\": \"DebugLeds/DebugLed1\",\n            \"access\": \"ReadWrite\"\n        },{\n            \"name\": \"NI.Debug.LED2Bool\",\n            \"description-en\": \"one of 4 blue LEDs with Bool data type\",\n            \"documentation-en\": \"towards back of module, under 2 caps, 2nd LED from the left\",\n            \"dataType\": \"Bool\",\n            \"bitfield\": \"DebugLeds/DebugLed2\",\n            \"access\": \"ReadWrite\"\n        },{\n            \"name\": \"NI.Debug.LED3Bool\",\n            \"description-en\": \"one of 4 blue LEDs with Bool data type\",\n            \"documentation-en\": \"towards back of module, under 2 caps, LED on far left\",\n            \"dataType\": \"Bool\",\n            \"bitfield\": \"DebugLeds/DebugLed3\",\n            \"access\": \"ReadWrite\"\n        },{\n            \"name\": \"NI.Debug.LED0Enum\",\n            \"description-en\": \"one of 4 blue LEDs with Enum data type\",\n            \"documentation-en\": \"towards back of module, under 2 caps, LED on far right\",\n            \"dataType\": \"NI.LEDState\",\n            \"bitfield\": \"DebugLeds/DebugLed0\",\n            \"access\": \"WriteOnly\"  \n        },{\n            \"name\": \"NI.Debug.LED1Enum\",\n            \"description-en\": \"one of 4 blue LEDs with Enum data type\",\n            \"documentation-en\": \"towards back of module, under 2 caps, 2nd LED from the right\",\n            \"dataType\": \"NI.LEDState\",\n            \"bitfield\": \"DebugLeds/DebugLed1\",\n            \"access\": \"ReadWrite\"\n        },{\n            \"name\": \"NI.Debug.LED2Enum\",\n            \"description-en\": \"one of 4 blue LEDs with Enum data type\",\n            \"documentation-en\": \"towards back of module, under 2 caps, 2nd LED from the left\",\n            \"dataType\": \"NI.LEDState\",\n            \"bitfield\": \"DebugLeds/DebugLed2\",\n            \"access\": \"ReadWrite\"\n        },{\n            \"name\": \"NI.Debug.LED3Enum\",\n            \"description-en\": \"one of 4 blue LEDs with Enum data type\",\n            \"documentation-en\": \"towards back of module, under 2 caps, LED on far left\",\n            \"dataType\": \"NI.LEDState\",\n            \"bitfield\": \"DebugLeds/DebugLed3\",\n            \"access\": \"ReadWrite\"\n        },{\n            \"name\": \"NI.Scratchpad64.U64\",\n            \"description-en\": \"use 64-bit Scratchpad as U64\",\n            \"documentation-en\": \"Read write 64-bit scratchpad with U64 value\",\n            \"dataType\": \"UInt64\",\n            \"access\": \"ReadWrite\",\n            \"bitfield\": \"DebugScratch64/Scratch64\"\n        },{\n            \"name\": \"NI.Scratchpad64.I64\",\n            \"description-en\": \"use 64-bit Scratchpad as I64\",\n            \"documentation-en\": \"Read write 64-bit scratchpad with I64 value\",\n            \"dataType\": \"Int64\",\n            \"access\": \"ReadWrite\",\n            \"bitfield\": \"DebugScratch64/ScratchI64\"\n        },{\n            \"name\": \"NI.Scratchpad64.U32\",\n            \"description-en\": \"use 64-bit Scratchpad as U32\",\n            \"documentation-en\": \"Read write 64-bit scratchpad with U32 value\",\n            \"dataType\": \"UInt32\",\n            \"access\": \"ReadWrite\",\n            \"bitfield\": \"DebugScratch64/Scratch32\"\n        },{\n            \"name\": \"NI.Scratchpad64.I32\",\n            \"description-en\": \"use 64-bit Scratchpad as I32\",\n            \"documentation-en\": \"Read write 64-bit scratchpad with I32 value\",\n            \"dataType\": \"Int32\",\n            \"access\": \"ReadWrite\",\n            \"bitfield\": \"DebugScratch64/ScratchI32\"\n        },{\n            \"name\": \"NI.Scratchpad64.U16\",\n            \"description-en\": \"use 64-bit Scratchpad as U16\",\n            \"documentation-en\": \"Read write 64-bit scratchpad with U16 value\",\n            \"dataType\": \"UInt32\",\n            \"access\": \"ReadWrite\",\n            \"bitfield\": \"DebugScratch64/Scratch16\"\n        },{\n            \"name\": \"NI.Scratchpad64.I16\",\n            \"description-en\": \"use 64-bit Scratchpad as I16\",\n            \"documentation-en\": \"Read write 64-bit scratchpad with I16 value\",\n            \"dataType\": \"Int32\",\n            \"access\": \"ReadWrite\",\n            \"bitfield\": \"DebugScratch64/ScratchI16\"\n        },{\n            \"name\": \"NI.Scratchpad64.U8\",\n            \"description-en\": \"use 64-bit Scratchpad as U8\",\n            \"documentation-en\": \"Read write 64-bit scratchpad with U8 value\",\n            \"dataType\": \"UInt32\",\n            \"access\": \"ReadWrite\",\n            \"bitfield\": \"DebugScratch64/Scratch8\"\n        },{\n            \"name\": \"NI.Scratchpad64.I8\",\n            \"description-en\": \"use 64-bit Scratchpad as I8\",\n            \"documentation-en\": \"Read write 64-bit scratchpad with I8 value\",\n            \"dataType\": \"Int32\",\n            \"access\": \"ReadWrite\",\n            \"bitfield\": \"DebugScratch64/ScratchI8\"\n        },{\n            \"name\": \"NI.Scratchpad64.Bool\",\n            \"description-en\": \"use 64-bit Scratchpad as Bool\",\n            \"documentation-en\": \"Read write 64-bit scratchpad with Bool value\",\n            \"dataType\": \"Bool\",\n            \"access\": \"ReadWrite\",\n            \"bitfield\": \"DebugScratch64/ScratchBool\"\n        },{\n            \"name\": \"NI.Scratchpad64.Double\",\n            \"description-en\": \"use 64-bit Scratchpad as Double\",\n            \"documentation-en\": \"Read write 64-bit scratchpad with Double value\",\n            \"dataType\": \"Double\",\n            \"access\": \"ReadWrite\",\n            \"bitfield\": \"DebugScratch64/ScratchI64\"\n        },{\n            \"name\": \"NI.Scratchpad32.U32\",\n            \"description-en\": \"use 32-bit Scratchpad as U32\",\n            \"documentation-en\": \"Read write 32-bit scratchpad with U32 value\",\n            \"dataType\": \"UInt32\",\n            \"access\": \"ReadWrite\",\n            \"bitfield\": \"DebugScratch32/Scratch32\"\n        },{\n            \"name\": \"NI.Scratchpad32.I32\",\n            \"description-en\": \"use 32-bit Scratchpad as I32\",\n            \"documentation-en\": \"Read write 32-bit scratchpad with I32 value\",\n            \"dataType\": \"Int32\",\n            \"access\": \"ReadWrite\",\n            \"bitfield\": \"DebugScratch32/ScratchI32\"\n        },{\n            \"name\": \"NI.Scratchpad32.U16\",\n            \"description-en\": \"use 32-bit Scratchpad as U16\",\n            \"documentation-en\": \"Read write 32-bit scratchpad with U16 value\",\n            \"dataType\": \"UInt32\",\n            \"access\": \"ReadWrite\",\n            \"bitfield\": \"DebugScratch32/Scratch16\"\n        },{\n            \"name\": \"NI.Scratchpad32.I16\",\n            \"description-en\": \"use 32-bit Scratchpad as I16\",\n            \"documentation-en\": \"Read write 32-bit scratchpad with I16 value\",\n            \"dataType\": \"Int32\",\n            \"access\": \"ReadWrite\",\n            \"bitfield\": \"DebugScratch32/ScratchI16\"\n        },{\n            \"name\": \"NI.Scratchpad32.U8\",\n            \"description-en\": \"use 32-bit Scratchpad as U8\",\n            \"documentation-en\": \"Read write 32-bit scratchpad with U8 value\",\n            \"dataType\": \"UInt32\",\n            \"access\": \"ReadWrite\",\n            \"bitfield\": \"DebugScratch32/Scratch8\"\n        },{\n            \"name\": \"NI.Scratchpad32.I8\",\n            \"description-en\": \"use 32-bit Scratchpad as I8\",\n            \"documentation-en\": \"Read write 32-bit scratchpad with I8 value\",\n            \"dataType\": \"Int32\",\n            \"access\": \"ReadWrite\",\n            \"bitfield\": \"DebugScratch32/ScratchI8\"\n        },{\n            \"name\": \"NI.Scratchpad32.Bool\",\n            \"description-en\": \"use 32-bit Scratchpad as Bool\",\n            \"documentation-en\": \"Read write 32-bit scratchpad with Bool value\",\n            \"dataType\": \"Bool\",\n            \"access\": \"ReadWrite\",\n            \"bitfield\": \"DebugScratch32/ScratchBool\"\n        },{\n            \"name\": \"NI.Scratchpad32.Double\",\n            \"description-en\": \"use 32-bit Scratchpad as Double\",\n            \"documentation-en\": \"Read write 32-bit scratchpad with Double value\",\n            \"dataType\": \"Double\",\n            \"access\": \"ReadWrite\",\n            \"bitfield\": \"DebugScratch32/ScratchI32\"\n        },{\n            \"name\": \"NI.Scratchpad16.U16\",\n            \"description-en\": \"use 16-bit Scratchpad as U16\",\n            \"documentation-en\": \"Read write 16-bit scratchpad with U16 value\",\n            \"dataType\": \"UInt32\",\n            \"access\": \"ReadWrite\",\n            \"bitfield\": \"DebugScratch16/Scratch16\"\n        },{\n            \"name\": \"NI.Scratchpad16.I16\",\n            \"description-en\": \"use 16-bit Scratchpad as I16\",\n            \"documentation-en\": \"Read write 16-bit scratchpad with I16 value\",\n            \"dataType\": \"Int32\",\n            \"access\": \"ReadWrite\",\n            \"bitfield\": \"DebugScratch16/ScratchI16\"\n        },{\n            \"name\": \"NI.Scratchpad16.U8\",\n            \"description-en\": \"use 16-bit Scratchpad as U8\",\n            \"documentation-en\": \"Read write 16-bit scratchpad with U8 value\",\n            \"dataType\": \"UInt32\",\n            \"access\": \"ReadWrite\",\n            \"bitfield\": \"DebugScratch16/Scratch8\"\n        },{\n            \"name\": \"NI.Scratchpad16.I8\",\n            \"description-en\": \"use 16-bit Scratchpad as I8\",\n            \"documentation-en\": \"Read write 16-bit scratchpad with I8 value\",\n            \"dataType\": \"Int32\",\n            \"access\": \"ReadWrite\",\n            \"bitfield\": \"DebugScratch16/ScratchI8\"\n        },{\n            \"name\": \"NI.Scratchpad16.Bool\",\n            \"description-en\": \"use 16-bit Scratchpad as Bool\",\n            \"documentation-en\": \"Read write 16-bit scratchpad with Bool value\",\n            \"dataType\": \"Bool\",\n            \"access\": \"ReadWrite\",\n            \"bitfield\": \"DebugScratch16/ScratchBool\"\n        },{\n            \"name\": \"NI.Scratchpad16.Double\",\n            \"description-en\": \"use 16-bit Scratchpad as Double\",\n            \"documentation-en\": \"Read write 16-bit scratchpad with Double value\",\n            \"dataType\": \"Double\",\n            \"access\": \"ReadWrite\",\n            \"bitfield\": \"DebugScratch16/ScratchI16\"\n        },{\n            \"name\": \"NI.Scratchpad8.U8\",\n            \"description-en\": \"use 8-bit Scratchpad as U8\",\n            \"documentation-en\": \"Read write 8-bit scratchpad with U8 value\",\n            \"dataType\": \"UInt32\",\n            \"access\": \"ReadWrite\",\n            \"bitfield\": \"DebugScratch8/Scratch8\"\n        },{\n            \"name\": \"NI.Scratchpad8.I8\",\n            \"description-en\": \"use 8-bit Scratchpad as I8\",\n            \"documentation-en\": \"Read write 8-bit scratchpad with I8 value\",\n            \"dataType\": \"Int32\",\n            \"access\": \"ReadWrite\",\n            \"bitfield\": \"DebugScratch8/ScratchI8\"\n        },{\n            \"name\": \"NI.Scratchpad8.Bool\",\n            \"description-en\": \"use 8-bit Scratchpad as Bool\",\n            \"documentation-en\": \"Read write 8-bit scratchpad with Bool value\",\n            \"dataType\": \"Bool\",\n            \"access\": \"ReadWrite\",\n            \"bitfield\": \"DebugScratch8/ScratchBool\"\n        },{\n            \"name\": \"NI.Scratchpad8.Double\",\n            \"description-en\": \"use 8-bit Scratchpad as Double\",\n            \"documentation-en\": \"Read write 8-bit scratchpad with Double value\",\n            \"dataType\": \"Double\",\n            \"access\": \"ReadWrite\",\n            \"bitfield\": \"DebugScratch8/ScratchI8\"\n        },{\n            \"name\": \"NI.Debug.ScratchU32.Min10\",\n            \"dataType\": \"UInt32\",\n            \"access\": \"ReadWrite\",\n            \"bitfield\": \"DebugScratch32/Scratch32\",\n            \"min\": 10\n        },{\n            \"name\": \"NI.Debug.ScratchU32.Max10\",\n            \"dataType\": \"UInt32\",\n            \"access\": \"ReadWrite\",\n            \"bitfield\": \"DebugScratch32/Scratch32\",\n            \"max\": 10\n        },{\n            \"name\": \"NI.Debug.ScratchU32.Min10Max20\",\n            \"dataType\": \"UInt32\",\n            \"access\": \"ReadWrite\",\n            \"bitfield\": \"DebugScratch32/Scratch32\",\n            \"min\": 10,\n            \"max\": 20\n        },{\n            \"name\": \"NI.Debug.ScratchI32.Strict4\",\n            \"dataType\": \"Int32\",\n            \"access\": \"ReadWrite\",\n            \"bitfield\": \"DebugScratch32/ScratchI32\",\n            \"scale\": \"TableStrict4Elements\"\n        },{\n            \"name\": \"NI.Debug.ScratchI32.Strict12\",\n            \"dataType\": \"Int32\",\n            \"access\": \"ReadWrite\",\n            \"bitfield\": \"DebugScratch32/ScratchI32\",\n            \"scale\": \"TableStrict12Elements\",\n            \"min\": -2,\n            \"max\": -1\n        },{\n            \"name\": \"NI.Debug.Scratch64.Int32.TableStrict12Elements\",\n            \"dataType\": \"Int32\",\n            \"access\": \"ReadWrite\",\n            \"bitfield\": \"DebugScratch64/ScratchI32\",\n            \"scale\": \"TableStrict12Elements\"\n        },{\n            \"name\": \"NI.Debug.Scratch64.Int32.TableRound\",\n            \"dataType\": \"Int32\",\n            \"access\": \"ReadWrite\",\n            \"bitfield\": \"DebugScratch64/ScratchI32\",\n            \"scale\": \"TableRound\"\n        },{\n            \"name\": \"NI.Debug.Scratch64.Int32.TableInterpolate\",\n            \"dataType\": \"Int32\",\n            \"access\": \"ReadWrite\",\n            \"bitfield\": \"DebugScratch64/ScratchI32\",\n            \"scale\": \"TableInterpolate\"\n        },{\n            \"name\": \"NI.Debug.Scratch64.Int32.LinearDivideBy8\",\n            \"dataType\": \"Int32\",\n            \"access\": \"ReadWrite\",\n            \"bitfield\": \"DebugScratch64/ScratchI32\",\n            \"scale\": \"LinearDivideBy8\"\n        },{\n            \"name\": \"NI.Debug.Scratch64.Int32.Times2Plus2\",\n            \"dataType\": \"Int32\",\n            \"access\": \"ReadWrite\",\n            \"bitfield\": \"DebugScratch64/ScratchI32\",\n            \"scale\": \"Times2Plus2\"\n        },{\n            \"name\": \"NI.Debug.Scratch64.Int32.PolynomialThermocouple\",\n            \"dataType\": \"Int32\",\n            \"access\": \"ReadWrite\",\n            \"bitfield\": \"DebugScratch64/ScratchI32\",\n            \"scale\": \"PolynomialThermocouple\",\n            \"min\": 0,\n            \"max\": 760\n        },{\n            \"name\": \"NI.Debug.Scratch64.Int32.PolynomialBoundaryConditions\",\n            \"dataType\": \"Int32\",\n            \"access\": \"ReadWrite\",\n            \"bitfield\": \"DebugScratch64/ScratchI32\",\n            \"scale\": \"PolynomialBoundaryConditions\"\n        },{\n            \"name\": \"NI.Debug.Scratch32.Int32.TableStrict12Elements\",\n            \"dataType\": \"Int32\",\n            \"access\": \"ReadWrite\",\n            \"bitfield\": \"DebugScratch32/ScratchI32\",\n            \"scale\": \"TableStrict12Elements\"\n        },{\n            \"name\": \"NI.Debug.Scratch32.Int32.TableRound\",\n            \"dataType\": \"Int32\",\n            \"access\": \"ReadWrite\",\n            \"bitfield\": \"DebugScratch32/ScratchI32\",\n            \"scale\": \"TableRound\"\n        },{\n            \"name\": \"NI.Debug.Scratch32.Int32.TableInterpolate\",\n            \"dataType\": \"Int32\",\n            \"access\": \"ReadWrite\",\n            \"bitfield\": \"DebugScratch32/ScratchI32\",\n            \"scale\": \"TableInterpolate\"\n        },{\n            \"name\": \"NI.Debug.Scratch32.Int32.LinearDivideBy8\",\n            \"dataType\": \"Int32\",\n            \"access\": \"ReadWrite\",\n            \"bitfield\": \"DebugScratch32/ScratchI32\",\n            \"scale\": \"LinearDivideBy8\"\n        },{\n            \"name\": \"NI.Debug.Scratch32.Int32.Times2Plus2\",\n            \"dataType\": \"Int32\",\n            \"access\": \"ReadWrite\",\n            \"bitfield\": \"DebugScratch32/ScratchI32\",\n            \"scale\": \"Times2Plus2\"\n        },{\n            \"name\": \"NI.Debug.Scratch32.Int32.PolynomialThermocouple\",\n            \"dataType\": \"Int32\",\n            \"access\": \"ReadWrite\",\n            \"bitfield\": \"DebugScratch32/ScratchI32\",\n            \"scale\": \"PolynomialThermocouple\",\n            \"min\": 0,\n            \"max\": 760\n        },{\n            \"name\": \"NI.Debug.Scratch32.Int32.PolynomialBoundaryConditions\",\n            \"dataType\": \"Int32\",\n            \"access\": \"ReadWrite\",\n            \"bitfield\": \"DebugScratch32/ScratchI32\",\n            \"scale\": \"PolynomialBoundaryConditions\"\n        },{\n            \"name\": \"NI.Debug.Scratch16.Int32.TableStrict12Elements\",\n            \"dataType\": \"Int32\",\n            \"access\": \"ReadWrite\",\n            \"bitfield\": \"DebugScratch16/ScratchI16\",\n            \"scale\": \"TableStrict12Elements\"\n        },{\n            \"name\": \"NI.Debug.Scratch16.Int32.TableRound\",\n            \"dataType\": \"Int32\",\n            \"access\": \"ReadWrite\",\n            \"bitfield\": \"DebugScratch16/ScratchI16\",\n            \"scale\": \"TableRound\"\n        },{\n            \"name\": \"NI.Debug.Scratch16.Int32.TableInterpolate\",\n            \"dataType\": \"Int32\",\n            \"access\": \"ReadWrite\",\n            \"bitfield\": \"DebugScratch16/ScratchI16\",\n            \"scale\": \"TableInterpolate\"\n        },{\n            \"name\": \"NI.Debug.Scratch16.Int32.LinearDivideBy8\",\n            \"dataType\": \"Int32\",\n            \"access\": \"ReadWrite\",\n            \"bitfield\": \"DebugScratch16/ScratchI16\",\n            \"scale\": \"LinearDivideBy8\"\n        },{\n            \"name\": \"NI.Debug.Scratch16.Int32.Times2Plus2\",\n            \"dataType\": \"Int32\",\n            \"access\": \"ReadWrite\",\n            \"bitfield\": \"DebugScratch16/ScratchI16\",\n            \"scale\": \"Times2Plus2\"\n        },{\n            \"name\": \"NI.Debug.Scratch16.Int32.PolynomialThermocouple\",\n            \"dataType\": \"Int32\",\n            \"access\": \"ReadWrite\",\n            \"bitfield\": \"DebugScratch16/ScratchI16\",\n            \"scale\": \"PolynomialThermocouple\",\n            \"min\": 0,\n            \"max\": 760\n        },{\n            \"name\": \"NI.Debug.Scratch16.Int32.PolynomialBoundaryConditions\",\n            \"dataType\": \"Int32\",\n            \"access\": \"ReadWrite\",\n            \"bitfield\": \"DebugScratch16/ScratchI16\",\n            \"scale\": \"PolynomialBoundaryConditions\"\n        },{\n            \"name\": \"NI.Debug.Scratch8.Int32.TableStrict12Elements\",\n            \"dataType\": \"Int32\",\n            \"access\": \"ReadWrite\",\n            \"bitfield\": \"DebugScratch8/ScratchI8\",\n            \"scale\": \"TableStrict12Elements\"\n        },{\n            \"name\": \"NI.Debug.Scratch8.Int32.TableRound\",\n            \"dataType\": \"Int32\",\n            \"access\": \"ReadWrite\",\n            \"bitfield\": \"DebugScratch8/ScratchI8\",\n            \"scale\": \"TableRound\"\n        },{\n            \"name\": \"NI.Debug.Scratch8.Int32.TableInterpolate\",\n            \"dataType\": \"Int32\",\n            \"access\": \"ReadWrite\",\n            \"bitfield\": \"DebugScratch8/ScratchI8\",\n            \"scale\": \"TableInterpolate\"\n        },{\n            \"name\": \"NI.Debug.Scratch8.Int32.LinearDivideBy8\",\n            \"dataType\": \"Int32\",\n            \"access\": \"ReadWrite\",\n            \"bitfield\": \"DebugScratch8/ScratchI8\",\n            \"scale\": \"LinearDivideBy8\"\n        },{\n            \"name\": \"NI.Debug.Scratch8.Int32.Times2Plus2\",\n            \"dataType\": \"Int32\",\n            \"access\": \"ReadWrite\",\n            \"bitfield\": \"DebugScratch8/ScratchI8\",\n            \"scale\": \"Times2Plus2\"\n        },{\n            \"name\": \"NI.Debug.Scratch8.Int32.PolynomialThermocouple\",\n            \"dataType\": \"Int32\",\n            \"access\": \"ReadWrite\",\n            \"bitfield\": \"DebugScratch8/ScratchI8\",\n            \"scale\": \"PolynomialThermocouple\",\n            \"min\": 0,\n            \"max\": 760\n        },{\n            \"name\": \"NI.Debug.Scratch8.Int32.PolynomialBoundaryConditions\",\n            \"dataType\": \"Int32\",\n            \"access\": \"ReadWrite\",\n            \"bitfield\": \"DebugScratch8/ScratchI8\",\n            \"scale\": \"PolynomialBoundaryConditions\"\n        },{\n            \"name\": \"NI.Debug.Scratch64.UInt32.TableStrict12Elements\",\n            \"dataType\": \"UInt32\",\n            \"access\": \"ReadWrite\",\n            \"bitfield\": \"DebugScratch64/Scratch32\",\n            \"scale\": \"TableStrict12Elements\"\n        },{\n            \"name\": \"NI.Debug.Scratch64.UInt32.TableRound\",\n            \"dataType\": \"UInt32\",\n            \"access\": \"ReadWrite\",\n            \"bitfield\": \"DebugScratch64/Scratch32\",\n            \"scale\": \"TableRound\"\n        },{\n            \"name\": \"NI.Debug.Scratch64.UInt32.TableInterpolate\",\n            \"dataType\": \"UInt32\",\n            \"access\": \"ReadWrite\",\n            \"bitfield\": \"DebugScratch64/Scratch32\",\n            \"scale\": \"TableInterpolate\"\n        },{\n            \"name\": \"NI.Debug.Scratch64.UInt32.LinearDivideBy8\",\n            \"dataType\": \"UInt32\",\n            \"access\": \"ReadWrite\",\n            \"bitfield\": \"DebugScratch64/Scratch32\",\n            \"scale\": \"LinearDivideBy8\"\n        },{\n            \"name\": \"NI.Debug.Scratch64.UInt32.Times2Plus2\",\n            \"dataType\": \"UInt32\",\n            \"access\": \"ReadWrite\",\n            \"bitfield\": \"DebugScratch64/Scratch32\",\n            \"scale\": \"Times2Plus2\"\n        },{\n            \"name\": \"NI.Debug.Scratch64.UInt32.PolynomialThermocouple\",\n            \"dataType\": \"UInt32\",\n            \"access\": \"ReadWrite\",\n            \"bitfield\": \"DebugScratch64/Scratch32\",\n            \"scale\": \"PolynomialThermocouple\",\n            \"min\": 0,\n            \"max\": 760\n        },{\n            \"name\": \"NI.Debug.Scratch64.UInt32.PolynomialBoundaryConditions\",\n            \"dataType\": \"UInt32\",\n            \"access\": \"ReadWrite\",\n            \"bitfield\": \"DebugScratch64/Scratch32\",\n            \"scale\": \"PolynomialBoundaryConditions\"\n        },{\n            \"name\": \"NI.Debug.Scratch32.UInt32.TableStrict12Elements\",\n            \"dataType\": \"UInt32\",\n            \"access\": \"ReadWrite\",\n            \"bitfield\": \"DebugScratch32/Scratch32\",\n            \"scale\": \"TableStrict12Elements\"\n        },{\n            \"name\": \"NI.Debug.Scratch32.UInt32.TableRound\",\n            \"dataType\": \"UInt32\",\n            \"access\": \"ReadWrite\",\n            \"bitfield\": \"DebugScratch32/Scratch32\",\n            \"scale\": \"TableRound\"\n        },{\n            \"name\": \"NI.Debug.Scratch32.UInt32.TableInterpolate\",\n            \"dataType\": \"UInt32\",\n            \"access\": \"ReadWrite\",\n            \"bitfield\": \"DebugScratch32/Scratch32\",\n            \"scale\": \"TableInterpolate\"\n        },{\n            \"name\": \"NI.Debug.Scratch32.UInt32.LinearDivideBy8\",\n            \"dataType\": \"UInt32\",\n            \"access\": \"ReadWrite\",\n            \"bitfield\": \"DebugScratch32/Scratch32\",\n            \"scale\": \"LinearDivideBy8\"\n        },{\n            \"name\": \"NI.Debug.Scratch32.UInt32.Times2Plus2\",\n            \"dataType\": \"UInt32\",\n            \"access\": \"ReadWrite\",\n            \"bitfield\": \"DebugScratch32/Scratch32\",\n            \"scale\": \"Times2Plus2\"\n        },{\n            \"name\": \"NI.Debug.Scratch32.UInt32.PolynomialThermocouple\",\n            \"dataType\": \"UInt32\",\n            \"access\": \"ReadWrite\",\n            \"bitfield\": \"DebugScratch32/Scratch32\",\n            \"scale\": \"PolynomialThermocouple\",\n            \"min\": 0,\n            \"max\": 760\n        },{\n            \"name\": \"NI.Debug.Scratch32.UInt32.PolynomialBoundaryConditions\",\n            \"dataType\": \"UInt32\",\n            \"access\": \"ReadWrite\",\n            \"bitfield\": \"DebugScratch32/Scratch32\",\n            \"scale\": \"PolynomialBoundaryConditions\"\n        },{\n            \"name\": \"NI.Debug.Scratch16.UInt32.TableStrict12Elements\",\n            \"dataType\": \"UInt32\",\n            \"access\": \"ReadWrite\",\n            \"bitfield\": \"DebugScratch16/Scratch16\",\n            \"scale\": \"TableStrict12Elements\"\n        },{\n            \"name\": \"NI.Debug.Scratch16.UInt32.TableRound\",\n            \"dataType\": \"UInt32\",\n            \"access\": \"ReadWrite\",\n            \"bitfield\": \"DebugScratch16/Scratch16\",\n            \"scale\": \"TableRound\"\n        },{\n            \"name\": \"NI.Debug.Scratch16.UInt32.TableInterpolate\",\n            \"dataType\": \"UInt32\",\n            \"access\": \"ReadWrite\",\n            \"bitfield\": \"DebugScratch16/Scratch16\",\n            \"scale\": \"TableInterpolate\"\n        },{\n            \"name\": \"NI.Debug.Scratch16.UInt32.LinearDivideBy8\",\n            \"dataType\": \"UInt32\",\n            \"access\": \"ReadWrite\",\n            \"bitfield\": \"DebugScratch16/Scratch16\",\n            \"scale\": \"LinearDivideBy8\"\n        },{\n            \"name\": \"NI.Debug.Scratch16.UInt32.Times2Plus2\",\n            \"dataType\": \"UInt32\",\n            \"access\": \"ReadWrite\",\n            \"bitfield\": \"DebugScratch16/Scratch16\",\n            \"scale\": \"Times2Plus2\"\n        },{\n            \"name\": \"NI.Debug.Scratch16.UInt32.PolynomialThermocouple\",\n            \"dataType\": \"UInt32\",\n            \"access\": \"ReadWrite\",\n            \"bitfield\": \"DebugScratch16/Scratch16\",\n            \"scale\": \"PolynomialThermocouple\",\n            \"min\": 0,\n            \"max\": 760\n        },{\n            \"name\": \"NI.Debug.Scratch16.UInt32.PolynomialBoundaryConditions\",\n            \"dataType\": \"UInt32\",\n            \"access\": \"ReadWrite\",\n            \"bitfield\": \"DebugScratch16/Scratch16\",\n            \"scale\": \"PolynomialBoundaryConditions\"\n        },{\n            \"name\": \"NI.Debug.Scratch8.UInt32.TableStrict12Elements\",\n            \"dataType\": \"UInt32\",\n            \"access\": \"ReadWrite\",\n            \"bitfield\": \"DebugScratch8/Scratch8\",\n            \"scale\": \"TableStrict12Elements\"\n        },{\n            \"name\": \"NI.Debug.Scratch8.UInt32.TableRound\",\n            \"dataType\": \"UInt32\",\n            \"access\": \"ReadWrite\",\n            \"bitfield\": \"DebugScratch8/Scratch8\",\n            \"scale\": \"TableRound\"\n        },{\n            \"name\": \"NI.Debug.Scratch8.UInt32.TableInterpolate\",\n            \"dataType\": \"UInt32\",\n            \"access\": \"ReadWrite\",\n            \"bitfield\": \"DebugScratch8/Scratch8\",\n            \"scale\": \"TableInterpolate\"\n        },{\n            \"name\": \"NI.Debug.Scratch8.UInt32.LinearDivideBy8\",\n            \"dataType\": \"UInt32\",\n            \"access\": \"ReadWrite\",\n            \"bitfield\": \"DebugScratch8/Scratch8\",\n            \"scale\": \"LinearDivideBy8\"\n        },{\n            \"name\": \"NI.Debug.Scratch8.UInt32.Times2Plus2\",\n            \"dataType\": \"UInt32\",\n            \"access\": \"ReadWrite\",\n            \"bitfield\": \"DebugScratch8/Scratch8\",\n            \"scale\": \"Times2Plus2\"\n        },{\n            \"name\": \"NI.Debug.Scratch8.UInt32.PolynomialThermocouple\",\n            \"dataType\": \"UInt32\",\n            \"access\": \"ReadWrite\",\n            \"bitfield\": \"DebugScratch8/Scratch8\",\n            \"scale\": \"PolynomialThermocouple\",\n            \"min\": 0,\n            \"max\": 760\n        },{\n            \"name\": \"NI.Debug.Scratch8.UInt32.PolynomialBoundaryConditions\",\n            \"dataType\": \"UInt32\",\n            \"access\": \"ReadWrite\",\n            \"bitfield\": \"DebugScratch8/Scratch8\",\n            \"scale\": \"PolynomialBoundaryConditions\"\n        },{\n            \"name\": \"NI.Debug.Scratch64.Int64.TableStrict12Elements\",\n            \"dataType\": \"Int64\",\n            \"access\": \"ReadWrite\",\n            \"bitfield\": \"DebugScratch64/ScratchI64\",\n            \"scale\": \"TableStrict12Elements\"\n        },{\n            \"name\": \"NI.Debug.Scratch64.Int64.TableRound\",\n            \"dataType\": \"Int64\",\n            \"access\": \"ReadWrite\",\n            \"bitfield\": \"DebugScratch64/ScratchI64\",\n            \"scale\": \"TableRound\"\n        },{\n            \"name\": \"NI.Debug.Scratch64.Int64.TableInterpolate\",\n            \"dataType\": \"Int64\",\n            \"access\": \"ReadWrite\",\n            \"bitfield\": \"DebugScratch64/ScratchI64\",\n            \"scale\": \"TableInterpolate\"\n        },{\n            \"name\": \"NI.Debug.Scratch64.Int64.LinearDivideBy8\",\n            \"dataType\": \"Int64\",\n            \"access\": \"ReadWrite\",\n            \"bitfield\": \"DebugScratch64/ScratchI64\",\n            \"scale\": \"LinearDivideBy8\"\n        },{\n            \"name\": \"NI.Debug.Scratch64.Int64.Times2Plus2\",\n            \"dataType\": \"Int64\",\n            \"access\": \"ReadWrite\",\n            \"bitfield\": \"DebugScratch64/ScratchI64\",\n            \"scale\": \"Times2Plus2\"\n        },{\n            \"name\": \"NI.Debug.Scratch64.Int64.PolynomialThermocouple\",\n            \"dataType\": \"Int64\",\n            \"access\": \"ReadWrite\",\n            \"bitfield\": \"DebugScratch64/ScratchI64\",\n            \"scale\": \"PolynomialThermocouple\",\n            \"min\": 0,\n            \"max\": 760\n        },{\n            \"name\": \"NI.Debug.Scratch64.Int64.PolynomialBoundaryConditions\",\n            \"dataType\": \"Int64\",\n            \"access\": \"ReadWrite\",\n            \"bitfield\": \"DebugScratch64/ScratchI64\",\n            \"scale\": \"PolynomialBoundaryConditions\"\n        },{\n            \"name\": \"NI.Debug.Scratch32.Int64.TableStrict12Elements\",\n            \"dataType\": \"Int64\",\n            \"access\": \"ReadWrite\",\n            \"bitfield\": \"DebugScratch32/ScratchI32\",\n            \"scale\": \"TableStrict12Elements\"\n        },{\n            \"name\": \"NI.Debug.Scratch32.Int64.TableRound\",\n            \"dataType\": \"Int64\",\n            \"access\": \"ReadWrite\",\n            \"bitfield\": \"DebugScratch32/ScratchI32\",\n            \"scale\": \"TableRound\"\n        },{\n            \"name\": \"NI.Debug.Scratch32.Int64.TableInterpolate\",\n            \"dataType\": \"Int64\",\n            \"access\": \"ReadWrite\",\n            \"bitfield\": \"DebugScratch32/ScratchI32\",\n            \"scale\": \"TableInterpolate\"\n        },{\n            \"name\": \"NI.Debug.Scratch32.Int64.LinearDivideBy8\",\n            \"dataType\": \"Int64\",\n            \"access\": \"ReadWrite\",\n            \"bitfield\": \"DebugScratch32/ScratchI32\",\n            \"scale\": \"LinearDivideBy8\"\n        },{\n            \"name\": \"NI.Debug.Scratch32.Int64.Times2Plus2\",\n            \"dataType\": \"Int64\",\n            \"access\": \"ReadWrite\",\n            \"bitfield\": \"DebugScratch32/ScratchI32\",\n            \"scale\": \"Times2Plus2\"\n        },{\n            \"name\": \"NI.Debug.Scratch32.Int64.PolynomialThermocouple\",\n            \"dataType\": \"Int64\",\n            \"access\": \"ReadWrite\",\n            \"bitfield\": \"DebugScratch32/ScratchI32\",\n            \"scale\": \"PolynomialThermocouple\",\n            \"min\": 0,\n            \"max\": 760\n        },{\n            \"name\": \"NI.Debug.Scratch32.Int64.PolynomialBoundaryConditions\",\n            \"dataType\": \"Int64\",\n            \"access\": \"ReadWrite\",\n            \"bitfield\": \"DebugScratch32/ScratchI32\",\n            \"scale\": \"PolynomialBoundaryConditions\"\n        },{\n            \"name\": \"NI.Debug.Scratch16.Int64.TableStrict12Elements\",\n            \"dataType\": \"Int64\",\n            \"access\": \"ReadWrite\",\n            \"bitfield\": \"DebugScratch16/ScratchI16\",\n            \"scale\": \"TableStrict12Elements\"\n        },{\n            \"name\": \"NI.Debug.Scratch16.Int64.TableRound\",\n            \"dataType\": \"Int64\",\n            \"access\": \"ReadWrite\",\n            \"bitfield\": \"DebugScratch16/ScratchI16\",\n            \"scale\": \"TableRound\"\n        },{\n            \"name\": \"NI.Debug.Scratch16.Int64.TableInterpolate\",\n            \"dataType\": \"Int64\",\n            \"access\": \"ReadWrite\",\n            \"bitfield\": \"DebugScratch16/ScratchI16\",\n            \"scale\": \"TableInterpolate\"\n        },{\n            \"name\": \"NI.Debug.Scratch16.Int64.LinearDivideBy8\",\n            \"dataType\": \"Int64\",\n            \"access\": \"ReadWrite\",\n            \"bitfield\": \"DebugScratch16/ScratchI16\",\n            \"scale\": \"LinearDivideBy8\"\n        },{\n            \"name\": \"NI.Debug.Scratch16.Int64.Times2Plus2\",\n            \"dataType\": \"Int64\",\n            \"access\": \"ReadWrite\",\n            \"bitfield\": \"DebugScratch16/ScratchI16\",\n            \"scale\": \"Times2Plus2\"\n        },{\n            \"name\": \"NI.Debug.Scratch16.Int64.PolynomialThermocouple\",\n            \"dataType\": \"Int64\",\n            \"access\": \"ReadWrite\",\n            \"bitfield\": \"DebugScratch16/ScratchI16\",\n            \"scale\": \"PolynomialThermocouple\",\n            \"min\": 0,\n            \"max\": 760\n        },{\n            \"name\": \"NI.Debug.Scratch16.Int64.PolynomialBoundaryConditions\",\n            \"dataType\": \"Int64\",\n            \"access\": \"ReadWrite\",\n            \"bitfield\": \"DebugScratch16/ScratchI16\",\n            \"scale\": \"PolynomialBoundaryConditions\"\n        },{\n            \"name\": \"NI.Debug.Scratch8.Int64.TableStrict12Elements\",\n            \"dataType\": \"Int64\",\n            \"access\": \"ReadWrite\",\n            \"bitfield\": \"DebugScratch8/ScratchI8\",\n            \"scale\": \"TableStrict12Elements\"\n        },{\n            \"name\": \"NI.Debug.Scratch8.Int64.TableRound\",\n            \"dataType\": \"Int64\",\n            \"access\": \"ReadWrite\",\n            \"bitfield\": \"DebugScratch8/ScratchI8\",\n            \"scale\": \"TableRound\"\n        },{\n            \"name\": \"NI.Debug.Scratch8.Int64.TableInterpolate\",\n            \"dataType\": \"Int64\",\n            \"access\": \"ReadWrite\",\n            \"bitfield\": \"DebugScratch8/ScratchI8\",\n            \"scale\": \"TableInterpolate\"\n        },{\n            \"name\": \"NI.Debug.Scratch8.Int64.LinearDivideBy8\",\n            \"dataType\": \"Int64\",\n            \"access\": \"ReadWrite\",\n            \"bitfield\": \"DebugScratch8/ScratchI8\",\n            \"scale\": \"LinearDivideBy8\"\n        },{\n            \"name\": \"NI.Debug.Scratch8.Int64.Times2Plus2\",\n            \"dataType\": \"Int64\",\n            \"access\": \"ReadWrite\",\n            \"bitfield\": \"DebugScratch8/ScratchI8\",\n            \"scale\": \"Times2Plus2\"\n        },{\n            \"name\": \"NI.Debug.Scratch8.Int64.PolynomialThermocouple\",\n            \"dataType\": \"Int64\",\n            \"access\": \"ReadWrite\",\n            \"bitfield\": \"DebugScratch8/ScratchI8\",\n            \"scale\": \"PolynomialThermocouple\",\n            \"min\": 0,\n            \"max\": 760\n        },{\n            \"name\": \"NI.Debug.Scratch8.Int64.PolynomialBoundaryConditions\",\n            \"dataType\": \"Int64\",\n            \"access\": \"ReadWrite\",\n            \"bitfield\": \"DebugScratch8/ScratchI8\",\n            \"scale\": \"PolynomialBoundaryConditions\"\n        },{\n            \"name\": \"NI.Debug.Scratch64.UInt64.TableStrict12Elements\",\n            \"dataType\": \"UInt64\",\n            \"access\": \"ReadWrite\",\n            \"bitfield\": \"DebugScratch64/Scratch64\",\n            \"scale\": \"TableStrict12Elements\"\n        },{\n            \"name\": \"NI.Debug.Scratch64.UInt64.TableRound\",\n            \"dataType\": \"UInt64\",\n            \"access\": \"ReadWrite\",\n            \"bitfield\": \"DebugScratch64/Scratch64\",\n            \"scale\": \"TableRound\"\n        },{\n            \"name\": \"NI.Debug.Scratch64.UInt64.TableInterpolate\",\n            \"dataType\": \"UInt64\",\n            \"access\": \"ReadWrite\",\n            \"bitfield\": \"DebugScratch64/Scratch64\",\n            \"scale\": \"TableInterpolate\"\n        },{\n            \"name\": \"NI.Debug.Scratch64.UInt64.LinearDivideBy8\",\n            \"dataType\": \"UInt64\",\n            \"access\": \"ReadWrite\",\n            \"bitfield\": \"DebugScratch64/Scratch64\",\n            \"scale\": \"LinearDivideBy8\"\n        },{\n            \"name\": \"NI.Debug.Scratch64.UInt64.Times2Plus2\",\n            \"dataType\": \"UInt64\",\n            \"access\": \"ReadWrite\",\n            \"bitfield\": \"DebugScratch64/Scratch64\",\n            \"scale\": \"Times2Plus2\"\n        },{\n            \"name\": \"NI.Debug.Scratch64.UInt64.PolynomialThermocouple\",\n            \"dataType\": \"UInt64\",\n            \"access\": \"ReadWrite\",\n            \"bitfield\": \"DebugScratch64/Scratch64\",\n            \"scale\": \"PolynomialThermocouple\",\n            \"min\": 0,\n            \"max\": 760\n        },{\n            \"name\": \"NI.Debug.Scratch64.UInt64.PolynomialBoundaryConditions\",\n            \"dataType\": \"UInt64\",\n            \"access\": \"ReadWrite\",\n            \"bitfield\": \"DebugScratch64/Scratch64\",\n            \"scale\": \"PolynomialBoundaryConditions\"\n        },{\n            \"name\": \"NI.Debug.Scratch32.UInt64.TableStrict12Elements\",\n            \"dataType\": \"UInt64\",\n            \"access\": \"ReadWrite\",\n            \"bitfield\": \"DebugScratch32/Scratch32\",\n            \"scale\": \"TableStrict12Elements\"\n        },{\n            \"name\": \"NI.Debug.Scratch32.UInt64.TableRound\",\n            \"dataType\": \"UInt64\",\n            \"access\": \"ReadWrite\",\n            \"bitfield\": \"DebugScratch32/Scratch32\",\n            \"scale\": \"TableRound\"\n        },{\n            \"name\": \"NI.Debug.Scratch32.UInt64.TableInterpolate\",\n            \"dataType\": \"UInt64\",\n            \"access\": \"ReadWrite\",\n            \"bitfield\": \"DebugScratch32/Scratch32\",\n            \"scale\": \"TableInterpolate\"\n        },{\n            \"name\": \"NI.Debug.Scratch32.UInt64.LinearDivideBy8\",\n            \"dataType\": \"UInt64\",\n            \"access\": \"ReadWrite\",\n            \"bitfield\": \"DebugScratch32/Scratch32\",\n            \"scale\": \"LinearDivideBy8\"\n        },{\n            \"name\": \"NI.Debug.Scratch32.UInt64.Times2Plus2\",\n            \"dataType\": \"UInt64\",\n            \"access\": \"ReadWrite\",\n            \"bitfield\": \"DebugScratch32/Scratch32\",\n            \"scale\": \"Times2Plus2\"\n        },{\n            \"name\": \"NI.Debug.Scratch32.UInt64.PolynomialThermocouple\",\n            \"dataType\": \"UInt64\",\n            \"access\": \"ReadWrite\",\n            \"bitfield\": \"DebugScratch32/Scratch32\",\n            \"scale\": \"PolynomialThermocouple\",\n            \"min\": 0,\n            \"max\": 760\n        },{\n            \"name\": \"NI.Debug.Scratch32.UInt64.PolynomialBoundaryConditions\",\n            \"dataType\": \"UInt64\",\n            \"access\": \"ReadWrite\",\n            \"bitfield\": \"DebugScratch32/Scratch32\",\n            \"scale\": \"PolynomialBoundaryConditions\"\n        },{\n            \"name\": \"NI.Debug.Scratch16.UInt64.TableStrict12Elements\",\n            \"dataType\": \"UInt64\",\n            \"access\": \"ReadWrite\",\n            \"bitfield\": \"DebugScratch16/Scratch16\",\n            \"scale\": \"TableStrict12Elements\"\n        },{\n            \"name\": \"NI.Debug.Scratch16.UInt64.TableRound\",\n            \"dataType\": \"UInt64\",\n            \"access\": \"ReadWrite\",\n            \"bitfield\": \"DebugScratch16/Scratch16\",\n            \"scale\": \"TableRound\"\n        },{\n            \"name\": \"NI.Debug.Scratch16.UInt64.TableInterpolate\",\n            \"dataType\": \"UInt64\",\n            \"access\": \"ReadWrite\",\n            \"bitfield\": \"DebugScratch16/Scratch16\",\n            \"scale\": \"TableInterpolate\"\n        },{\n            \"name\": \"NI.Debug.Scratch16.UInt64.LinearDivideBy8\",\n            \"dataType\": \"UInt64\",\n            \"access\": \"ReadWrite\",\n            \"bitfield\": \"DebugScratch16/Scratch16\",\n            \"scale\": \"LinearDivideBy8\"\n        },{\n            \"name\": \"NI.Debug.Scratch16.UInt64.Times2Plus2\",\n            \"dataType\": \"UInt64\",\n            \"access\": \"ReadWrite\",\n            \"bitfield\": \"DebugScratch16/Scratch16\",\n            \"scale\": \"Times2Plus2\"\n        },{\n            \"name\": \"NI.Debug.Scratch16.UInt64.PolynomialThermocouple\",\n            \"dataType\": \"UInt64\",\n            \"access\": \"ReadWrite\",\n            \"bitfield\": \"DebugScratch16/Scratch16\",\n            \"scale\": \"PolynomialThermocouple\",\n            \"min\": 0,\n            \"max\": 760\n        },{\n            \"name\": \"NI.Debug.Scratch16.UInt64.PolynomialBoundaryConditions\",\n            \"dataType\": \"UInt64\",\n            \"access\": \"ReadWrite\",\n            \"bitfield\": \"DebugScratch16/Scratch16\",\n            \"scale\": \"PolynomialBoundaryConditions\"\n        },{\n            \"name\": \"NI.Debug.Scratch8.UInt64.TableStrict12Elements\",\n            \"dataType\": \"UInt64\",\n            \"access\": \"ReadWrite\",\n            \"bitfield\": \"DebugScratch8/Scratch8\",\n            \"scale\": \"TableStrict12Elements\"\n        },{\n            \"name\": \"NI.Debug.Scratch8.UInt64.TableRound\",\n            \"dataType\": \"UInt64\",\n            \"access\": \"ReadWrite\",\n            \"bitfield\": \"DebugScratch8/Scratch8\",\n            \"scale\": \"TableRound\"\n        },{\n            \"name\": \"NI.Debug.Scratch8.UInt64.TableInterpolate\",\n            \"dataType\": \"UInt64\",\n            \"access\": \"ReadWrite\",\n            \"bitfield\": \"DebugScratch8/Scratch8\",\n            \"scale\": \"TableInterpolate\"\n        },{\n            \"name\": \"NI.Debug.Scratch8.UInt64.LinearDivideBy8\",\n            \"dataType\": \"UInt64\",\n            \"access\": \"ReadWrite\",\n            \"bitfield\": \"DebugScratch8/Scratch8\",\n            \"scale\": \"LinearDivideBy8\"\n        },{\n            \"name\": \"NI.Debug.Scratch8.UInt64.Times2Plus2\",\n            \"dataType\": \"UInt64\",\n            \"access\": \"ReadWrite\",\n            \"bitfield\": \"DebugScratch8/Scratch8\",\n            \"scale\": \"Times2Plus2\"\n        },{\n            \"name\": \"NI.Debug.Scratch8.UInt64.PolynomialThermocouple\",\n            \"dataType\": \"UInt64\",\n            \"access\": \"ReadWrite\",\n            \"bitfield\": \"DebugScratch8/Scratch8\",\n            \"scale\": \"PolynomialThermocouple\",\n            \"min\": 0,\n            \"max\": 760\n        },{\n            \"name\": \"NI.Debug.Scratch8.UInt64.PolynomialBoundaryConditions\",\n            \"dataType\": \"UInt64\",\n            \"access\": \"ReadWrite\",\n            \"bitfield\": \"DebugScratch8/Scratch8\",\n            \"scale\": \"PolynomialBoundaryConditions\"\n        },{\n            \"name\": \"NI.Debug.Scratch64.Double.TableStrict\",\n            \"dataType\": \"Double\",\n            \"access\": \"ReadWrite\",\n            \"bitfield\": \"DebugScratch64/ScratchI64\",\n            \"scale\": \"TableStrict\"\n        },{\n            \"name\": \"NI.Debug.Scratch64.Double.TableStrict12Elements\",\n            \"dataType\": \"Double\",\n            \"access\": \"ReadWrite\",\n            \"bitfield\": \"DebugScratch64/ScratchI64\",\n            \"scale\": \"TableStrict12Elements\"\n        },{\n            \"name\": \"NI.Debug.Scratch64.Double.TableRound\",\n            \"dataType\": \"Double\",\n            \"access\": \"ReadWrite\",\n            \"bitfield\": \"DebugScratch64/ScratchI64\",\n            \"scale\": \"TableRound\"\n        },{\n            \"name\": \"NI.Debug.Scratch64.Double.TableInterpolate\",\n            \"dataType\": \"Double\",\n            \"access\": \"ReadWrite\",\n            \"bitfield\": \"DebugScratch64/ScratchI64\",\n            \"scale\": \"TableInterpolate\"\n        },{\n            \"name\": \"NI.Debug.Scratch64.Double.LinearDivideBy8\",\n            \"dataType\": \"Double\",\n            \"access\": \"ReadWrite\",\n            \"bitfield\": \"DebugScratch64/ScratchI64\",\n            \"scale\": \"LinearDivideBy8\"\n        },{\n            \"name\": \"NI.Debug.Scratch64.Double.Times2Plus2\",\n            \"dataType\": \"Double\",\n            \"access\": \"ReadWrite\",\n            \"bitfield\": \"DebugScratch64/ScratchI64\",\n            \"scale\": \"Times2Plus2\"\n        },{\n            \"name\": \"NI.Debug.Scratch64.Double.PolynomialThermocouple\",\n            \"dataType\": \"Double\",\n            \"access\": \"ReadWrite\",\n            \"bitfield\": \"DebugScratch64/ScratchI64\",\n            \"scale\": \"PolynomialThermocouple\",\n            \"min\": 0,\n            \"max\": 760\n        },{\n            \"name\": \"NI.Debug.Scratch64.Double.PolynomialBoundaryConditions\",\n            \"dataType\": \"Double\",\n            \"access\": \"ReadWrite\",\n            \"bitfield\": \"DebugScratch64/ScratchI64\",\n            \"scale\": \"PolynomialBoundaryConditions\"\n        },{\n            \"name\": \"NI.Debug.Scratch32.Double.TableStrict\",\n            \"dataType\": \"Double\",\n            \"access\": \"ReadWrite\",\n            \"bitfield\": \"DebugScratch32/ScratchI32\",\n            \"scale\": \"TableStrict\"\n        },{\n            \"name\": \"NI.Debug.Scratch32.Double.TableStrict12Elements\",\n            \"dataType\": \"Double\",\n            \"access\": \"ReadWrite\",\n            \"bitfield\": \"DebugScratch32/ScratchI32\",\n            \"scale\": \"TableStrict12Elements\"\n        },{\n            \"name\": \"NI.Debug.Scratch32.Double.TableRound\",\n            \"dataType\": \"Double\",\n            \"access\": \"ReadWrite\",\n            \"bitfield\": \"DebugScratch32/ScratchI32\",\n            \"scale\": \"TableRound\"\n        },{\n            \"name\": \"NI.Debug.Scratch32.Double.TableInterpolate\",\n            \"dataType\": \"Double\",\n            \"access\": \"ReadWrite\",\n            \"bitfield\": \"DebugScratch32/ScratchI32\",\n            \"scale\": \"TableInterpolate\"\n        },{\n            \"name\": \"NI.Debug.Scratch32.Double.LinearDivideBy8\",\n            \"dataType\": \"Double\",\n            \"access\": \"ReadWrite\",\n            \"bitfield\": \"DebugScratch32/ScratchI32\",\n            \"scale\": \"LinearDivideBy8\"\n        },{\n            \"name\": \"NI.Debug.Scratch32.Double.Times2Plus2\",\n            \"dataType\": \"Double\",\n            \"access\": \"ReadWrite\",\n            \"bitfield\": \"DebugScratch32/ScratchI32\",\n            \"scale\": \"Times2Plus2\"\n        },{\n            \"name\": \"NI.Debug.Scratch32.Double.PolynomialThermocouple\",\n            \"dataType\": \"Double\",\n            \"access\": \"ReadWrite\",\n            \"bitfield\": \"DebugScratch32/ScratchI32\",\n            \"scale\": \"PolynomialThermocouple\",\n            \"min\": 0,\n            \"max\": 760\n        },{\n            \"name\": \"NI.Debug.Scratch32.Double.PolynomialBoundaryConditions\",\n            \"dataType\": \"Double\",\n            \"access\": \"ReadWrite\",\n            \"bitfield\": \"DebugScratch32/ScratchI32\",\n            \"scale\": \"PolynomialBoundaryConditions\"\n        },{\n            \"name\": \"NI.Debug.Scratch16.Double.TableStrict\",\n            \"dataType\": \"Double\",\n            \"access\": \"ReadWrite\",\n            \"bitfield\": \"DebugScratch16/ScratchI16\",\n            \"scale\": \"TableStrict\"\n        },{\n            \"name\": \"NI.Debug.Scratch16.Double.TableStrict12Elements\",\n            \"dataType\": \"Double\",\n            \"access\": \"ReadWrite\",\n            \"bitfield\": \"DebugScratch16/ScratchI16\",\n            \"scale\": \"TableStrict12Elements\"\n        },{\n            \"name\": \"NI.Debug.Scratch16.Double.TableRound\",\n            \"dataType\": \"Double\",\n            \"access\": \"ReadWrite\",\n            \"bitfield\": \"DebugScratch16/ScratchI16\",\n            \"scale\": \"TableRound\"\n        },{\n            \"name\": \"NI.Debug.Scratch16.Double.TableInterpolate\",\n            \"dataType\": \"Double\",\n            \"access\": \"ReadWrite\",\n            \"bitfield\": \"DebugScratch16/ScratchI16\",\n            \"scale\": \"TableInterpolate\"\n        },{\n            \"name\": \"NI.Debug.Scratch16.Double.LinearDivideBy8\",\n            \"dataType\": \"Double\",\n            \"access\": \"ReadWrite\",\n            \"bitfield\": \"DebugScratch16/ScratchI16\",\n            \"scale\": \"LinearDivideBy8\"\n        },{\n            \"name\": \"NI.Debug.Scratch16.Double.Times2Plus2\",\n            \"dataType\": \"Double\",\n            \"access\": \"ReadWrite\",\n            \"bitfield\": \"DebugScratch16/ScratchI16\",\n            \"scale\": \"Times2Plus2\"\n        },{\n            \"name\": \"NI.Debug.Scratch16.Double.PolynomialThermocouple\",\n            \"dataType\": \"Double\",\n            \"access\": \"ReadWrite\",\n            \"bitfield\": \"DebugScratch16/ScratchI16\",\n            \"scale\": \"PolynomialThermocouple\",\n            \"min\": 0,\n            \"max\": 760\n        },{\n            \"name\": \"NI.Debug.Scratch16.Double.PolynomialBoundaryConditions\",\n            \"dataType\": \"Double\",\n            \"access\": \"ReadWrite\",\n            \"bitfield\": \"DebugScratch16/ScratchI16\",\n            \"scale\": \"PolynomialBoundaryConditions\"\n        },{\n            \"name\": \"NI.Debug.Scratch8.Double.TableStrict\",\n            \"dataType\": \"Double\",\n            \"access\": \"ReadWrite\",\n            \"bitfield\": \"DebugScratch8/ScratchI8\",\n            \"scale\": \"TableStrict\"\n        },{\n            \"name\": \"NI.Debug.Scratch8.Double.TableStrict12Elements\",\n            \"dataType\": \"Double\",\n            \"access\": \"ReadWrite\",\n            \"bitfield\": \"DebugScratch8/ScratchI8\",\n            \"scale\": \"TableStrict12Elements\"\n        },{\n            \"name\": \"NI.Debug.Scratch8.Double.TableRound\",\n            \"dataType\": \"Double\",\n            \"access\": \"ReadWrite\",\n            \"bitfield\": \"DebugScratch8/ScratchI8\",\n            \"scale\": \"TableRound\"\n        },{\n            \"name\": \"NI.Debug.Scratch8.Double.TableInterpolate\",\n            \"dataType\": \"Double\",\n            \"access\": \"ReadWrite\",\n            \"bitfield\": \"DebugScratch8/ScratchI8\",\n            \"scale\": \"TableInterpolate\"\n        },{\n            \"name\": \"NI.Debug.Scratch8.Double.LinearDivideBy8\",\n            \"dataType\": \"Double\",\n            \"access\": \"ReadWrite\",\n            \"bitfield\": \"DebugScratch8/ScratchI8\",\n            \"scale\": \"LinearDivideBy8\"\n        },{\n            \"name\": \"NI.Debug.Scratch8.Double.Times2Plus2\",\n            \"dataType\": \"Double\",\n            \"access\": \"ReadWrite\",\n            \"bitfield\": \"DebugScratch8/ScratchI8\",\n            \"scale\": \"Times2Plus2\"\n        },{\n            \"name\": \"NI.Debug.Scratch8.Double.PolynomialThermocouple\",\n            \"dataType\": \"Double\",\n            \"access\": \"ReadWrite\",\n            \"bitfield\": \"DebugScratch8/ScratchI8\",\n            \"scale\": \"PolynomialThermocouple\",\n            \"min\": 0,\n            \"max\": 760\n        },{\n            \"name\": \"NI.Debug.Scratch8.Double.PolynomialBoundaryConditions\",\n            \"dataType\": \"Double\",\n            \"access\": \"ReadWrite\",\n            \"bitfield\": \"DebugScratch8/ScratchI8\",\n            \"scale\": \"PolynomialBoundaryConditions\"\n        },{\n            \"name\": \"NI.Debug.ScratchBool.InvertBoolean\",\n            \"dataType\": \"Bool\",\n            \"access\": \"ReadWrite\",\n            \"bitfield\": \"DebugScratch64/ScratchBool\",\n            \"scale\": \"InvertBoolean\"\n        },{\n            \"name\": \"NI.Debug.ScratchBool.TableStrictTrueFalse\",\n            \"dataType\": \"Bool\",\n            \"access\": \"ReadWrite\",\n            \"bitfield\": \"DebugScratch64/Scratch64\",\n            \"scale\": \"TableStrictTrueFalse\"\n        },{\n            \"name\": \"NI.Debug.ScratchBool.TableStrictFalse\",\n            \"dataType\": \"Bool\",\n            \"access\": \"ReadWrite\",\n            \"bitfield\": \"DebugScratch64/Scratch64\",\n            \"scale\": \"TableStrictFalse\"\n        },{\n            \"name\": \"NI.Debug.ScratchBool.TableStrictTrue\",\n            \"dataType\": \"Bool\",\n            \"access\": \"ReadWrite\",\n            \"bitfield\": \"DebugScratch64/Scratch64\",\n            \"scale\": \"TableStrictTrue\"\n        },{\n            \"name\": \"NI.GreenLED0\",\n            \"description-en\": \"one of 3 tri-colored LEDs (red/green/amber), controls green\",\n            \"documentation-en\": \"towards front of module, at the top, left LED\",\n            \"dataType\": \"Bool\",\n            \"access\": \"WriteOnly\",\n            \"bitfield\": \"FrontPanelLeds/LedGreen0Enable\"\n        },{\n            \"name\": \"NI.GreenLED1\",\n            \"description-en\": \"one of 3 tri-colored LEDs (red/green/amber), controls green\",\n            \"documentation-en\": \"towards front of module, at the top, center LED\",\n            \"dataType\": \"Bool\",\n            \"access\": \"WriteOnly\",\n            \"bitfield\": \"FrontPanelLeds/LedGreen1Enable\"\n        },{\n            \"name\": \"NI.GreenLED2\",\n            \"description-en\": \"one of 3 tri-colored LEDs (red/green/amber), controls green\",\n            \"documentation-en\": \"towards front of module, at the top, right LED\",\n            \"dataType\": \"Bool\",\n            \"access\": \"WriteOnly\",\n            \"bitfield\": \"FrontPanelLeds/LedGreen2Enable\"\n        },{\n            \"name\": \"NI.RedLED0\",\n            \"description-en\": \"one of 3 tri-colored LEDs (red/green/amber), controls red\",\n            \"documentation-en\": \"towards front of module, at the top, left LED\",\n            \"dataType\": \"Bool\",\n            \"access\": \"WriteOnly\",\n            \"bitfield\": \"FrontPanelLeds/LedRed0Enable\"\n        },{\n            \"name\": \"NI.RedLED1\",\n            \"description-en\": \"one of 3 tri-colored LEDs (red/green/amber), controls red\",\n            \"documentation-en\": \"towards front of module, at the top, center LED\",\n            \"dataType\": \"Bool\",\n            \"access\": \"WriteOnly\",\n            \"bitfield\": \"FrontPanelLeds/LedRed1Enable\"\n        },{\n            \"name\": \"NI.RedLED2\",\n            \"description-en\": \"one of 3 tri-colored LEDs (red/green/amber), controls red\",\n            \"documentation-en\": \"towards front of module, at the top, right LED\",\n            \"dataType\": \"Bool\",\n            \"access\": \"WriteOnly\",\n            \"bitfield\": \"FrontPanelLeds/LedRed2Enable\"\n        },{\n            \"name\": \"NI.EventCounter0\",\n            \"dataType\": \"UInt32\",\n            \"access\": \"ReadWrite\",\n            \"bitfield\": \"EventCounter0/DelayInMilliseconds\",\n            \"max\": 255\n        },{\n            \"name\": \"NI.EventCounter1\",\n            \"dataType\": \"UInt32\",\n            \"access\": \"ReadWrite\",\n            \"bitfield\": \"EventCounter1/DelayInMilliseconds\",\n            \"max\": 255\n        },{\n            \"name\": \"NI.EventCounter2\",\n            \"dataType\": \"UInt32\",\n            \"access\": \"ReadWrite\",\n            \"bitfield\": \"EventCounter2/DelayInMilliseconds\",\n            \"max\": 255\n        },{\n            \"name\": \"NI.EventCounter3\",\n            \"dataType\": \"UInt32\",\n            \"access\": \"ReadWrite\",\n            \"bitfield\": \"EventCounter3/DelayInMilliseconds\",\n            \"max\": 255\n        },{\n            \"name\": \"NI.EventCounter0.DelayInMs\",\n            \"dataType\": \"UInt32\",\n            \"access\": \"ReadWrite\",\n            \"bitfield\": \"EventCounter0/DelayInMilliseconds\",\n            \"max\": 255\n        },{\n            \"name\": \"NI.EventCounter1.DelayInMs\",\n            \"dataType\": \"UInt32\",\n            \"access\": \"ReadWrite\",\n            \"bitfield\": \"EventCounter1/DelayInMilliseconds\",\n            \"max\": 255\n        },{\n            \"name\": \"NI.EventCounter2.DelayInMs\",\n            \"dataType\": \"UInt32\",\n            \"access\": \"ReadWrite\",\n            \"bitfield\": \"EventCounter2/DelayInMilliseconds\",\n            \"max\": 255\n        },{\n            \"name\": \"NI.EventCounter3.DelayInMs\",\n            \"dataType\": \"UInt32\",\n            \"access\": \"ReadWrite\",\n            \"bitfield\": \"EventCounter3/DelayInMilliseconds\",\n            \"max\": 255\n        },{\n            \"name\": \"NI.EventCounter0.DelayInSec\",\n            \"dataType\": \"Double\",\n            \"access\": \"ReadWrite\",\n            \"bitfield\": \"EventCounter0/DelayInMilliseconds\",\n            \"scale\": \"LinearMillisecondToSecond\",\n            \"min\": 0.0,\n            \"max\": 0.255\n        },{\n            \"name\": \"NI.EventCounter1.DelayInSec\",\n            \"dataType\": \"Double\",\n            \"access\": \"ReadWrite\",\n            \"bitfield\": \"EventCounter1/DelayInMilliseconds\",\n            \"scale\": \"LinearMillisecondToSecond\",\n            \"min\": 0.0,\n            \"max\": 0.255\n        },{\n            \"name\": \"NI.EventCounter2.DelayInSec\",\n            \"dataType\": \"Double\",\n            \"access\": \"ReadWrite\",\n            \"bitfield\": \"EventCounter2/DelayInMilliseconds\",\n            \"scale\": \"LinearMillisecondToSecond\",\n            \"min\": 0.0,\n            \"max\": 0.255\n        },{\n            \"name\": \"NI.EventCounter3.DelayInSec\",\n            \"dataType\": \"Double\",\n            \"access\": \"ReadWrite\",\n            \"bitfield\": \"EventCounter3/DelayInMilliseconds\",\n            \"scale\": \"LinearMillisecondToSecond\",\n            \"min\": 0.0,\n            \"max\": 0.255\n        },{\n            \"name\": \"NI.EventCounter0.DelayEnum\",\n            \"dataType\": \"NI.EventDelay\",\n            \"access\": \"ReadWrite\",\n            \"bitfield\": \"EventCounter0/DelayInMilliseconds\"\n        },{\n            \"name\": \"NI.EventCounter1.DelayEnum\",\n            \"dataType\": \"NI.EventDelay\",\n            \"access\": \"ReadWrite\",\n            \"bitfield\": \"EventCounter1/DelayInMilliseconds\"\n        },{\n            \"name\": \"NI.EventCounter2.DelayEnum\",\n            \"dataType\": \"NI.EventDelay\",\n            \"access\": \"ReadWrite\",\n            \"bitfield\": \"EventCounter2/DelayInMilliseconds\"\n        },{\n            \"name\": \"NI.EventCounter3.DelayEnum\",\n            \"dataType\": \"NI.EventDelay\",\n            \"access\": \"ReadWrite\",\n            \"bitfield\": \"EventCounter3/DelayInMilliseconds\"\n        },{\n            \"name\": \"NI.PropertyMinCapsSpecVerTest_OlderVersion\",\n            \"minCapsSpecVersion\" : 1,\n            \"dataType\": \"String\",\n            \"value\": \"PropertyMinCapsSpecVerTest\"\n        },{\n            \"name\": \"NI.PropertyMinCapsSpecVerTest_CurrentVersion\",\n            \"minCapsSpecVersion\" : 2,\n            \"dataType\": \"String\",\n            \"value\": \"PropertyMinCapsSpecVerTest\"\n        },{\n            \"name\": \"NI.PropertyMinCapsSpecVerTest_NewerVersion\",\n            \"minCapsSpecVersion\" : 3,\n            \"dataType\": \"String\",\n            \"value\": \"PropertyMinCapsSpecVerTest\"\n        },{\n            \"name\": \"NI.PropertyMaxCapsSpecVerTest_OlderVersion\",\n            \"maxCapsSpecVersion\" : 1,\n            \"dataType\": \"String\",\n            \"value\": \"PropertyMaxCapsSpecVerTest\"\n        },{\n            \"name\": \"NI.PropertyMaxCapsSpecVerTest_CurrentVersion\",\n            \"maxCapsSpecVersion\" : 2,\n            \"dataType\": \"String\",\n            \"value\": \"PropertyMaxCapsSpecVerTest\"\n        },{\n            \"name\": \"NI.PropertyMaxCapsSpecVerTest_NewerVersion\",\n            \"maxCapsSpecVersion\" : 3,\n            \"dataType\": \"String\",\n            \"value\": \"PropertyMaxCapsSpecVerTest\"\n        }]}") -> (0 "error out":errorcluster, 3 "Properties Array":string[](array[string]) caption="<JSON>Elements")   [LabVIEW 2018]
uses:
  <vilib>/JDP Science/JSONtext/String Subset.vi
  <vilib>/JDP Science/JSONtext/Parsing/Parse Full Path or Item Name.vi
  <vilib>/JDP Science/JSONtext/Offset/Find Item Locations by Path.vi
  <vilib>/JDP Science/JSONtext/JSONtext.lvlib
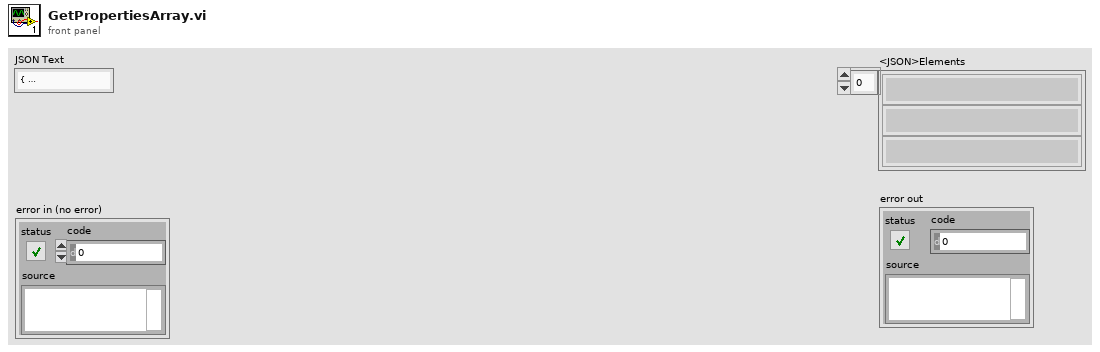
[diagram p1: front panel]
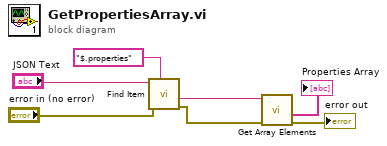
[diagram p0: block diagram]
diagram:
  n1 = call <vilib>:"Find Item.vi"("$Path or Item Name"="$.properties", "error in (no error)"="error in (no error)", "JSON"="JSON Text") -> ("error out"=w2:errorcluster, "<JSON>"=w5:string)  [unwired: 5 in, 2 out]
  n2 = call <vilib>:"Get Array Elements.vi"("error in (no error)"=w2, "JSON"=w5) -> ("error out"=→"error out":errorcluster, "<JSON>"=→"Properties Array":string[])  [unwired: 7 in, 1 out]
